vi "Motor driving.vi"(9 "New direction":string, 11 "Current direction":string) -> ()   [LabVIEW 2015]
uses:
  <vilib>/Platform/TimedLoop/XDataNode/timing_clust.ctl
  <vilib>/Platform/TimedLoop/XDataNode/nitl_modes.ctl
  <vilib>/Platform/TimedLoop/XDataNode/wakeup.ctl
  <vilib>/myRIO/Instrument Drivers/Onboard IO/PWM/typedefs/PWM Reference.ctl
  <vilib>/myRIO/Common/Instrument Driver Framework/Utilities/typedefs/myRIO Generic Hardware Reference.ctl
  <vilib>/myRIO/Common/Instrument Driver Framework/Utilities/typedefs/Hardware Version Enum.ctl
  <vilib>/myRIO/Common/Instrument Driver Framework/Utilities/typedefs/myRIO v1.0 Reference.ctl
  <vilib>/myRIO/Common/Instrument Driver Framework/Utilities/typedefs/Generic FPGA Reference.ctl
  <vilib>/myRIO/Common/Instrument Driver Framework/myRIO v1.0/PWM/typedefs/PWM Channels Enum.ctl
  <vilib>/myRIO/Instrument Drivers/Onboard IO/PWM/typedefs/PWM Configuration.ctl
  <vilib>/userdefined/High Color/nirio_resource_hc.ctl
  <vilib>/myRIO/Common/Instrument Driver Framework/Utilities/vis/Is FPGA Ref Available.vi
  <vilib>/myRIO/Common/Instrument Driver Framework/myRIO v1.0/PWM/vis/myRIO v1.1 Open PWM.vi
  <vilib>/myRIO/Instrument Drivers/Onboard IO/PWM/vis/Set Duty Cycle and Frequency.vi
  <vilib>/myRIO/Common/Instrument Driver Framework/Utilities/vis/Validate Channels.vi
  <vilib>/myRIO/Common/Instrument Driver Framework/myRIO v1.0/PWM/vis/myRIO v1.0 Reserve PWM.vi
  <vilib>/myRIO/Common/Instrument Driver Framework/myRIO v1.0/PWM/vis/myRIO v1.0 Build MUX Configuration PWM.vi
  <vilib>/myRIO/Common/Instrument Driver Framework/myRIO v1.0/Resource Manager/vis/myRIO v1.0 Reserve Channel List.vi
  <vilib>/myRIO/Common/Instrument Driver Framework/myRIO v1.0/Resource Manager/vis/myRIO v1.0 Create Configuration List.vi
  <vilib>/myRIO/Common/Instrument Driver Framework/myRIO v1.0/Resource Manager/vis/myRIO v1.0 Reserve Channel.vi
  <vilib>/myRIO/Common/Instrument Driver Framework/myRIO v1.0/Resource Manager/vis/myRIO v1.0 Unreserve Channel.vi
  <vilib>/myRIO/Common/Instrument Driver Framework/myRIO v1.0/Resource Manager/vis/myRIO v1.0 Build Mutex Name.vi
  <vilib>/Utility/VariantDataType/GetNumericInfo.vi
  <vilib>/Utility/error.llb/Error Cluster From Error Code.vi
  <vilib>/myRIO/Common/Instrument Driver Framework/myRIO v1.0/myRIO v1.1 Open.vi
  <vilib>/myRIO/Common/Instrument Driver Framework/Utilities/vis/IO Manager.vi
  <vilib>/myRIO/Common/Instrument Driver Framework/Utilities/vis/Configuration Manager.vi
  <vilib>/myRIO/Common/Instrument Driver Framework/myRIO v1.0/Resource Manager/vis/myRIO v1.0 Configure IO.vi
  <vilib>/myRIO/Common/Instrument Driver Framework/myRIO v1.0/myRIO v1.0 Close.vi
  <vilib>/myRIO/Common/Instrument Driver Framework/myRIO v1.0/PWM/vis/myRIO v1.0 Write PWM.vi
  <vilib>/platform/TimedLoop/XDataNode/XDataNode.xnode
  <vilib>/myRIO/Express VI/Onboard IO/PWM/PWM Express VI.xnode
  <vilib>/myRIO/Instrument Drivers/Onboard IO/PWM/vis/myRIO PWM Open.xnode
  <vilib>/Platform/TimedLoop/XDataNode/XDNodeRunTimeDep.lvlib
  <vilib>/myRIO/Instrument Drivers/Onboard IO/PWM/PWM.lvlib
panel:
  in  "Array":string[](array[string])
  out "left sped/right speed/time":dbl[][](array[numeric])
  out "Right":dbl=0.85
  out "Left":dbl=0.65
  out "Time":i32=2000
  out "error out 3":errorcluster
  out "error out 2":errorcluster
  in  "error in (no error) 2":errorcluster
  in  "error in (no error)":errorcluster
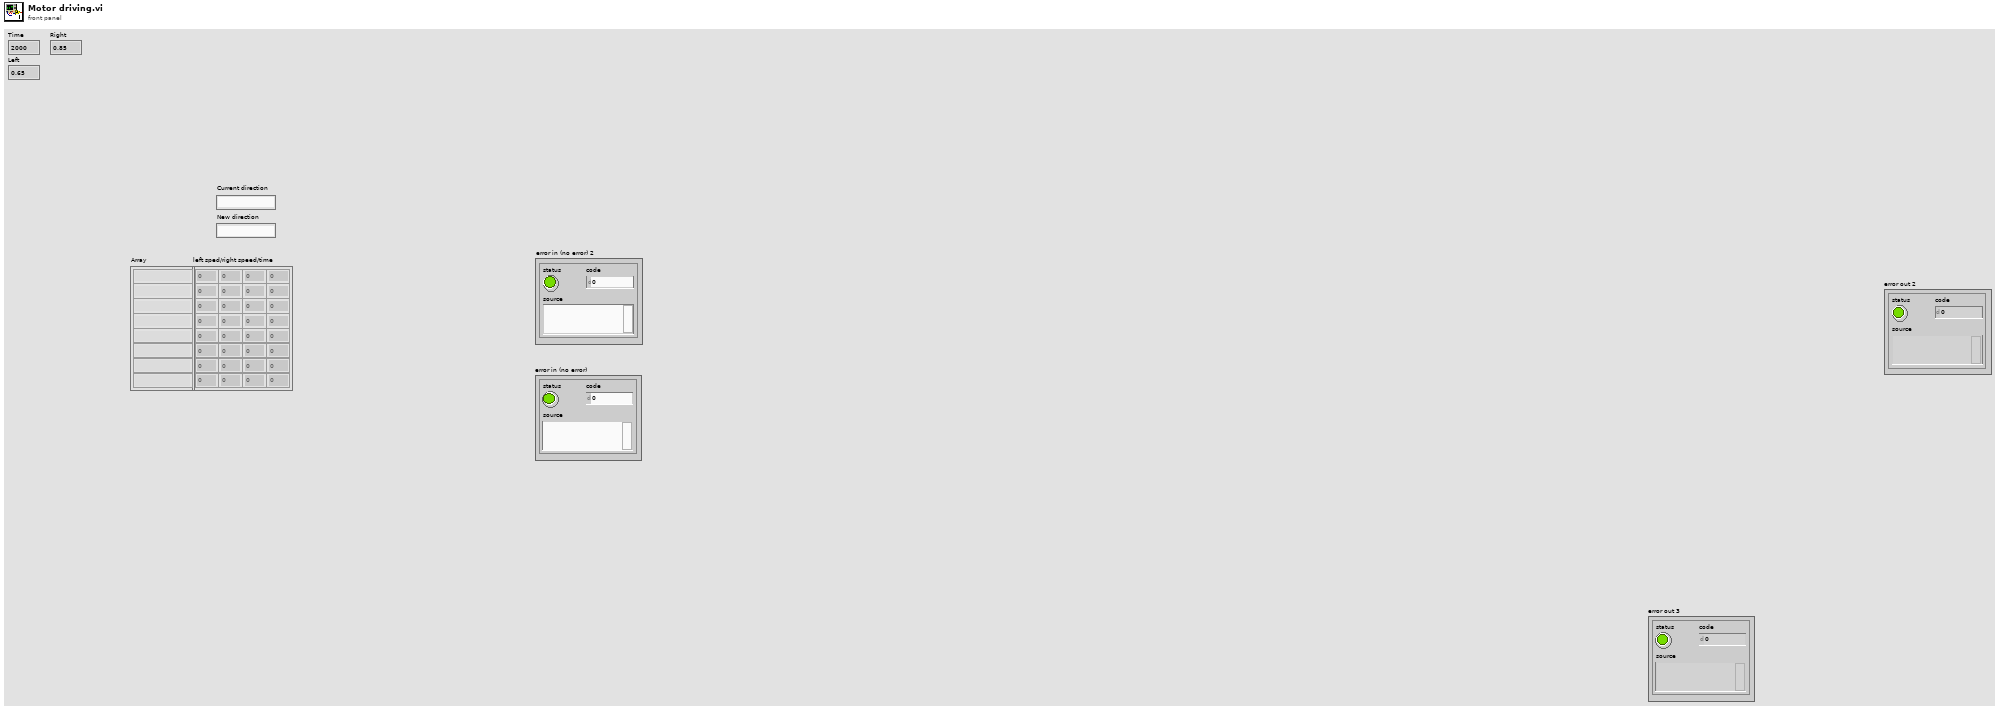
[diagram p1: front panel]
types:
  T1 = typedef "XDNodeRunTimeDep.lvlib/timing_clust.ctl" = cluster{"Expected End [f-1]":u64, "Actual End [f-1]":u64, "Finished Late? [f-1]":bool, "Expected End [i-1]":u64, "Actual End [i-1]":u64, "Finished Late? [i-1]":bool, "Expected Start [i]":u64, "Actual Start [i]":u64, "Expected Start [f]":u64, "Actual Start [f]":u64, "Source Name":string, "Structure Name":string, "Period":i64, "Deadline":i64, "Offset":i64, "Start":i64, "Priority":i32, "Timeout":i32, "Mode":T2, "Wakeup Reason":T3, "Error":errorcluster, "Source Type":string, "Secondary Source Type":string, "Global End Time":u64, "Global Start Time":u64, "Frame Duration":u64, "Iteration Duration":u64, "Assigned CPU":i32, "I/O Scan Engine Mode":u32}
  T2 = typedef "XDNodeRunTimeDep.lvlib/nitl_modes.ctl" = enum32{"No Change", "Process missed periods, maintain original phase", "Discard missed periods, maintain original phase", "Process missed periods, ignore original phase", "Discard missed periods, ignore original phase"}
  T3 = typedef "XDNodeRunTimeDep.lvlib/wakeup.ctl" = enum32{"Normal", "Aborted", "Asynchronous wakeup", "Timing source error", "Timed loop error", "Timeout"}
  T4 = typedef "PWM.lvlib/PWM Reference.ctl" = cluster{"myRIO Reference":T5, "PWM Channels Enum":T9, "PWM Configuration":T10}
  T5 = typedef "myRIO Generic Hardware Reference.ctl" = cluster{"myRIO Model":T6, "myRIO Hardware Reference":T7}
  T6 = typedef "Hardware Version Enum.ctl" = enum16{"Unknown", "myRIO-1900", "myRIO-1950", "roboRIO"}
  T7 = typedef "myRIO v1.0 Reference.ctl" = cluster{"Generic FPGA Reference":T8, "Allow multiple opens":bool}
  T8 = typedef "Generic FPGA Reference.ctl" = refnum<k20>
  T9 = typedef "PWM Channels Enum.ctl" = enum16{"Not Connected", "C/PWM0", "C/PWM1", "A/PWM0", "A/PWM1", "A/PWM2", "B/PWM0", "B/PWM1", "B/PWM2", "PWM/PWM0", "PWM/PWM1", "PWM/PWM2", "PWM/PWM3", "PWM/PWM4", "PWM/PWM5", "PWM/PWM6", "PWM/PWM7", "PWM/PWM8", "PWM/PWM9"}
  T10 = typedef "PWM.lvlib/PWM Configuration.ctl" = cluster{"Frequency":dbl, "Duty Cycle":dbl}
  T11 = typedef "nirio_resource_hc.ctl" = tag
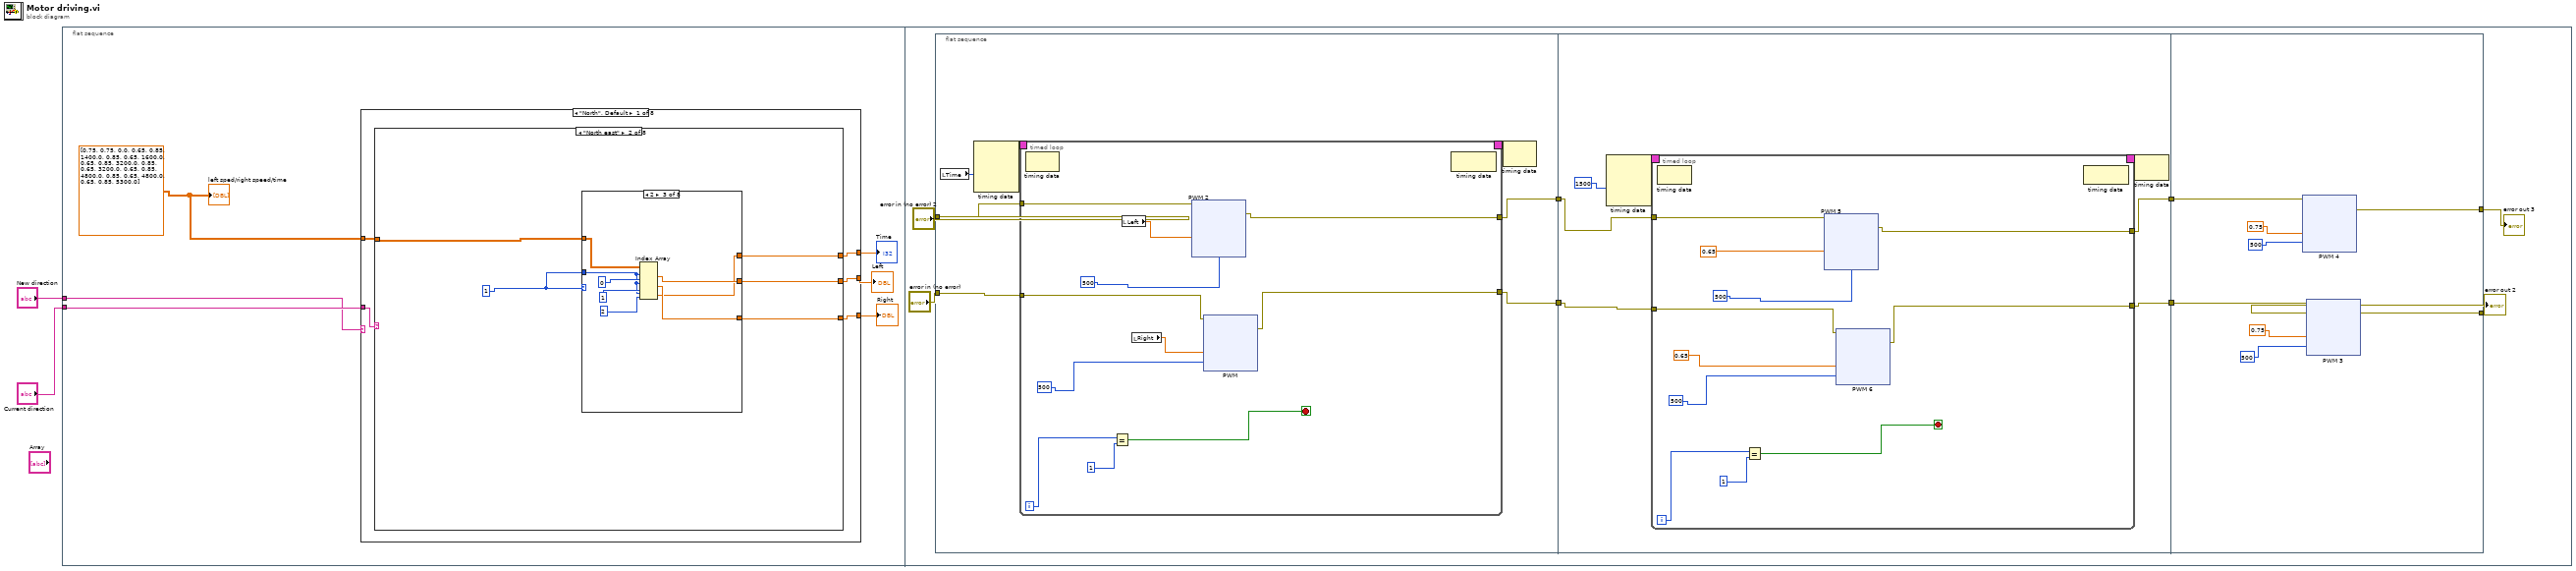
[diagram p0: block diagram]
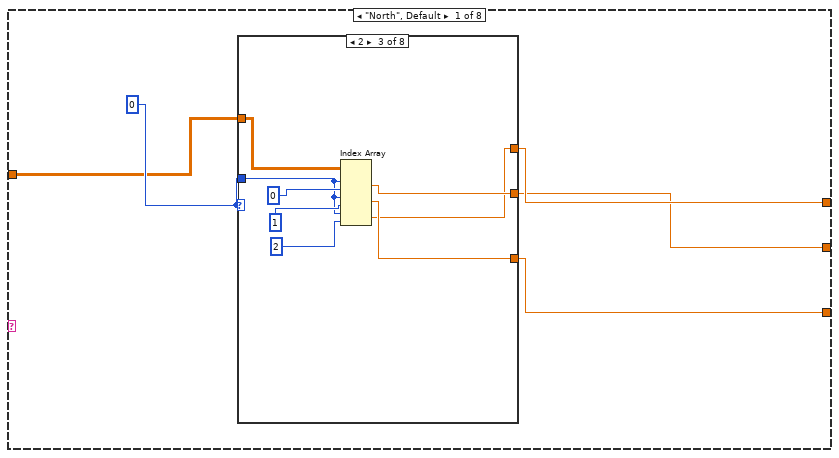
[diagram p2: hidden frame]
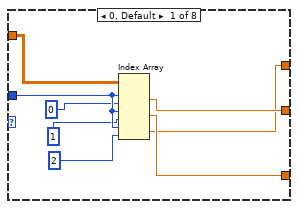
[diagram p3: hidden frame]
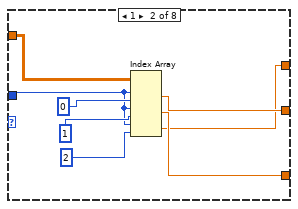
[diagram p4: hidden frame]
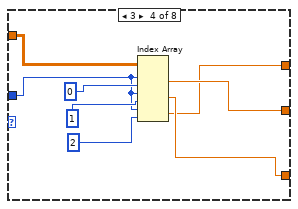
[diagram p5: hidden frame]
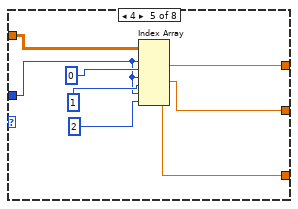
[diagram p6: hidden frame]
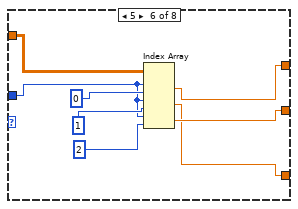
[diagram p7: hidden frame]
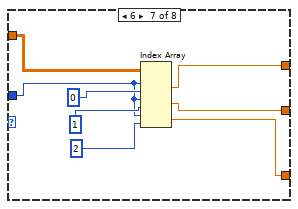
[diagram p8: hidden frame]
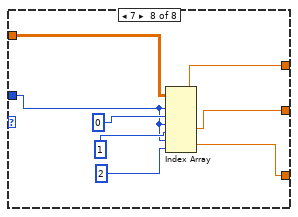
[diagram p9: hidden frame]
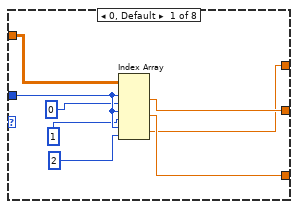
[diagram p10: hidden frame]
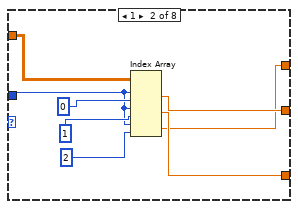
[diagram p11: hidden frame]
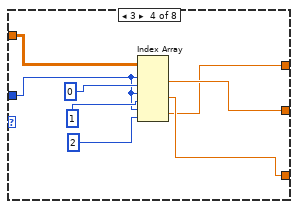
[diagram p12: hidden frame]
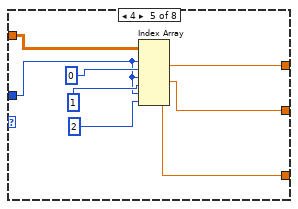
[diagram p13: hidden frame]
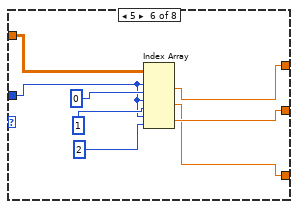
[diagram p14: hidden frame]
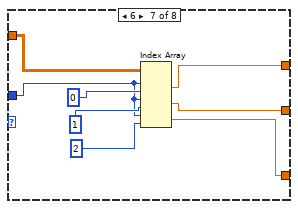
[diagram p15: hidden frame]
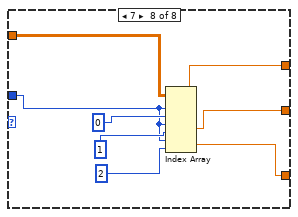
[diagram p16: hidden frame]
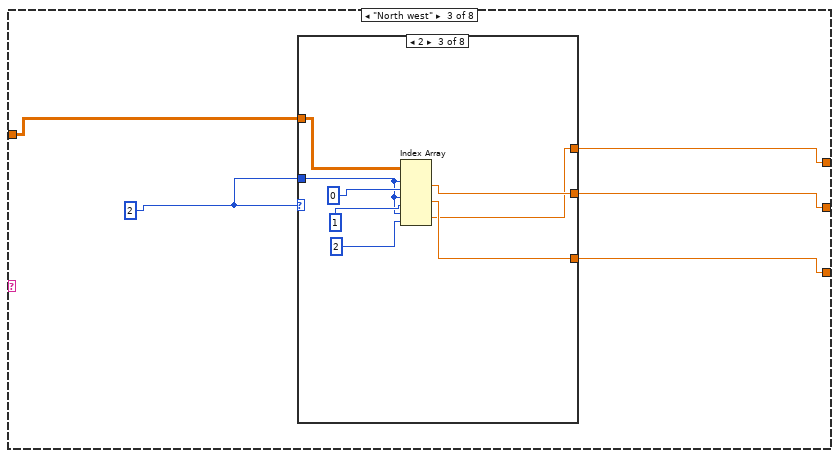
[diagram p17: hidden frame]
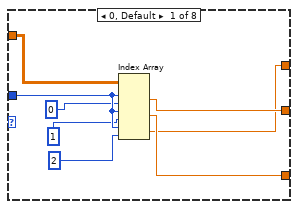
[diagram p18: hidden frame]
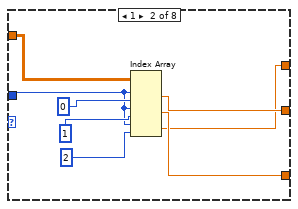
[diagram p19: hidden frame]
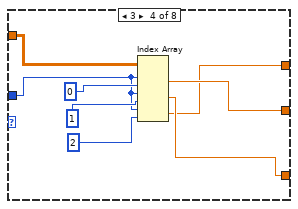
[diagram p20: hidden frame]
diagram:
  n1 = flat-sequence {
    tunnel: "Current direction" -> [w4]
    tunnel: "New direction" -> [w3]
    frame #0 {
      w5 = dbl[][] [[0.75, 0.75, 0.0], [0.65, 0.85, 1400.0], [0.85, 0.65, 1600.0], [0.65, 0.85, 3200.0], [0.85, 0.65, 3200.0], [0.65, 0.85, 4800.0], [0.85, 0.65, 4800.0], [0.65, 0.85, 5300.0]]
      n2 = case shown="\"North\", Default" w3 {
        tunnel: w4 -> [w9 w570 w1127 w1684 w2240 w2797 w3354 w3911]
        tunnel: [w12 w568 w1125 w1682 w2239 w2796 w3353 w3910] -> w8
        tunnel: [w11 w567 w1124 w1681 w2238 w2795 w3352 w3909] -> w7
        tunnel: [w10 w566 w1123 w1680 w2237 w2794 w3351 w3908] -> w6
        tunnel: w5 -> [w13 w569 w1126 w1683 w2241 w2798 w3355 w3912]
        frame "North", Default {
          n3 = case shown="\"North east\"" w9 {
            tunnel: [w17 w87 w155 w222 w292 w362 w430 w500] -> w12
            tunnel: [w16 w86 w154 w223 w291 w360 w429 w499] -> w11
            tunnel: [w15 w85 w153 w221 w290 w359 w428 w498] -> w10
            tunnel: w13 -> [w14 w83 w152 w224 w293 w361 w431 w497]
            frame "North", Default {
              w18 = 0
              n4 = case shown="2" w18 {
                tunnel: [w22 w28 w36 w44 w52 w61 w68 w77] -> w17
                tunnel: [w24 w30 w38 w45 w54 w63 w70 w79] -> w16
                tunnel: [w23 w29 w37 w46 w53 w62 w69 w78] -> w15
                tunnel: w18 -> [w26 w31 w39 w47 w55 w60 w71 w76]
                tunnel: w14 -> [w19 w27 w35 w43 w51 w59 w67 w75]
                frame 0, Default {
                  n5 = Index Array(array=w19, index (row) #1=w26, index (col) #1=0, index (row) #2=w26, index (col) #2=1, index (row) #3=w26, index (col) #3=2) -> (element #1=w24:dbl, element #2=w23:dbl, element #3=w22:dbl)
                }
                frame 1 {
                  n6 = Index Array(array=w27, index (row) #1=w31, index (col) #1=0, index (row) #2=w31, index (col) #2=1, index (row) #3=w31, index (col) #3=2) -> (element #1=w30:dbl, element #2=w29:dbl, element #3=w28:dbl)
                }
                frame 2 {
                  n7 = Index Array(array=w35, index (row) #1=w39, index (col) #1=0, index (row) #2=w39, index (col) #2=1, index (row) #3=w39, index (col) #3=2) -> (element #1=w38:dbl, element #2=w37:dbl, element #3=w36:dbl)
                }
                frame 3 {
                  n8 = Index Array(array=w43, index (row) #1=w47, index (col) #1=0, index (row) #2=w47, index (col) #2=1, index (row) #3=w47, index (col) #3=2) -> (element #1=w45:dbl, element #2=w46:dbl, element #3=w44:dbl)
                }
                frame 4 {
                  n9 = Index Array(array=w51, index (row) #1=w55, index (col) #1=0, index (row) #2=w55, index (col) #2=1, index (row) #3=w55, index (col) #3=2) -> (element #1=w52:dbl, element #2=w54:dbl, element #3=w53:dbl)
                }
                frame 5 {
                  n10 = Index Array(array=w59, index (row) #1=w60, index (col) #1=0, index (row) #2=w60, index (col) #2=1, index (row) #3=w60, index (col) #3=2) -> (element #1=w61:dbl, element #2=w62:dbl, element #3=w63:dbl)
                }
                frame 6 {
                  n11 = Index Array(array=w67, index (row) #1=w71, index (col) #1=0, index (row) #2=w71, index (col) #2=1, index (row) #3=w71, index (col) #3=2) -> (element #1=w68:dbl, element #2=w70:dbl, element #3=w69:dbl)
                }
                frame 7 {
                  n12 = Index Array(array=w75, index (row) #1=w76, index (col) #1=0, index (row) #2=w76, index (col) #2=1, index (row) #3=w76, index (col) #3=2) -> (element #1=w77:dbl, element #2=w79:dbl, element #3=w78:dbl)
                }
              }
            }
            frame "North east" {
              w84 = 1
              n13 = case shown="2" w84 {
                tunnel: [w91 w97 w105 w113 w121 w130 w137 w146] -> w87
                tunnel: [w93 w99 w107 w114 w123 w132 w139 w148] -> w86
                tunnel: [w92 w98 w106 w115 w122 w131 w138 w147] -> w85
                tunnel: w84 -> [w95 w100 w108 w116 w124 w129 w140 w145]
                tunnel: w83 -> [w88 w96 w104 w112 w120 w128 w136 w144]
                frame 0, Default {
                  n14 = Index Array(array=w88, index (row) #1=w95, index (col) #1=0, index (row) #2=w95, index (col) #2=1, index (row) #3=w95, index (col) #3=2) -> (element #1=w93:dbl, element #2=w92:dbl, element #3=w91:dbl)
                }
                frame 1 {
                  n15 = Index Array(array=w96, index (row) #1=w100, index (col) #1=0, index (row) #2=w100, index (col) #2=1, index (row) #3=w100, index (col) #3=2) -> (element #1=w99:dbl, element #2=w98:dbl, element #3=w97:dbl)
                }
                frame 2 {
                  n16 = Index Array(array=w104, index (row) #1=w108, index (col) #1=0, index (row) #2=w108, index (col) #2=1, index (row) #3=w108, index (col) #3=2) -> (element #1=w107:dbl, element #2=w106:dbl, element #3=w105:dbl)
                }
                frame 3 {
                  n17 = Index Array(array=w112, index (row) #1=w116, index (col) #1=0, index (row) #2=w116, index (col) #2=1, index (row) #3=w116, index (col) #3=2) -> (element #1=w114:dbl, element #2=w115:dbl, element #3=w113:dbl)
                }
                frame 4 {
                  n18 = Index Array(array=w120, index (row) #1=w124, index (col) #1=0, index (row) #2=w124, index (col) #2=1, index (row) #3=w124, index (col) #3=2) -> (element #1=w121:dbl, element #2=w123:dbl, element #3=w122:dbl)
                }
                frame 5 {
                  n19 = Index Array(array=w128, index (row) #1=w129, index (col) #1=0, index (row) #2=w129, index (col) #2=1, index (row) #3=w129, index (col) #3=2) -> (element #1=w130:dbl, element #2=w131:dbl, element #3=w132:dbl)
                }
                frame 6 {
                  n20 = Index Array(array=w136, index (row) #1=w140, index (col) #1=0, index (row) #2=w140, index (col) #2=1, index (row) #3=w140, index (col) #3=2) -> (element #1=w137:dbl, element #2=w139:dbl, element #3=w138:dbl)
                }
                frame 7 {
                  n21 = Index Array(array=w144, index (row) #1=w145, index (col) #1=0, index (row) #2=w145, index (col) #2=1, index (row) #3=w145, index (col) #3=2) -> (element #1=w146:dbl, element #2=w148:dbl, element #3=w147:dbl)
                }
              }
            }
            frame "North west" {
              w156 = 2
              n22 = case shown="2" w156 {
                tunnel: [w160 w166 w174 w182 w190 w199 w206 w215] -> w155
                tunnel: [w162 w168 w176 w183 w192 w201 w208 w217] -> w154
                tunnel: [w161 w167 w175 w184 w191 w200 w207 w216] -> w153
                tunnel: w156 -> [w164 w169 w177 w185 w193 w198 w209 w214]
                tunnel: w152 -> [w157 w165 w173 w181 w189 w197 w205 w213]
                frame 0, Default {
                  n23 = Index Array(array=w157, index (row) #1=w164, index (col) #1=0, index (row) #2=w164, index (col) #2=1, index (row) #3=w164, index (col) #3=2) -> (element #1=w162:dbl, element #2=w161:dbl, element #3=w160:dbl)
                }
                frame 1 {
                  n24 = Index Array(array=w165, index (row) #1=w169, index (col) #1=0, index (row) #2=w169, index (col) #2=1, index (row) #3=w169, index (col) #3=2) -> (element #1=w168:dbl, element #2=w167:dbl, element #3=w166:dbl)
                }
                frame 2 {
                  n25 = Index Array(array=w173, index (row) #1=w177, index (col) #1=0, index (row) #2=w177, index (col) #2=1, index (row) #3=w177, index (col) #3=2) -> (element #1=w176:dbl, element #2=w175:dbl, element #3=w174:dbl)
                }
                frame 3 {
                  n26 = Index Array(array=w181, index (row) #1=w185, index (col) #1=0, index (row) #2=w185, index (col) #2=1, index (row) #3=w185, index (col) #3=2) -> (element #1=w183:dbl, element #2=w184:dbl, element #3=w182:dbl)
                }
                frame 4 {
                  n27 = Index Array(array=w189, index (row) #1=w193, index (col) #1=0, index (row) #2=w193, index (col) #2=1, index (row) #3=w193, index (col) #3=2) -> (element #1=w190:dbl, element #2=w192:dbl, element #3=w191:dbl)
                }
                frame 5 {
                  n28 = Index Array(array=w197, index (row) #1=w198, index (col) #1=0, index (row) #2=w198, index (col) #2=1, index (row) #3=w198, index (col) #3=2) -> (element #1=w199:dbl, element #2=w200:dbl, element #3=w201:dbl)
                }
                frame 6 {
                  n29 = Index Array(array=w205, index (row) #1=w209, index (col) #1=0, index (row) #2=w209, index (col) #2=1, index (row) #3=w209, index (col) #3=2) -> (element #1=w206:dbl, element #2=w208:dbl, element #3=w207:dbl)
                }
                frame 7 {
                  n30 = Index Array(array=w213, index (row) #1=w214, index (col) #1=0, index (row) #2=w214, index (col) #2=1, index (row) #3=w214, index (col) #3=2) -> (element #1=w215:dbl, element #2=w217:dbl, element #3=w216:dbl)
                }
              }
            }
            frame "West" {
              w225 = 4
              n31 = case shown="2" w225 {
                tunnel: [w229 w235 w243 w251 w259 w268 w275 w284] -> w222
                tunnel: [w231 w237 w245 w252 w261 w270 w277 w286] -> w223
                tunnel: [w230 w236 w244 w253 w260 w269 w276 w285] -> w221
                tunnel: w225 -> [w233 w238 w246 w254 w262 w267 w278 w283]
                tunnel: w224 -> [w226 w234 w242 w250 w258 w266 w274 w282]
                frame 0, Default {
                  n32 = Index Array(array=w226, index (row) #1=w233, index (col) #1=0, index (row) #2=w233, index (col) #2=1, index (row) #3=w233, index (col) #3=2) -> (element #1=w231:dbl, element #2=w230:dbl, element #3=w229:dbl)
                }
                frame 1 {
                  n33 = Index Array(array=w234, index (row) #1=w238, index (col) #1=0, index (row) #2=w238, index (col) #2=1, index (row) #3=w238, index (col) #3=2) -> (element #1=w237:dbl, element #2=w236:dbl, element #3=w235:dbl)
                }
                frame 2 {
                  n34 = Index Array(array=w242, index (row) #1=w246, index (col) #1=0, index (row) #2=w246, index (col) #2=1, index (row) #3=w246, index (col) #3=2) -> (element #1=w245:dbl, element #2=w244:dbl, element #3=w243:dbl)
                }
                frame 3 {
                  n35 = Index Array(array=w250, index (row) #1=w254, index (col) #1=0, index (row) #2=w254, index (col) #2=1, index (row) #3=w254, index (col) #3=2) -> (element #1=w252:dbl, element #2=w253:dbl, element #3=w251:dbl)
                }
                frame 4 {
                  n36 = Index Array(array=w258, index (row) #1=w262, index (col) #1=0, index (row) #2=w262, index (col) #2=1, index (row) #3=w262, index (col) #3=2) -> (element #1=w259:dbl, element #2=w261:dbl, element #3=w260:dbl)
                }
                frame 5 {
                  n37 = Index Array(array=w266, index (row) #1=w267, index (col) #1=0, index (row) #2=w267, index (col) #2=1, index (row) #3=w267, index (col) #3=2) -> (element #1=w268:dbl, element #2=w269:dbl, element #3=w270:dbl)
                }
                frame 6 {
                  n38 = Index Array(array=w274, index (row) #1=w278, index (col) #1=0, index (row) #2=w278, index (col) #2=1, index (row) #3=w278, index (col) #3=2) -> (element #1=w275:dbl, element #2=w277:dbl, element #3=w276:dbl)
                }
                frame 7 {
                  n39 = Index Array(array=w282, index (row) #1=w283, index (col) #1=0, index (row) #2=w283, index (col) #2=1, index (row) #3=w283, index (col) #3=2) -> (element #1=w284:dbl, element #2=w286:dbl, element #3=w285:dbl)
                }
              }
            }
            frame "East" {
              w294 = 3
              n40 = case shown="2" w294 {
                tunnel: [w298 w304 w312 w320 w328 w337 w344 w353] -> w292
                tunnel: [w300 w306 w314 w321 w330 w339 w346 w355] -> w291
                tunnel: [w299 w305 w313 w322 w329 w338 w345 w354] -> w290
                tunnel: w294 -> [w302 w307 w315 w323 w331 w336 w347 w352]
                tunnel: w293 -> [w295 w303 w311 w319 w327 w335 w343 w351]
                frame 0, Default {
                  n41 = Index Array(array=w295, index (row) #1=w302, index (col) #1=0, index (row) #2=w302, index (col) #2=1, index (row) #3=w302, index (col) #3=2) -> (element #1=w300:dbl, element #2=w299:dbl, element #3=w298:dbl)
                }
                frame 1 {
                  n42 = Index Array(array=w303, index (row) #1=w307, index (col) #1=0, index (row) #2=w307, index (col) #2=1, index (row) #3=w307, index (col) #3=2) -> (element #1=w306:dbl, element #2=w305:dbl, element #3=w304:dbl)
                }
                frame 2 {
                  n43 = Index Array(array=w311, index (row) #1=w315, index (col) #1=0, index (row) #2=w315, index (col) #2=1, index (row) #3=w315, index (col) #3=2) -> (element #1=w314:dbl, element #2=w313:dbl, element #3=w312:dbl)
                }
                frame 3 {
                  n44 = Index Array(array=w319, index (row) #1=w323, index (col) #1=0, index (row) #2=w323, index (col) #2=1, index (row) #3=w323, index (col) #3=2) -> (element #1=w321:dbl, element #2=w322:dbl, element #3=w320:dbl)
                }
                frame 4 {
                  n45 = Index Array(array=w327, index (row) #1=w331, index (col) #1=0, index (row) #2=w331, index (col) #2=1, index (row) #3=w331, index (col) #3=2) -> (element #1=w328:dbl, element #2=w330:dbl, element #3=w329:dbl)
                }
                frame 5 {
                  n46 = Index Array(array=w335, index (row) #1=w336, index (col) #1=0, index (row) #2=w336, index (col) #2=1, index (row) #3=w336, index (col) #3=2) -> (element #1=w337:dbl, element #2=w338:dbl, element #3=w339:dbl)
                }
                frame 6 {
                  n47 = Index Array(array=w343, index (row) #1=w347, index (col) #1=0, index (row) #2=w347, index (col) #2=1, index (row) #3=w347, index (col) #3=2) -> (element #1=w344:dbl, element #2=w346:dbl, element #3=w345:dbl)
                }
                frame 7 {
                  n48 = Index Array(array=w351, index (row) #1=w352, index (col) #1=0, index (row) #2=w352, index (col) #2=1, index (row) #3=w352, index (col) #3=2) -> (element #1=w353:dbl, element #2=w355:dbl, element #3=w354:dbl)
                }
              }
            }
            frame "South" {
              w363 = 7
              n49 = case shown="2" w363 {
                tunnel: [w367 w373 w381 w389 w397 w406 w413 w422] -> w362
                tunnel: [w369 w375 w383 w390 w399 w408 w415 w424] -> w360
                tunnel: [w368 w374 w382 w391 w398 w407 w414 w423] -> w359
                tunnel: w363 -> [w371 w376 w384 w392 w400 w405 w416 w421]
                tunnel: w361 -> [w364 w372 w380 w388 w396 w404 w412 w420]
                frame 0, Default {
                  n50 = Index Array(array=w364, index (row) #1=w371, index (col) #1=0, index (row) #2=w371, index (col) #2=1, index (row) #3=w371, index (col) #3=2) -> (element #1=w369:dbl, element #2=w368:dbl, element #3=w367:dbl)
                }
                frame 1 {
                  n51 = Index Array(array=w372, index (row) #1=w376, index (col) #1=0, index (row) #2=w376, index (col) #2=1, index (row) #3=w376, index (col) #3=2) -> (element #1=w375:dbl, element #2=w374:dbl, element #3=w373:dbl)
                }
                frame 2 {
                  n52 = Index Array(array=w380, index (row) #1=w384, index (col) #1=0, index (row) #2=w384, index (col) #2=1, index (row) #3=w384, index (col) #3=2) -> (element #1=w383:dbl, element #2=w382:dbl, element #3=w381:dbl)
                }
                frame 3 {
                  n53 = Index Array(array=w388, index (row) #1=w392, index (col) #1=0, index (row) #2=w392, index (col) #2=1, index (row) #3=w392, index (col) #3=2) -> (element #1=w390:dbl, element #2=w391:dbl, element #3=w389:dbl)
                }
                frame 4 {
                  n54 = Index Array(array=w396, index (row) #1=w400, index (col) #1=0, index (row) #2=w400, index (col) #2=1, index (row) #3=w400, index (col) #3=2) -> (element #1=w397:dbl, element #2=w399:dbl, element #3=w398:dbl)
                }
                frame 5 {
                  n55 = Index Array(array=w404, index (row) #1=w405, index (col) #1=0, index (row) #2=w405, index (col) #2=1, index (row) #3=w405, index (col) #3=2) -> (element #1=w406:dbl, element #2=w407:dbl, element #3=w408:dbl)
                }
                frame 6 {
                  n56 = Index Array(array=w412, index (row) #1=w416, index (col) #1=0, index (row) #2=w416, index (col) #2=1, index (row) #3=w416, index (col) #3=2) -> (element #1=w413:dbl, element #2=w415:dbl, element #3=w414:dbl)
                }
                frame 7 {
                  n57 = Index Array(array=w420, index (row) #1=w421, index (col) #1=0, index (row) #2=w421, index (col) #2=1, index (row) #3=w421, index (col) #3=2) -> (element #1=w422:dbl, element #2=w424:dbl, element #3=w423:dbl)
                }
              }
            }
            frame "South west" {
              w432 = 6
              n58 = case shown="2" w432 {
                tunnel: [w436 w442 w450 w458 w466 w475 w482 w491] -> w430
                tunnel: [w438 w444 w452 w459 w468 w477 w484 w493] -> w429
                tunnel: [w437 w443 w451 w460 w467 w476 w483 w492] -> w428
                tunnel: w432 -> [w440 w445 w453 w461 w469 w474 w485 w490]
                tunnel: w431 -> [w433 w441 w449 w457 w465 w473 w481 w489]
                frame 0, Default {
                  n59 = Index Array(array=w433, index (row) #1=w440, index (col) #1=0, index (row) #2=w440, index (col) #2=1, index (row) #3=w440, index (col) #3=2) -> (element #1=w438:dbl, element #2=w437:dbl, element #3=w436:dbl)
                }
                frame 1 {
                  n60 = Index Array(array=w441, index (row) #1=w445, index (col) #1=0, index (row) #2=w445, index (col) #2=1, index (row) #3=w445, index (col) #3=2) -> (element #1=w444:dbl, element #2=w443:dbl, element #3=w442:dbl)
                }
                frame 2 {
                  n61 = Index Array(array=w449, index (row) #1=w453, index (col) #1=0, index (row) #2=w453, index (col) #2=1, index (row) #3=w453, index (col) #3=2) -> (element #1=w452:dbl, element #2=w451:dbl, element #3=w450:dbl)
                }
                frame 3 {
                  n62 = Index Array(array=w457, index (row) #1=w461, index (col) #1=0, index (row) #2=w461, index (col) #2=1, index (row) #3=w461, index (col) #3=2) -> (element #1=w459:dbl, element #2=w460:dbl, element #3=w458:dbl)
                }
                frame 4 {
                  n63 = Index Array(array=w465, index (row) #1=w469, index (col) #1=0, index (row) #2=w469, index (col) #2=1, index (row) #3=w469, index (col) #3=2) -> (element #1=w466:dbl, element #2=w468:dbl, element #3=w467:dbl)
                }
                frame 5 {
                  n64 = Index Array(array=w473, index (row) #1=w474, index (col) #1=0, index (row) #2=w474, index (col) #2=1, index (row) #3=w474, index (col) #3=2) -> (element #1=w475:dbl, element #2=w476:dbl, element #3=w477:dbl)
                }
                frame 6 {
                  n65 = Index Array(array=w481, index (row) #1=w485, index (col) #1=0, index (row) #2=w485, index (col) #2=1, index (row) #3=w485, index (col) #3=2) -> (element #1=w482:dbl, element #2=w484:dbl, element #3=w483:dbl)
                }
                frame 7 {
                  n66 = Index Array(array=w489, index (row) #1=w490, index (col) #1=0, index (row) #2=w490, index (col) #2=1, index (row) #3=w490, index (col) #3=2) -> (element #1=w491:dbl, element #2=w493:dbl, element #3=w492:dbl)
                }
              }
            }
            frame "South east" {
              w501 = 5
              n67 = case shown="2" w501 {
                tunnel: [w505 w511 w519 w527 w535 w544 w551 w560] -> w500
                tunnel: [w507 w513 w521 w528 w537 w546 w553 w562] -> w499
                tunnel: [w506 w512 w520 w529 w536 w545 w552 w561] -> w498
                tunnel: w501 -> [w509 w514 w522 w530 w538 w543 w554 w559]
                tunnel: w497 -> [w502 w510 w518 w526 w534 w542 w550 w558]
                frame 0, Default {
                  n68 = Index Array(array=w502, index (row) #1=w509, index (col) #1=0, index (row) #2=w509, index (col) #2=1, index (row) #3=w509, index (col) #3=2) -> (element #1=w507:dbl, element #2=w506:dbl, element #3=w505:dbl)
                }
                frame 1 {
                  n69 = Index Array(array=w510, index (row) #1=w514, index (col) #1=0, index (row) #2=w514, index (col) #2=1, index (row) #3=w514, index (col) #3=2) -> (element #1=w513:dbl, element #2=w512:dbl, element #3=w511:dbl)
                }
                frame 2 {
                  n70 = Index Array(array=w518, index (row) #1=w522, index (col) #1=0, index (row) #2=w522, index (col) #2=1, index (row) #3=w522, index (col) #3=2) -> (element #1=w521:dbl, element #2=w520:dbl, element #3=w519:dbl)
                }
                frame 3 {
                  n71 = Index Array(array=w526, index (row) #1=w530, index (col) #1=0, index (row) #2=w530, index (col) #2=1, index (row) #3=w530, index (col) #3=2) -> (element #1=w528:dbl, element #2=w529:dbl, element #3=w527:dbl)
                }
                frame 4 {
                  n72 = Index Array(array=w534, index (row) #1=w538, index (col) #1=0, index (row) #2=w538, index (col) #2=1, index (row) #3=w538, index (col) #3=2) -> (element #1=w535:dbl, element #2=w537:dbl, element #3=w536:dbl)
                }
                frame 5 {
                  n73 = Index Array(array=w542, index (row) #1=w543, index (col) #1=0, index (row) #2=w543, index (col) #2=1, index (row) #3=w543, index (col) #3=2) -> (element #1=w544:dbl, element #2=w545:dbl, element #3=w546:dbl)
                }
                frame 6 {
                  n74 = Index Array(array=w550, index (row) #1=w554, index (col) #1=0, index (row) #2=w554, index (col) #2=1, index (row) #3=w554, index (col) #3=2) -> (element #1=w551:dbl, element #2=w553:dbl, element #3=w552:dbl)
                }
                frame 7 {
                  n75 = Index Array(array=w558, index (row) #1=w559, index (col) #1=0, index (row) #2=w559, index (col) #2=1, index (row) #3=w559, index (col) #3=2) -> (element #1=w560:dbl, element #2=w562:dbl, element #3=w561:dbl)
                }
              }
            }
          }
        }
        frame "North east" {
          n76 = case shown="\"North\", Default" w570 {
            tunnel: [w574 w644 w712 w779 w849 w919 w987 w1057] -> w568
            tunnel: [w573 w643 w711 w780 w848 w917 w986 w1056] -> w567
            tunnel: [w572 w642 w710 w778 w847 w916 w985 w1055] -> w566
            tunnel: w569 -> [w571 w640 w709 w781 w850 w918 w988 w1054]
            frame "North", Default {
              w575 = 2
              n77 = case shown="2" w575 {
                tunnel: [w579 w585 w593 w601 w609 w618 w625 w634] -> w574
                tunnel: [w581 w587 w595 w602 w611 w620 w627 w636] -> w573
                tunnel: [w580 w586 w594 w603 w610 w619 w626 w635] -> w572
                tunnel: w575 -> [w583 w588 w596 w604 w612 w617 w628 w633]
                tunnel: w571 -> [w576 w584 w592 w600 w608 w616 w624 w632]
                frame 0, Default {
                  n78 = Index Array(array=w576, index (row) #1=w583, index (col) #1=0, index (row) #2=w583, index (col) #2=1, index (row) #3=w583, index (col) #3=2) -> (element #1=w581:dbl, element #2=w580:dbl, element #3=w579:dbl)
                }
                frame 1 {
                  n79 = Index Array(array=w584, index (row) #1=w588, index (col) #1=0, index (row) #2=w588, index (col) #2=1, index (row) #3=w588, index (col) #3=2) -> (element #1=w587:dbl, element #2=w586:dbl, element #3=w585:dbl)
                }
                frame 2 {
                  n80 = Index Array(array=w592, index (row) #1=w596, index (col) #1=0, index (row) #2=w596, index (col) #2=1, index (row) #3=w596, index (col) #3=2) -> (element #1=w595:dbl, element #2=w594:dbl, element #3=w593:dbl)
                }
                frame 3 {
                  n81 = Index Array(array=w600, index (row) #1=w604, index (col) #1=0, index (row) #2=w604, index (col) #2=1, index (row) #3=w604, index (col) #3=2) -> (element #1=w602:dbl, element #2=w603:dbl, element #3=w601:dbl)
                }
                frame 4 {
                  n82 = Index Array(array=w608, index (row) #1=w612, index (col) #1=0, index (row) #2=w612, index (col) #2=1, index (row) #3=w612, index (col) #3=2) -> (element #1=w609:dbl, element #2=w611:dbl, element #3=w610:dbl)
                }
                frame 5 {
                  n83 = Index Array(array=w616, index (row) #1=w617, index (col) #1=0, index (row) #2=w617, index (col) #2=1, index (row) #3=w617, index (col) #3=2) -> (element #1=w618:dbl, element #2=w619:dbl, element #3=w620:dbl)
                }
                frame 6 {
                  n84 = Index Array(array=w624, index (row) #1=w628, index (col) #1=0, index (row) #2=w628, index (col) #2=1, index (row) #3=w628, index (col) #3=2) -> (element #1=w625:dbl, element #2=w627:dbl, element #3=w626:dbl)
                }
                frame 7 {
                  n85 = Index Array(array=w632, index (row) #1=w633, index (col) #1=0, index (row) #2=w633, index (col) #2=1, index (row) #3=w633, index (col) #3=2) -> (element #1=w634:dbl, element #2=w636:dbl, element #3=w635:dbl)
                }
              }
            }
            frame "North east" {
              w641 = 0
              n86 = case shown="2" w641 {
                tunnel: [w648 w654 w662 w670 w678 w687 w694 w703] -> w644
                tunnel: [w650 w656 w664 w671 w680 w689 w696 w705] -> w643
                tunnel: [w649 w655 w663 w672 w679 w688 w695 w704] -> w642
                tunnel: w641 -> [w652 w657 w665 w673 w681 w686 w697 w702]
                tunnel: w640 -> [w645 w653 w661 w669 w677 w685 w693 w701]
                frame 0, Default {
                  n87 = Index Array(array=w645, index (row) #1=w652, index (col) #1=0, index (row) #2=w652, index (col) #2=1, index (row) #3=w652, index (col) #3=2) -> (element #1=w650:dbl, element #2=w649:dbl, element #3=w648:dbl)
                }
                frame 1 {
                  n88 = Index Array(array=w653, index (row) #1=w657, index (col) #1=0, index (row) #2=w657, index (col) #2=1, index (row) #3=w657, index (col) #3=2) -> (element #1=w656:dbl, element #2=w655:dbl, element #3=w654:dbl)
                }
                frame 2 {
                  n89 = Index Array(array=w661, index (row) #1=w665, index (col) #1=0, index (row) #2=w665, index (col) #2=1, index (row) #3=w665, index (col) #3=2) -> (element #1=w664:dbl, element #2=w663:dbl, element #3=w662:dbl)
                }
                frame 3 {
                  n90 = Index Array(array=w669, index (row) #1=w673, index (col) #1=0, index (row) #2=w673, index (col) #2=1, index (row) #3=w673, index (col) #3=2) -> (element #1=w671:dbl, element #2=w672:dbl, element #3=w670:dbl)
                }
                frame 4 {
                  n91 = Index Array(array=w677, index (row) #1=w681, index (col) #1=0, index (row) #2=w681, index (col) #2=1, index (row) #3=w681, index (col) #3=2) -> (element #1=w678:dbl, element #2=w680:dbl, element #3=w679:dbl)
                }
                frame 5 {
                  n92 = Index Array(array=w685, index (row) #1=w686, index (col) #1=0, index (row) #2=w686, index (col) #2=1, index (row) #3=w686, index (col) #3=2) -> (element #1=w687:dbl, element #2=w688:dbl, element #3=w689:dbl)
                }
                frame 6 {
                  n93 = Index Array(array=w693, index (row) #1=w697, index (col) #1=0, index (row) #2=w697, index (col) #2=1, index (row) #3=w697, index (col) #3=2) -> (element #1=w694:dbl, element #2=w696:dbl, element #3=w695:dbl)
                }
                frame 7 {
                  n94 = Index Array(array=w701, index (row) #1=w702, index (col) #1=0, index (row) #2=w702, index (col) #2=1, index (row) #3=w702, index (col) #3=2) -> (element #1=w703:dbl, element #2=w705:dbl, element #3=w704:dbl)
                }
              }
            }
            frame "North west" {
              w713 = 4
              n95 = case shown="2" w713 {
                tunnel: [w717 w723 w731 w739 w747 w756 w763 w772] -> w712
                tunnel: [w719 w725 w733 w740 w749 w758 w765 w774] -> w711
                tunnel: [w718 w724 w732 w741 w748 w757 w764 w773] -> w710
                tunnel: w713 -> [w721 w726 w734 w742 w750 w755 w766 w771]
                tunnel: w709 -> [w714 w722 w730 w738 w746 w754 w762 w770]
                frame 0, Default {
                  n96 = Index Array(array=w714, index (row) #1=w721, index (col) #1=0, index (row) #2=w721, index (col) #2=1, index (row) #3=w721, index (col) #3=2) -> (element #1=w719:dbl, element #2=w718:dbl, element #3=w717:dbl)
                }
                frame 1 {
                  n97 = Index Array(array=w722, index (row) #1=w726, index (col) #1=0, index (row) #2=w726, index (col) #2=1, index (row) #3=w726, index (col) #3=2) -> (element #1=w725:dbl, element #2=w724:dbl, element #3=w723:dbl)
                }
                frame 2 {
                  n98 = Index Array(array=w730, index (row) #1=w734, index (col) #1=0, index (row) #2=w734, index (col) #2=1, index (row) #3=w734, index (col) #3=2) -> (element #1=w733:dbl, element #2=w732:dbl, element #3=w731:dbl)
                }
                frame 3 {
                  n99 = Index Array(array=w738, index (row) #1=w742, index (col) #1=0, index (row) #2=w742, index (col) #2=1, index (row) #3=w742, index (col) #3=2) -> (element #1=w740:dbl, element #2=w741:dbl, element #3=w739:dbl)
                }
                frame 4 {
                  n100 = Index Array(array=w746, index (row) #1=w750, index (col) #1=0, index (row) #2=w750, index (col) #2=1, index (row) #3=w750, index (col) #3=2) -> (element #1=w747:dbl, element #2=w749:dbl, element #3=w748:dbl)
                }
                frame 5 {
                  n101 = Index Array(array=w754, index (row) #1=w755, index (col) #1=0, index (row) #2=w755, index (col) #2=1, index (row) #3=w755, index (col) #3=2) -> (element #1=w756:dbl, element #2=w757:dbl, element #3=w758:dbl)
                }
                frame 6 {
                  n102 = Index Array(array=w762, index (row) #1=w766, index (col) #1=0, index (row) #2=w766, index (col) #2=1, index (row) #3=w766, index (col) #3=2) -> (element #1=w763:dbl, element #2=w765:dbl, element #3=w764:dbl)
                }
                frame 7 {
                  n103 = Index Array(array=w770, index (row) #1=w771, index (col) #1=0, index (row) #2=w771, index (col) #2=1, index (row) #3=w771, index (col) #3=2) -> (element #1=w772:dbl, element #2=w774:dbl, element #3=w773:dbl)
                }
              }
            }
            frame "West" {
              w782 = 6
              n104 = case shown="2" w782 {
                tunnel: [w786 w792 w800 w808 w816 w825 w832 w841] -> w779
                tunnel: [w788 w794 w802 w809 w818 w827 w834 w843] -> w780
                tunnel: [w787 w793 w801 w810 w817 w826 w833 w842] -> w778
                tunnel: w782 -> [w790 w795 w803 w811 w819 w824 w835 w840]
                tunnel: w781 -> [w783 w791 w799 w807 w815 w823 w831 w839]
                frame 0, Default {
                  n105 = Index Array(array=w783, index (row) #1=w790, index (col) #1=0, index (row) #2=w790, index (col) #2=1, index (row) #3=w790, index (col) #3=2) -> (element #1=w788:dbl, element #2=w787:dbl, element #3=w786:dbl)
                }
                frame 1 {
                  n106 = Index Array(array=w791, index (row) #1=w795, index (col) #1=0, index (row) #2=w795, index (col) #2=1, index (row) #3=w795, index (col) #3=2) -> (element #1=w794:dbl, element #2=w793:dbl, element #3=w792:dbl)
                }
                frame 2 {
                  n107 = Index Array(array=w799, index (row) #1=w803, index (col) #1=0, index (row) #2=w803, index (col) #2=1, index (row) #3=w803, index (col) #3=2) -> (element #1=w802:dbl, element #2=w801:dbl, element #3=w800:dbl)
                }
                frame 3 {
                  n108 = Index Array(array=w807, index (row) #1=w811, index (col) #1=0, index (row) #2=w811, index (col) #2=1, index (row) #3=w811, index (col) #3=2) -> (element #1=w809:dbl, element #2=w810:dbl, element #3=w808:dbl)
                }
                frame 4 {
                  n109 = Index Array(array=w815, index (row) #1=w819, index (col) #1=0, index (row) #2=w819, index (col) #2=1, index (row) #3=w819, index (col) #3=2) -> (element #1=w816:dbl, element #2=w818:dbl, element #3=w817:dbl)
                }
                frame 5 {
                  n110 = Index Array(array=w823, index (row) #1=w824, index (col) #1=0, index (row) #2=w824, index (col) #2=1, index (row) #3=w824, index (col) #3=2) -> (element #1=w825:dbl, element #2=w826:dbl, element #3=w827:dbl)
                }
                frame 6 {
                  n111 = Index Array(array=w831, index (row) #1=w835, index (col) #1=0, index (row) #2=w835, index (col) #2=1, index (row) #3=w835, index (col) #3=2) -> (element #1=w832:dbl, element #2=w834:dbl, element #3=w833:dbl)
                }
                frame 7 {
                  n112 = Index Array(array=w839, index (row) #1=w840, index (col) #1=0, index (row) #2=w840, index (col) #2=1, index (row) #3=w840, index (col) #3=2) -> (element #1=w841:dbl, element #2=w843:dbl, element #3=w842:dbl)
                }
              }
            }
            frame "East" {
              w851 = 1
              n113 = case shown="2" w851 {
                tunnel: [w855 w861 w869 w877 w885 w894 w901 w910] -> w849
                tunnel: [w857 w863 w871 w878 w887 w896 w903 w912] -> w848
                tunnel: [w856 w862 w870 w879 w886 w895 w902 w911] -> w847
                tunnel: w851 -> [w859 w864 w872 w880 w888 w893 w904 w909]
                tunnel: w850 -> [w852 w860 w868 w876 w884 w892 w900 w908]
                frame 0, Default {
                  n114 = Index Array(array=w852, index (row) #1=w859, index (col) #1=0, index (row) #2=w859, index (col) #2=1, index (row) #3=w859, index (col) #3=2) -> (element #1=w857:dbl, element #2=w856:dbl, element #3=w855:dbl)
                }
                frame 1 {
                  n115 = Index Array(array=w860, index (row) #1=w864, index (col) #1=0, index (row) #2=w864, index (col) #2=1, index (row) #3=w864, index (col) #3=2) -> (element #1=w863:dbl, element #2=w862:dbl, element #3=w861:dbl)
                }
                frame 2 {
                  n116 = Index Array(array=w868, index (row) #1=w872, index (col) #1=0, index (row) #2=w872, index (col) #2=1, index (row) #3=w872, index (col) #3=2) -> (element #1=w871:dbl, element #2=w870:dbl, element #3=w869:dbl)
                }
                frame 3 {
                  n117 = Index Array(array=w876, index (row) #1=w880, index (col) #1=0, index (row) #2=w880, index (col) #2=1, index (row) #3=w880, index (col) #3=2) -> (element #1=w878:dbl, element #2=w879:dbl, element #3=w877:dbl)
                }
                frame 4 {
                  n118 = Index Array(array=w884, index (row) #1=w888, index (col) #1=0, index (row) #2=w888, index (col) #2=1, index (row) #3=w888, index (col) #3=2) -> (element #1=w885:dbl, element #2=w887:dbl, element #3=w886:dbl)
                }
                frame 5 {
                  n119 = Index Array(array=w892, index (row) #1=w893, index (col) #1=0, index (row) #2=w893, index (col) #2=1, index (row) #3=w893, index (col) #3=2) -> (element #1=w894:dbl, element #2=w895:dbl, element #3=w896:dbl)
                }
                frame 6 {
                  n120 = Index Array(array=w900, index (row) #1=w904, index (col) #1=0, index (row) #2=w904, index (col) #2=1, index (row) #3=w904, index (col) #3=2) -> (element #1=w901:dbl, element #2=w903:dbl, element #3=w902:dbl)
                }
                frame 7 {
                  n121 = Index Array(array=w908, index (row) #1=w909, index (col) #1=0, index (row) #2=w909, index (col) #2=1, index (row) #3=w909, index (col) #3=2) -> (element #1=w910:dbl, element #2=w912:dbl, element #3=w911:dbl)
                }
              }
            }
            frame "South" {
              w920 = 5
              n122 = case shown="2" w920 {
                tunnel: [w924 w930 w938 w946 w954 w963 w970 w979] -> w919
                tunnel: [w926 w932 w940 w947 w956 w965 w972 w981] -> w917
                tunnel: [w925 w931 w939 w948 w955 w964 w971 w980] -> w916
                tunnel: w920 -> [w928 w933 w941 w949 w957 w962 w973 w978]
                tunnel: w918 -> [w921 w929 w937 w945 w953 w961 w969 w977]
                frame 0, Default {
                  n123 = Index Array(array=w921, index (row) #1=w928, index (col) #1=0, index (row) #2=w928, index (col) #2=1, index (row) #3=w928, index (col) #3=2) -> (element #1=w926:dbl, element #2=w925:dbl, element #3=w924:dbl)
                }
                frame 1 {
                  n124 = Index Array(array=w929, index (row) #1=w933, index (col) #1=0, index (row) #2=w933, index (col) #2=1, index (row) #3=w933, index (col) #3=2) -> (element #1=w932:dbl, element #2=w931:dbl, element #3=w930:dbl)
                }
                frame 2 {
                  n125 = Index Array(array=w937, index (row) #1=w941, index (col) #1=0, index (row) #2=w941, index (col) #2=1, index (row) #3=w941, index (col) #3=2) -> (element #1=w940:dbl, element #2=w939:dbl, element #3=w938:dbl)
                }
                frame 3 {
                  n126 = Index Array(array=w945, index (row) #1=w949, index (col) #1=0, index (row) #2=w949, index (col) #2=1, index (row) #3=w949, index (col) #3=2) -> (element #1=w947:dbl, element #2=w948:dbl, element #3=w946:dbl)
                }
                frame 4 {
                  n127 = Index Array(array=w953, index (row) #1=w957, index (col) #1=0, index (row) #2=w957, index (col) #2=1, index (row) #3=w957, index (col) #3=2) -> (element #1=w954:dbl, element #2=w956:dbl, element #3=w955:dbl)
                }
                frame 5 {
                  n128 = Index Array(array=w961, index (row) #1=w962, index (col) #1=0, index (row) #2=w962, index (col) #2=1, index (row) #3=w962, index (col) #3=2) -> (element #1=w963:dbl, element #2=w964:dbl, element #3=w965:dbl)
                }
                frame 6 {
                  n129 = Index Array(array=w969, index (row) #1=w973, index (col) #1=0, index (row) #2=w973, index (col) #2=1, index (row) #3=w973, index (col) #3=2) -> (element #1=w970:dbl, element #2=w972:dbl, element #3=w971:dbl)
                }
                frame 7 {
                  n130 = Index Array(array=w977, index (row) #1=w978, index (col) #1=0, index (row) #2=w978, index (col) #2=1, index (row) #3=w978, index (col) #3=2) -> (element #1=w979:dbl, element #2=w981:dbl, element #3=w980:dbl)
                }
              }
            }
            frame "South west" {
              w989 = 7
              n131 = case shown="2" w989 {
                tunnel: [w993 w999 w1007 w1015 w1023 w1032 w1039 w1048] -> w987
                tunnel: [w995 w1001 w1009 w1016 w1025 w1034 w1041 w1050] -> w986
                tunnel: [w994 w1000 w1008 w1017 w1024 w1033 w1040 w1049] -> w985
                tunnel: w989 -> [w997 w1002 w1010 w1018 w1026 w1031 w1042 w1047]
                tunnel: w988 -> [w990 w998 w1006 w1014 w1022 w1030 w1038 w1046]
                frame 0, Default {
                  n132 = Index Array(array=w990, index (row) #1=w997, index (col) #1=0, index (row) #2=w997, index (col) #2=1, index (row) #3=w997, index (col) #3=2) -> (element #1=w995:dbl, element #2=w994:dbl, element #3=w993:dbl)
                }
                frame 1 {
                  n133 = Index Array(array=w998, index (row) #1=w1002, index (col) #1=0, index (row) #2=w1002, index (col) #2=1, index (row) #3=w1002, index (col) #3=2) -> (element #1=w1001:dbl, element #2=w1000:dbl, element #3=w999:dbl)
                }
                frame 2 {
                  n134 = Index Array(array=w1006, index (row) #1=w1010, index (col) #1=0, index (row) #2=w1010, index (col) #2=1, index (row) #3=w1010, index (col) #3=2) -> (element #1=w1009:dbl, element #2=w1008:dbl, element #3=w1007:dbl)
                }
                frame 3 {
                  n135 = Index Array(array=w1014, index (row) #1=w1018, index (col) #1=0, index (row) #2=w1018, index (col) #2=1, index (row) #3=w1018, index (col) #3=2) -> (element #1=w1016:dbl, element #2=w1017:dbl, element #3=w1015:dbl)
                }
                frame 4 {
                  n136 = Index Array(array=w1022, index (row) #1=w1026, index (col) #1=0, index (row) #2=w1026, index (col) #2=1, index (row) #3=w1026, index (col) #3=2) -> (element #1=w1023:dbl, element #2=w1025:dbl, element #3=w1024:dbl)
                }
                frame 5 {
                  n137 = Index Array(array=w1030, index (row) #1=w1031, index (col) #1=0, index (row) #2=w1031, index (col) #2=1, index (row) #3=w1031, index (col) #3=2) -> (element #1=w1032:dbl, element #2=w1033:dbl, element #3=w1034:dbl)
                }
                frame 6 {
                  n138 = Index Array(array=w1038, index (row) #1=w1042, index (col) #1=0, index (row) #2=w1042, index (col) #2=1, index (row) #3=w1042, index (col) #3=2) -> (element #1=w1039:dbl, element #2=w1041:dbl, element #3=w1040:dbl)
                }
                frame 7 {
                  n139 = Index Array(array=w1046, index (row) #1=w1047, index (col) #1=0, index (row) #2=w1047, index (col) #2=1, index (row) #3=w1047, index (col) #3=2) -> (element #1=w1048:dbl, element #2=w1050:dbl, element #3=w1049:dbl)
                }
              }
            }
            frame "South east" {
              w1058 = 3
              n140 = case shown="2" w1058 {
                tunnel: [w1062 w1068 w1076 w1084 w1092 w1101 w1108 w1117] -> w1057
                tunnel: [w1064 w1070 w1078 w1085 w1094 w1103 w1110 w1119] -> w1056
                tunnel: [w1063 w1069 w1077 w1086 w1093 w1102 w1109 w1118] -> w1055
                tunnel: w1058 -> [w1066 w1071 w1079 w1087 w1095 w1100 w1111 w1116]
                tunnel: w1054 -> [w1059 w1067 w1075 w1083 w1091 w1099 w1107 w1115]
                frame 0, Default {
                  n141 = Index Array(array=w1059, index (row) #1=w1066, index (col) #1=0, index (row) #2=w1066, index (col) #2=1, index (row) #3=w1066, index (col) #3=2) -> (element #1=w1064:dbl, element #2=w1063:dbl, element #3=w1062:dbl)
                }
                frame 1 {
                  n142 = Index Array(array=w1067, index (row) #1=w1071, index (col) #1=0, index (row) #2=w1071, index (col) #2=1, index (row) #3=w1071, index (col) #3=2) -> (element #1=w1070:dbl, element #2=w1069:dbl, element #3=w1068:dbl)
                }
                frame 2 {
                  n143 = Index Array(array=w1075, index (row) #1=w1079, index (col) #1=0, index (row) #2=w1079, index (col) #2=1, index (row) #3=w1079, index (col) #3=2) -> (element #1=w1078:dbl, element #2=w1077:dbl, element #3=w1076:dbl)
                }
                frame 3 {
                  n144 = Index Array(array=w1083, index (row) #1=w1087, index (col) #1=0, index (row) #2=w1087, index (col) #2=1, index (row) #3=w1087, index (col) #3=2) -> (element #1=w1085:dbl, element #2=w1086:dbl, element #3=w1084:dbl)
                }
                frame 4 {
                  n145 = Index Array(array=w1091, index (row) #1=w1095, index (col) #1=0, index (row) #2=w1095, index (col) #2=1, index (row) #3=w1095, index (col) #3=2) -> (element #1=w1092:dbl, element #2=w1094:dbl, element #3=w1093:dbl)
                }
                frame 5 {
                  n146 = Index Array(array=w1099, index (row) #1=w1100, index (col) #1=0, index (row) #2=w1100, index (col) #2=1, index (row) #3=w1100, index (col) #3=2) -> (element #1=w1101:dbl, element #2=w1102:dbl, element #3=w1103:dbl)
                }
                frame 6 {
                  n147 = Index Array(array=w1107, index (row) #1=w1111, index (col) #1=0, index (row) #2=w1111, index (col) #2=1, index (row) #3=w1111, index (col) #3=2) -> (element #1=w1108:dbl, element #2=w1110:dbl, element #3=w1109:dbl)
                }
                frame 7 {
                  n148 = Index Array(array=w1115, index (row) #1=w1116, index (col) #1=0, index (row) #2=w1116, index (col) #2=1, index (row) #3=w1116, index (col) #3=2) -> (element #1=w1117:dbl, element #2=w1119:dbl, element #3=w1118:dbl)
                }
              }
            }
          }
        }
        frame "North west" {
          n149 = case shown="\"South east\"" w1127 {
            tunnel: [w1131 w1201 w1269 w1336 w1406 w1476 w1544 w1614] -> w1125
            tunnel: [w1130 w1200 w1268 w1337 w1405 w1474 w1543 w1613] -> w1124
            tunnel: [w1129 w1199 w1267 w1335 w1404 w1473 w1542 w1612] -> w1123
            tunnel: w1126 -> [w1128 w1197 w1266 w1338 w1407 w1475 w1545 w1611]
            frame "North", Default {
              w1132 = 1
              n150 = case shown="2" w1132 {
                tunnel: [w1136 w1142 w1150 w1158 w1166 w1175 w1182 w1191] -> w1131
                tunnel: [w1138 w1144 w1152 w1159 w1168 w1177 w1184 w1193] -> w1130
                tunnel: [w1137 w1143 w1151 w1160 w1167 w1176 w1183 w1192] -> w1129
                tunnel: w1132 -> [w1140 w1145 w1153 w1161 w1169 w1174 w1185 w1190]
                tunnel: w1128 -> [w1133 w1141 w1149 w1157 w1165 w1173 w1181 w1189]
                frame 0, Default {
                  n151 = Index Array(array=w1133, index (row) #1=w1140, index (col) #1=0, index (row) #2=w1140, index (col) #2=1, index (row) #3=w1140, index (col) #3=2) -> (element #1=w1138:dbl, element #2=w1137:dbl, element #3=w1136:dbl)
                }
                frame 1 {
                  n152 = Index Array(array=w1141, index (row) #1=w1145, index (col) #1=0, index (row) #2=w1145, index (col) #2=1, index (row) #3=w1145, index (col) #3=2) -> (element #1=w1144:dbl, element #2=w1143:dbl, element #3=w1142:dbl)
                }
                frame 2 {
                  n153 = Index Array(array=w1149, index (row) #1=w1153, index (col) #1=0, index (row) #2=w1153, index (col) #2=1, index (row) #3=w1153, index (col) #3=2) -> (element #1=w1152:dbl, element #2=w1151:dbl, element #3=w1150:dbl)
                }
                frame 3 {
                  n154 = Index Array(array=w1157, index (row) #1=w1161, index (col) #1=0, index (row) #2=w1161, index (col) #2=1, index (row) #3=w1161, index (col) #3=2) -> (element #1=w1159:dbl, element #2=w1160:dbl, element #3=w1158:dbl)
                }
                frame 4 {
                  n155 = Index Array(array=w1165, index (row) #1=w1169, index (col) #1=0, index (row) #2=w1169, index (col) #2=1, index (row) #3=w1169, index (col) #3=2) -> (element #1=w1166:dbl, element #2=w1168:dbl, element #3=w1167:dbl)
                }
                frame 5 {
                  n156 = Index Array(array=w1173, index (row) #1=w1174, index (col) #1=0, index (row) #2=w1174, index (col) #2=1, index (row) #3=w1174, index (col) #3=2) -> (element #1=w1175:dbl, element #2=w1176:dbl, element #3=w1177:dbl)
                }
                frame 6 {
                  n157 = Index Array(array=w1181, index (row) #1=w1185, index (col) #1=0, index (row) #2=w1185, index (col) #2=1, index (row) #3=w1185, index (col) #3=2) -> (element #1=w1182:dbl, element #2=w1184:dbl, element #3=w1183:dbl)
                }
                frame 7 {
                  n158 = Index Array(array=w1189, index (row) #1=w1190, index (col) #1=0, index (row) #2=w1190, index (col) #2=1, index (row) #3=w1190, index (col) #3=2) -> (element #1=w1191:dbl, element #2=w1193:dbl, element #3=w1192:dbl)
                }
              }
            }
            frame "North east" {
              w1198 = 3
              n159 = case shown="2" w1198 {
                tunnel: [w1205 w1211 w1219 w1227 w1235 w1244 w1251 w1260] -> w1201
                tunnel: [w1207 w1213 w1221 w1228 w1237 w1246 w1253 w1262] -> w1200
                tunnel: [w1206 w1212 w1220 w1229 w1236 w1245 w1252 w1261] -> w1199
                tunnel: w1198 -> [w1209 w1214 w1222 w1230 w1238 w1243 w1254 w1259]
                tunnel: w1197 -> [w1202 w1210 w1218 w1226 w1234 w1242 w1250 w1258]
                frame 0, Default {
                  n160 = Index Array(array=w1202, index (row) #1=w1209, index (col) #1=0, index (row) #2=w1209, index (col) #2=1, index (row) #3=w1209, index (col) #3=2) -> (element #1=w1207:dbl, element #2=w1206:dbl, element #3=w1205:dbl)
                }
                frame 1 {
                  n161 = Index Array(array=w1210, index (row) #1=w1214, index (col) #1=0, index (row) #2=w1214, index (col) #2=1, index (row) #3=w1214, index (col) #3=2) -> (element #1=w1213:dbl, element #2=w1212:dbl, element #3=w1211:dbl)
                }
                frame 2 {
                  n162 = Index Array(array=w1218, index (row) #1=w1222, index (col) #1=0, index (row) #2=w1222, index (col) #2=1, index (row) #3=w1222, index (col) #3=2) -> (element #1=w1221:dbl, element #2=w1220:dbl, element #3=w1219:dbl)
                }
                frame 3 {
                  n163 = Index Array(array=w1226, index (row) #1=w1230, index (col) #1=0, index (row) #2=w1230, index (col) #2=1, index (row) #3=w1230, index (col) #3=2) -> (element #1=w1228:dbl, element #2=w1229:dbl, element #3=w1227:dbl)
                }
                frame 4 {
                  n164 = Index Array(array=w1234, index (row) #1=w1238, index (col) #1=0, index (row) #2=w1238, index (col) #2=1, index (row) #3=w1238, index (col) #3=2) -> (element #1=w1235:dbl, element #2=w1237:dbl, element #3=w1236:dbl)
                }
                frame 5 {
                  n165 = Index Array(array=w1242, index (row) #1=w1243, index (col) #1=0, index (row) #2=w1243, index (col) #2=1, index (row) #3=w1243, index (col) #3=2) -> (element #1=w1244:dbl, element #2=w1245:dbl, element #3=w1246:dbl)
                }
                frame 6 {
                  n166 = Index Array(array=w1250, index (row) #1=w1254, index (col) #1=0, index (row) #2=w1254, index (col) #2=1, index (row) #3=w1254, index (col) #3=2) -> (element #1=w1251:dbl, element #2=w1253:dbl, element #3=w1252:dbl)
                }
                frame 7 {
                  n167 = Index Array(array=w1258, index (row) #1=w1259, index (col) #1=0, index (row) #2=w1259, index (col) #2=1, index (row) #3=w1259, index (col) #3=2) -> (element #1=w1260:dbl, element #2=w1262:dbl, element #3=w1261:dbl)
                }
              }
            }
            frame "North west" {
              w1270 = 0
              n168 = case shown="2" w1270 {
                tunnel: [w1274 w1280 w1288 w1296 w1304 w1313 w1320 w1329] -> w1269
                tunnel: [w1276 w1282 w1290 w1297 w1306 w1315 w1322 w1331] -> w1268
                tunnel: [w1275 w1281 w1289 w1298 w1305 w1314 w1321 w1330] -> w1267
                tunnel: w1270 -> [w1278 w1283 w1291 w1299 w1307 w1312 w1323 w1328]
                tunnel: w1266 -> [w1271 w1279 w1287 w1295 w1303 w1311 w1319 w1327]
                frame 0, Default {
                  n169 = Index Array(array=w1271, index (row) #1=w1278, index (col) #1=0, index (row) #2=w1278, index (col) #2=1, index (row) #3=w1278, index (col) #3=2) -> (element #1=w1276:dbl, element #2=w1275:dbl, element #3=w1274:dbl)
                }
                frame 1 {
                  n170 = Index Array(array=w1279, index (row) #1=w1283, index (col) #1=0, index (row) #2=w1283, index (col) #2=1, index (row) #3=w1283, index (col) #3=2) -> (element #1=w1282:dbl, element #2=w1281:dbl, element #3=w1280:dbl)
                }
                frame 2 {
                  n171 = Index Array(array=w1287, index (row) #1=w1291, index (col) #1=0, index (row) #2=w1291, index (col) #2=1, index (row) #3=w1291, index (col) #3=2) -> (element #1=w1290:dbl, element #2=w1289:dbl, element #3=w1288:dbl)
                }
                frame 3 {
                  n172 = Index Array(array=w1295, index (row) #1=w1299, index (col) #1=0, index (row) #2=w1299, index (col) #2=1, index (row) #3=w1299, index (col) #3=2) -> (element #1=w1297:dbl, element #2=w1298:dbl, element #3=w1296:dbl)
                }
                frame 4 {
                  n173 = Index Array(array=w1303, index (row) #1=w1307, index (col) #1=0, index (row) #2=w1307, index (col) #2=1, index (row) #3=w1307, index (col) #3=2) -> (element #1=w1304:dbl, element #2=w1306:dbl, element #3=w1305:dbl)
                }
                frame 5 {
                  n174 = Index Array(array=w1311, index (row) #1=w1312, index (col) #1=0, index (row) #2=w1312, index (col) #2=1, index (row) #3=w1312, index (col) #3=2) -> (element #1=w1313:dbl, element #2=w1314:dbl, element #3=w1315:dbl)
                }
                frame 6 {
                  n175 = Index Array(array=w1319, index (row) #1=w1323, index (col) #1=0, index (row) #2=w1323, index (col) #2=1, index (row) #3=w1323, index (col) #3=2) -> (element #1=w1320:dbl, element #2=w1322:dbl, element #3=w1321:dbl)
                }
                frame 7 {
                  n176 = Index Array(array=w1327, index (row) #1=w1328, index (col) #1=0, index (row) #2=w1328, index (col) #2=1, index (row) #3=w1328, index (col) #3=2) -> (element #1=w1329:dbl, element #2=w1331:dbl, element #3=w1330:dbl)
                }
              }
            }
            frame "West" {
              w1339 = 2
              n177 = case shown="2" w1339 {
                tunnel: [w1343 w1349 w1357 w1365 w1373 w1382 w1389 w1398] -> w1336
                tunnel: [w1345 w1351 w1359 w1366 w1375 w1384 w1391 w1400] -> w1337
                tunnel: [w1344 w1350 w1358 w1367 w1374 w1383 w1390 w1399] -> w1335
                tunnel: w1339 -> [w1347 w1352 w1360 w1368 w1376 w1381 w1392 w1397]
                tunnel: w1338 -> [w1340 w1348 w1356 w1364 w1372 w1380 w1388 w1396]
                frame 0, Default {
                  n178 = Index Array(array=w1340, index (row) #1=w1347, index (col) #1=0, index (row) #2=w1347, index (col) #2=1, index (row) #3=w1347, index (col) #3=2) -> (element #1=w1345:dbl, element #2=w1344:dbl, element #3=w1343:dbl)
                }
                frame 1 {
                  n179 = Index Array(array=w1348, index (row) #1=w1352, index (col) #1=0, index (row) #2=w1352, index (col) #2=1, index (row) #3=w1352, index (col) #3=2) -> (element #1=w1351:dbl, element #2=w1350:dbl, element #3=w1349:dbl)
                }
                frame 2 {
                  n180 = Index Array(array=w1356, index (row) #1=w1360, index (col) #1=0, index (row) #2=w1360, index (col) #2=1, index (row) #3=w1360, index (col) #3=2) -> (element #1=w1359:dbl, element #2=w1358:dbl, element #3=w1357:dbl)
                }
                frame 3 {
                  n181 = Index Array(array=w1364, index (row) #1=w1368, index (col) #1=0, index (row) #2=w1368, index (col) #2=1, index (row) #3=w1368, index (col) #3=2) -> (element #1=w1366:dbl, element #2=w1367:dbl, element #3=w1365:dbl)
                }
                frame 4 {
                  n182 = Index Array(array=w1372, index (row) #1=w1376, index (col) #1=0, index (row) #2=w1376, index (col) #2=1, index (row) #3=w1376, index (col) #3=2) -> (element #1=w1373:dbl, element #2=w1375:dbl, element #3=w1374:dbl)
                }
                frame 5 {
                  n183 = Index Array(array=w1380, index (row) #1=w1381, index (col) #1=0, index (row) #2=w1381, index (col) #2=1, index (row) #3=w1381, index (col) #3=2) -> (element #1=w1382:dbl, element #2=w1383:dbl, element #3=w1384:dbl)
                }
                frame 6 {
                  n184 = Index Array(array=w1388, index (row) #1=w1392, index (col) #1=0, index (row) #2=w1392, index (col) #2=1, index (row) #3=w1392, index (col) #3=2) -> (element #1=w1389:dbl, element #2=w1391:dbl, element #3=w1390:dbl)
                }
                frame 7 {
                  n185 = Index Array(array=w1396, index (row) #1=w1397, index (col) #1=0, index (row) #2=w1397, index (col) #2=1, index (row) #3=w1397, index (col) #3=2) -> (element #1=w1398:dbl, element #2=w1400:dbl, element #3=w1399:dbl)
                }
              }
            }
            frame "East" {
              w1408 = 5
              n186 = case shown="2" w1408 {
                tunnel: [w1412 w1418 w1426 w1434 w1442 w1451 w1458 w1467] -> w1406
                tunnel: [w1414 w1420 w1428 w1435 w1444 w1453 w1460 w1469] -> w1405
                tunnel: [w1413 w1419 w1427 w1436 w1443 w1452 w1459 w1468] -> w1404
                tunnel: w1408 -> [w1416 w1421 w1429 w1437 w1445 w1450 w1461 w1466]
                tunnel: w1407 -> [w1409 w1417 w1425 w1433 w1441 w1449 w1457 w1465]
                frame 0, Default {
                  n187 = Index Array(array=w1409, index (row) #1=w1416, index (col) #1=0, index (row) #2=w1416, index (col) #2=1, index (row) #3=w1416, index (col) #3=2) -> (element #1=w1414:dbl, element #2=w1413:dbl, element #3=w1412:dbl)
                }
                frame 1 {
                  n188 = Index Array(array=w1417, index (row) #1=w1421, index (col) #1=0, index (row) #2=w1421, index (col) #2=1, index (row) #3=w1421, index (col) #3=2) -> (element #1=w1420:dbl, element #2=w1419:dbl, element #3=w1418:dbl)
                }
                frame 2 {
                  n189 = Index Array(array=w1425, index (row) #1=w1429, index (col) #1=0, index (row) #2=w1429, index (col) #2=1, index (row) #3=w1429, index (col) #3=2) -> (element #1=w1428:dbl, element #2=w1427:dbl, element #3=w1426:dbl)
                }
                frame 3 {
                  n190 = Index Array(array=w1433, index (row) #1=w1437, index (col) #1=0, index (row) #2=w1437, index (col) #2=1, index (row) #3=w1437, index (col) #3=2) -> (element #1=w1435:dbl, element #2=w1436:dbl, element #3=w1434:dbl)
                }
                frame 4 {
                  n191 = Index Array(array=w1441, index (row) #1=w1445, index (col) #1=0, index (row) #2=w1445, index (col) #2=1, index (row) #3=w1445, index (col) #3=2) -> (element #1=w1442:dbl, element #2=w1444:dbl, element #3=w1443:dbl)
                }
                frame 5 {
                  n192 = Index Array(array=w1449, index (row) #1=w1450, index (col) #1=0, index (row) #2=w1450, index (col) #2=1, index (row) #3=w1450, index (col) #3=2) -> (element #1=w1451:dbl, element #2=w1452:dbl, element #3=w1453:dbl)
                }
                frame 6 {
                  n193 = Index Array(array=w1457, index (row) #1=w1461, index (col) #1=0, index (row) #2=w1461, index (col) #2=1, index (row) #3=w1461, index (col) #3=2) -> (element #1=w1458:dbl, element #2=w1460:dbl, element #3=w1459:dbl)
                }
                frame 7 {
                  n194 = Index Array(array=w1465, index (row) #1=w1466, index (col) #1=0, index (row) #2=w1466, index (col) #2=1, index (row) #3=w1466, index (col) #3=2) -> (element #1=w1467:dbl, element #2=w1469:dbl, element #3=w1468:dbl)
                }
              }
            }
            frame "South" {
              w1477 = 6
              n195 = case shown="2" w1477 {
                tunnel: [w1481 w1487 w1495 w1503 w1511 w1520 w1527 w1536] -> w1476
                tunnel: [w1483 w1489 w1497 w1504 w1513 w1522 w1529 w1538] -> w1474
                tunnel: [w1482 w1488 w1496 w1505 w1512 w1521 w1528 w1537] -> w1473
                tunnel: w1477 -> [w1485 w1490 w1498 w1506 w1514 w1519 w1530 w1535]
                tunnel: w1475 -> [w1478 w1486 w1494 w1502 w1510 w1518 w1526 w1534]
                frame 0, Default {
                  n196 = Index Array(array=w1478, index (row) #1=w1485, index (col) #1=0, index (row) #2=w1485, index (col) #2=1, index (row) #3=w1485, index (col) #3=2) -> (element #1=w1483:dbl, element #2=w1482:dbl, element #3=w1481:dbl)
                }
                frame 1 {
                  n197 = Index Array(array=w1486, index (row) #1=w1490, index (col) #1=0, index (row) #2=w1490, index (col) #2=1, index (row) #3=w1490, index (col) #3=2) -> (element #1=w1489:dbl, element #2=w1488:dbl, element #3=w1487:dbl)
                }
                frame 2 {
                  n198 = Index Array(array=w1494, index (row) #1=w1498, index (col) #1=0, index (row) #2=w1498, index (col) #2=1, index (row) #3=w1498, index (col) #3=2) -> (element #1=w1497:dbl, element #2=w1496:dbl, element #3=w1495:dbl)
                }
                frame 3 {
                  n199 = Index Array(array=w1502, index (row) #1=w1506, index (col) #1=0, index (row) #2=w1506, index (col) #2=1, index (row) #3=w1506, index (col) #3=2) -> (element #1=w1504:dbl, element #2=w1505:dbl, element #3=w1503:dbl)
                }
                frame 4 {
                  n200 = Index Array(array=w1510, index (row) #1=w1514, index (col) #1=0, index (row) #2=w1514, index (col) #2=1, index (row) #3=w1514, index (col) #3=2) -> (element #1=w1511:dbl, element #2=w1513:dbl, element #3=w1512:dbl)
                }
                frame 5 {
                  n201 = Index Array(array=w1518, index (row) #1=w1519, index (col) #1=0, index (row) #2=w1519, index (col) #2=1, index (row) #3=w1519, index (col) #3=2) -> (element #1=w1520:dbl, element #2=w1521:dbl, element #3=w1522:dbl)
                }
                frame 6 {
                  n202 = Index Array(array=w1526, index (row) #1=w1530, index (col) #1=0, index (row) #2=w1530, index (col) #2=1, index (row) #3=w1530, index (col) #3=2) -> (element #1=w1527:dbl, element #2=w1529:dbl, element #3=w1528:dbl)
                }
                frame 7 {
                  n203 = Index Array(array=w1534, index (row) #1=w1535, index (col) #1=0, index (row) #2=w1535, index (col) #2=1, index (row) #3=w1535, index (col) #3=2) -> (element #1=w1536:dbl, element #2=w1538:dbl, element #3=w1537:dbl)
                }
              }
            }
            frame "South west" {
              w1546 = 4
              n204 = case shown="2" w1546 {
                tunnel: [w1550 w1556 w1564 w1572 w1580 w1589 w1596 w1605] -> w1544
                tunnel: [w1552 w1558 w1566 w1573 w1582 w1591 w1598 w1607] -> w1543
                tunnel: [w1551 w1557 w1565 w1574 w1581 w1590 w1597 w1606] -> w1542
                tunnel: w1546 -> [w1554 w1559 w1567 w1575 w1583 w1588 w1599 w1604]
                tunnel: w1545 -> [w1547 w1555 w1563 w1571 w1579 w1587 w1595 w1603]
                frame 0, Default {
                  n205 = Index Array(array=w1547, index (row) #1=w1554, index (col) #1=0, index (row) #2=w1554, index (col) #2=1, index (row) #3=w1554, index (col) #3=2) -> (element #1=w1552:dbl, element #2=w1551:dbl, element #3=w1550:dbl)
                }
                frame 1 {
                  n206 = Index Array(array=w1555, index (row) #1=w1559, index (col) #1=0, index (row) #2=w1559, index (col) #2=1, index (row) #3=w1559, index (col) #3=2) -> (element #1=w1558:dbl, element #2=w1557:dbl, element #3=w1556:dbl)
                }
                frame 2 {
                  n207 = Index Array(array=w1563, index (row) #1=w1567, index (col) #1=0, index (row) #2=w1567, index (col) #2=1, index (row) #3=w1567, index (col) #3=2) -> (element #1=w1566:dbl, element #2=w1565:dbl, element #3=w1564:dbl)
                }
                frame 3 {
                  n208 = Index Array(array=w1571, index (row) #1=w1575, index (col) #1=0, index (row) #2=w1575, index (col) #2=1, index (row) #3=w1575, index (col) #3=2) -> (element #1=w1573:dbl, element #2=w1574:dbl, element #3=w1572:dbl)
                }
                frame 4 {
                  n209 = Index Array(array=w1579, index (row) #1=w1583, index (col) #1=0, index (row) #2=w1583, index (col) #2=1, index (row) #3=w1583, index (col) #3=2) -> (element #1=w1580:dbl, element #2=w1582:dbl, element #3=w1581:dbl)
                }
                frame 5 {
                  n210 = Index Array(array=w1587, index (row) #1=w1588, index (col) #1=0, index (row) #2=w1588, index (col) #2=1, index (row) #3=w1588, index (col) #3=2) -> (element #1=w1589:dbl, element #2=w1590:dbl, element #3=w1591:dbl)
                }
                frame 6 {
                  n211 = Index Array(array=w1595, index (row) #1=w1599, index (col) #1=0, index (row) #2=w1599, index (col) #2=1, index (row) #3=w1599, index (col) #3=2) -> (element #1=w1596:dbl, element #2=w1598:dbl, element #3=w1597:dbl)
                }
                frame 7 {
                  n212 = Index Array(array=w1603, index (row) #1=w1604, index (col) #1=0, index (row) #2=w1604, index (col) #2=1, index (row) #3=w1604, index (col) #3=2) -> (element #1=w1605:dbl, element #2=w1607:dbl, element #3=w1606:dbl)
                }
              }
            }
            frame "South east" {
              w1615 = 7
              n213 = case shown="2" w1615 {
                tunnel: [w1619 w1625 w1633 w1641 w1649 w1658 w1665 w1674] -> w1614
                tunnel: [w1621 w1627 w1635 w1642 w1651 w1660 w1667 w1676] -> w1613
                tunnel: [w1620 w1626 w1634 w1643 w1650 w1659 w1666 w1675] -> w1612
                tunnel: w1615 -> [w1623 w1628 w1636 w1644 w1652 w1657 w1668 w1673]
                tunnel: w1611 -> [w1616 w1624 w1632 w1640 w1648 w1656 w1664 w1672]
                frame 0, Default {
                  n214 = Index Array(array=w1616, index (row) #1=w1623, index (col) #1=0, index (row) #2=w1623, index (col) #2=1, index (row) #3=w1623, index (col) #3=2) -> (element #1=w1621:dbl, element #2=w1620:dbl, element #3=w1619:dbl)
                }
                frame 1 {
                  n215 = Index Array(array=w1624, index (row) #1=w1628, index (col) #1=0, index (row) #2=w1628, index (col) #2=1, index (row) #3=w1628, index (col) #3=2) -> (element #1=w1627:dbl, element #2=w1626:dbl, element #3=w1625:dbl)
                }
                frame 2 {
                  n216 = Index Array(array=w1632, index (row) #1=w1636, index (col) #1=0, index (row) #2=w1636, index (col) #2=1, index (row) #3=w1636, index (col) #3=2) -> (element #1=w1635:dbl, element #2=w1634:dbl, element #3=w1633:dbl)
                }
                frame 3 {
                  n217 = Index Array(array=w1640, index (row) #1=w1644, index (col) #1=0, index (row) #2=w1644, index (col) #2=1, index (row) #3=w1644, index (col) #3=2) -> (element #1=w1642:dbl, element #2=w1643:dbl, element #3=w1641:dbl)
                }
                frame 4 {
                  n218 = Index Array(array=w1648, index (row) #1=w1652, index (col) #1=0, index (row) #2=w1652, index (col) #2=1, index (row) #3=w1652, index (col) #3=2) -> (element #1=w1649:dbl, element #2=w1651:dbl, element #3=w1650:dbl)
                }
                frame 5 {
                  n219 = Index Array(array=w1656, index (row) #1=w1657, index (col) #1=0, index (row) #2=w1657, index (col) #2=1, index (row) #3=w1657, index (col) #3=2) -> (element #1=w1658:dbl, element #2=w1659:dbl, element #3=w1660:dbl)
                }
                frame 6 {
                  n220 = Index Array(array=w1664, index (row) #1=w1668, index (col) #1=0, index (row) #2=w1668, index (col) #2=1, index (row) #3=w1668, index (col) #3=2) -> (element #1=w1665:dbl, element #2=w1667:dbl, element #3=w1666:dbl)
                }
                frame 7 {
                  n221 = Index Array(array=w1672, index (row) #1=w1673, index (col) #1=0, index (row) #2=w1673, index (col) #2=1, index (row) #3=w1673, index (col) #3=2) -> (element #1=w1674:dbl, element #2=w1676:dbl, element #3=w1675:dbl)
                }
              }
            }
          }
        }
        frame "West" {
          n222 = case shown="\"North\", Default" w1684 {
            tunnel: [w1688 w1758 w1826 w1893 w1963 w2033 w2101 w2171] -> w1682
            tunnel: [w1687 w1757 w1825 w1894 w1962 w2031 w2100 w2170] -> w1681
            tunnel: [w1686 w1756 w1824 w1892 w1961 w2030 w2099 w2169] -> w1680
            tunnel: w1683 -> [w1685 w1754 w1823 w1895 w1964 w2032 w2102 w2168]
            frame "North", Default {
              w1689 = 3
              n223 = case shown="2" w1689 {
                tunnel: [w1693 w1699 w1707 w1715 w1723 w1732 w1739 w1748] -> w1688
                tunnel: [w1695 w1701 w1709 w1716 w1725 w1734 w1741 w1750] -> w1687
                tunnel: [w1694 w1700 w1708 w1717 w1724 w1733 w1740 w1749] -> w1686
                tunnel: w1689 -> [w1697 w1702 w1710 w1718 w1726 w1731 w1742 w1747]
                tunnel: w1685 -> [w1690 w1698 w1706 w1714 w1722 w1730 w1738 w1746]
                frame 0, Default {
                  n224 = Index Array(array=w1690, index (row) #1=w1697, index (col) #1=0, index (row) #2=w1697, index (col) #2=1, index (row) #3=w1697, index (col) #3=2) -> (element #1=w1695:dbl, element #2=w1694:dbl, element #3=w1693:dbl)
                }
                frame 1 {
                  n225 = Index Array(array=w1698, index (row) #1=w1702, index (col) #1=0, index (row) #2=w1702, index (col) #2=1, index (row) #3=w1702, index (col) #3=2) -> (element #1=w1701:dbl, element #2=w1700:dbl, element #3=w1699:dbl)
                }
                frame 2 {
                  n226 = Index Array(array=w1706, index (row) #1=w1710, index (col) #1=0, index (row) #2=w1710, index (col) #2=1, index (row) #3=w1710, index (col) #3=2) -> (element #1=w1709:dbl, element #2=w1708:dbl, element #3=w1707:dbl)
                }
                frame 3 {
                  n227 = Index Array(array=w1714, index (row) #1=w1718, index (col) #1=0, index (row) #2=w1718, index (col) #2=1, index (row) #3=w1718, index (col) #3=2) -> (element #1=w1716:dbl, element #2=w1717:dbl, element #3=w1715:dbl)
                }
                frame 4 {
                  n228 = Index Array(array=w1722, index (row) #1=w1726, index (col) #1=0, index (row) #2=w1726, index (col) #2=1, index (row) #3=w1726, index (col) #3=2) -> (element #1=w1723:dbl, element #2=w1725:dbl, element #3=w1724:dbl)
                }
                frame 5 {
                  n229 = Index Array(array=w1730, index (row) #1=w1731, index (col) #1=0, index (row) #2=w1731, index (col) #2=1, index (row) #3=w1731, index (col) #3=2) -> (element #1=w1732:dbl, element #2=w1733:dbl, element #3=w1734:dbl)
                }
                frame 6 {
                  n230 = Index Array(array=w1738, index (row) #1=w1742, index (col) #1=0, index (row) #2=w1742, index (col) #2=1, index (row) #3=w1742, index (col) #3=2) -> (element #1=w1739:dbl, element #2=w1741:dbl, element #3=w1740:dbl)
                }
                frame 7 {
                  n231 = Index Array(array=w1746, index (row) #1=w1747, index (col) #1=0, index (row) #2=w1747, index (col) #2=1, index (row) #3=w1747, index (col) #3=2) -> (element #1=w1748:dbl, element #2=w1750:dbl, element #3=w1749:dbl)
                }
              }
            }
            frame "North east" {
              w1755 = 5
              n232 = case shown="2" w1755 {
                tunnel: [w1762 w1768 w1776 w1784 w1792 w1801 w1808 w1817] -> w1758
                tunnel: [w1764 w1770 w1778 w1785 w1794 w1803 w1810 w1819] -> w1757
                tunnel: [w1763 w1769 w1777 w1786 w1793 w1802 w1809 w1818] -> w1756
                tunnel: w1755 -> [w1766 w1771 w1779 w1787 w1795 w1800 w1811 w1816]
                tunnel: w1754 -> [w1759 w1767 w1775 w1783 w1791 w1799 w1807 w1815]
                frame 0, Default {
                  n233 = Index Array(array=w1759, index (row) #1=w1766, index (col) #1=0, index (row) #2=w1766, index (col) #2=1, index (row) #3=w1766, index (col) #3=2) -> (element #1=w1764:dbl, element #2=w1763:dbl, element #3=w1762:dbl)
                }
                frame 1 {
                  n234 = Index Array(array=w1767, index (row) #1=w1771, index (col) #1=0, index (row) #2=w1771, index (col) #2=1, index (row) #3=w1771, index (col) #3=2) -> (element #1=w1770:dbl, element #2=w1769:dbl, element #3=w1768:dbl)
                }
                frame 2 {
                  n235 = Index Array(array=w1775, index (row) #1=w1779, index (col) #1=0, index (row) #2=w1779, index (col) #2=1, index (row) #3=w1779, index (col) #3=2) -> (element #1=w1778:dbl, element #2=w1777:dbl, element #3=w1776:dbl)
                }
                frame 3 {
                  n236 = Index Array(array=w1783, index (row) #1=w1787, index (col) #1=0, index (row) #2=w1787, index (col) #2=1, index (row) #3=w1787, index (col) #3=2) -> (element #1=w1785:dbl, element #2=w1786:dbl, element #3=w1784:dbl)
                }
                frame 4 {
                  n237 = Index Array(array=w1791, index (row) #1=w1795, index (col) #1=0, index (row) #2=w1795, index (col) #2=1, index (row) #3=w1795, index (col) #3=2) -> (element #1=w1792:dbl, element #2=w1794:dbl, element #3=w1793:dbl)
                }
                frame 5 {
                  n238 = Index Array(array=w1799, index (row) #1=w1800, index (col) #1=0, index (row) #2=w1800, index (col) #2=1, index (row) #3=w1800, index (col) #3=2) -> (element #1=w1801:dbl, element #2=w1802:dbl, element #3=w1803:dbl)
                }
                frame 6 {
                  n239 = Index Array(array=w1807, index (row) #1=w1811, index (col) #1=0, index (row) #2=w1811, index (col) #2=1, index (row) #3=w1811, index (col) #3=2) -> (element #1=w1808:dbl, element #2=w1810:dbl, element #3=w1809:dbl)
                }
                frame 7 {
                  n240 = Index Array(array=w1815, index (row) #1=w1816, index (col) #1=0, index (row) #2=w1816, index (col) #2=1, index (row) #3=w1816, index (col) #3=2) -> (element #1=w1817:dbl, element #2=w1819:dbl, element #3=w1818:dbl)
                }
              }
            }
            frame "North west" {
              w1827 = 1
              n241 = case shown="2" w1827 {
                tunnel: [w1831 w1837 w1845 w1853 w1861 w1870 w1877 w1886] -> w1826
                tunnel: [w1833 w1839 w1847 w1854 w1863 w1872 w1879 w1888] -> w1825
                tunnel: [w1832 w1838 w1846 w1855 w1862 w1871 w1878 w1887] -> w1824
                tunnel: w1827 -> [w1835 w1840 w1848 w1856 w1864 w1869 w1880 w1885]
                tunnel: w1823 -> [w1828 w1836 w1844 w1852 w1860 w1868 w1876 w1884]
                frame 0, Default {
                  n242 = Index Array(array=w1828, index (row) #1=w1835, index (col) #1=0, index (row) #2=w1835, index (col) #2=1, index (row) #3=w1835, index (col) #3=2) -> (element #1=w1833:dbl, element #2=w1832:dbl, element #3=w1831:dbl)
                }
                frame 1 {
                  n243 = Index Array(array=w1836, index (row) #1=w1840, index (col) #1=0, index (row) #2=w1840, index (col) #2=1, index (row) #3=w1840, index (col) #3=2) -> (element #1=w1839:dbl, element #2=w1838:dbl, element #3=w1837:dbl)
                }
                frame 2 {
                  n244 = Index Array(array=w1844, index (row) #1=w1848, index (col) #1=0, index (row) #2=w1848, index (col) #2=1, index (row) #3=w1848, index (col) #3=2) -> (element #1=w1847:dbl, element #2=w1846:dbl, element #3=w1845:dbl)
                }
                frame 3 {
                  n245 = Index Array(array=w1852, index (row) #1=w1856, index (col) #1=0, index (row) #2=w1856, index (col) #2=1, index (row) #3=w1856, index (col) #3=2) -> (element #1=w1854:dbl, element #2=w1855:dbl, element #3=w1853:dbl)
                }
                frame 4 {
                  n246 = Index Array(array=w1860, index (row) #1=w1864, index (col) #1=0, index (row) #2=w1864, index (col) #2=1, index (row) #3=w1864, index (col) #3=2) -> (element #1=w1861:dbl, element #2=w1863:dbl, element #3=w1862:dbl)
                }
                frame 5 {
                  n247 = Index Array(array=w1868, index (row) #1=w1869, index (col) #1=0, index (row) #2=w1869, index (col) #2=1, index (row) #3=w1869, index (col) #3=2) -> (element #1=w1870:dbl, element #2=w1871:dbl, element #3=w1872:dbl)
                }
                frame 6 {
                  n248 = Index Array(array=w1876, index (row) #1=w1880, index (col) #1=0, index (row) #2=w1880, index (col) #2=1, index (row) #3=w1880, index (col) #3=2) -> (element #1=w1877:dbl, element #2=w1879:dbl, element #3=w1878:dbl)
                }
                frame 7 {
                  n249 = Index Array(array=w1884, index (row) #1=w1885, index (col) #1=0, index (row) #2=w1885, index (col) #2=1, index (row) #3=w1885, index (col) #3=2) -> (element #1=w1886:dbl, element #2=w1888:dbl, element #3=w1887:dbl)
                }
              }
            }
            frame "West" {
              w1896 = 0
              n250 = case shown="2" w1896 {
                tunnel: [w1900 w1906 w1914 w1922 w1930 w1939 w1946 w1955] -> w1893
                tunnel: [w1902 w1908 w1916 w1923 w1932 w1941 w1948 w1957] -> w1894
                tunnel: [w1901 w1907 w1915 w1924 w1931 w1940 w1947 w1956] -> w1892
                tunnel: w1896 -> [w1904 w1909 w1917 w1925 w1933 w1938 w1949 w1954]
                tunnel: w1895 -> [w1897 w1905 w1913 w1921 w1929 w1937 w1945 w1953]
                frame 0, Default {
                  n251 = Index Array(array=w1897, index (row) #1=w1904, index (col) #1=0, index (row) #2=w1904, index (col) #2=1, index (row) #3=w1904, index (col) #3=2) -> (element #1=w1902:dbl, element #2=w1901:dbl, element #3=w1900:dbl)
                }
                frame 1 {
                  n252 = Index Array(array=w1905, index (row) #1=w1909, index (col) #1=0, index (row) #2=w1909, index (col) #2=1, index (row) #3=w1909, index (col) #3=2) -> (element #1=w1908:dbl, element #2=w1907:dbl, element #3=w1906:dbl)
                }
                frame 2 {
                  n253 = Index Array(array=w1913, index (row) #1=w1917, index (col) #1=0, index (row) #2=w1917, index (col) #2=1, index (row) #3=w1917, index (col) #3=2) -> (element #1=w1916:dbl, element #2=w1915:dbl, element #3=w1914:dbl)
                }
                frame 3 {
                  n254 = Index Array(array=w1921, index (row) #1=w1925, index (col) #1=0, index (row) #2=w1925, index (col) #2=1, index (row) #3=w1925, index (col) #3=2) -> (element #1=w1923:dbl, element #2=w1924:dbl, element #3=w1922:dbl)
                }
                frame 4 {
                  n255 = Index Array(array=w1929, index (row) #1=w1933, index (col) #1=0, index (row) #2=w1933, index (col) #2=1, index (row) #3=w1933, index (col) #3=2) -> (element #1=w1930:dbl, element #2=w1932:dbl, element #3=w1931:dbl)
                }
                frame 5 {
                  n256 = Index Array(array=w1937, index (row) #1=w1938, index (col) #1=0, index (row) #2=w1938, index (col) #2=1, index (row) #3=w1938, index (col) #3=2) -> (element #1=w1939:dbl, element #2=w1940:dbl, element #3=w1941:dbl)
                }
                frame 6 {
                  n257 = Index Array(array=w1945, index (row) #1=w1949, index (col) #1=0, index (row) #2=w1949, index (col) #2=1, index (row) #3=w1949, index (col) #3=2) -> (element #1=w1946:dbl, element #2=w1948:dbl, element #3=w1947:dbl)
                }
                frame 7 {
                  n258 = Index Array(array=w1953, index (row) #1=w1954, index (col) #1=0, index (row) #2=w1954, index (col) #2=1, index (row) #3=w1954, index (col) #3=2) -> (element #1=w1955:dbl, element #2=w1957:dbl, element #3=w1956:dbl)
                }
              }
            }
            frame "East" {
              w1965 = 7
              n259 = case shown="2" w1965 {
                tunnel: [w1969 w1975 w1983 w1991 w1999 w2008 w2015 w2024] -> w1963
                tunnel: [w1971 w1977 w1985 w1992 w2001 w2010 w2017 w2026] -> w1962
                tunnel: [w1970 w1976 w1984 w1993 w2000 w2009 w2016 w2025] -> w1961
                tunnel: w1965 -> [w1973 w1978 w1986 w1994 w2002 w2007 w2018 w2023]
                tunnel: w1964 -> [w1966 w1974 w1982 w1990 w1998 w2006 w2014 w2022]
                frame 0, Default {
                  n260 = Index Array(array=w1966, index (row) #1=w1973, index (col) #1=0, index (row) #2=w1973, index (col) #2=1, index (row) #3=w1973, index (col) #3=2) -> (element #1=w1971:dbl, element #2=w1970:dbl, element #3=w1969:dbl)
                }
                frame 1 {
                  n261 = Index Array(array=w1974, index (row) #1=w1978, index (col) #1=0, index (row) #2=w1978, index (col) #2=1, index (row) #3=w1978, index (col) #3=2) -> (element #1=w1977:dbl, element #2=w1976:dbl, element #3=w1975:dbl)
                }
                frame 2 {
                  n262 = Index Array(array=w1982, index (row) #1=w1986, index (col) #1=0, index (row) #2=w1986, index (col) #2=1, index (row) #3=w1986, index (col) #3=2) -> (element #1=w1985:dbl, element #2=w1984:dbl, element #3=w1983:dbl)
                }
                frame 3 {
                  n263 = Index Array(array=w1990, index (row) #1=w1994, index (col) #1=0, index (row) #2=w1994, index (col) #2=1, index (row) #3=w1994, index (col) #3=2) -> (element #1=w1992:dbl, element #2=w1993:dbl, element #3=w1991:dbl)
                }
                frame 4 {
                  n264 = Index Array(array=w1998, index (row) #1=w2002, index (col) #1=0, index (row) #2=w2002, index (col) #2=1, index (row) #3=w2002, index (col) #3=2) -> (element #1=w1999:dbl, element #2=w2001:dbl, element #3=w2000:dbl)
                }
                frame 5 {
                  n265 = Index Array(array=w2006, index (row) #1=w2007, index (col) #1=0, index (row) #2=w2007, index (col) #2=1, index (row) #3=w2007, index (col) #3=2) -> (element #1=w2008:dbl, element #2=w2009:dbl, element #3=w2010:dbl)
                }
                frame 6 {
                  n266 = Index Array(array=w2014, index (row) #1=w2018, index (col) #1=0, index (row) #2=w2018, index (col) #2=1, index (row) #3=w2018, index (col) #3=2) -> (element #1=w2015:dbl, element #2=w2017:dbl, element #3=w2016:dbl)
                }
                frame 7 {
                  n267 = Index Array(array=w2022, index (row) #1=w2023, index (col) #1=0, index (row) #2=w2023, index (col) #2=1, index (row) #3=w2023, index (col) #3=2) -> (element #1=w2024:dbl, element #2=w2026:dbl, element #3=w2025:dbl)
                }
              }
            }
            frame "South" {
              w2034 = 4
              n268 = case shown="2" w2034 {
                tunnel: [w2038 w2044 w2052 w2060 w2068 w2077 w2084 w2093] -> w2033
                tunnel: [w2040 w2046 w2054 w2061 w2070 w2079 w2086 w2095] -> w2031
                tunnel: [w2039 w2045 w2053 w2062 w2069 w2078 w2085 w2094] -> w2030
                tunnel: w2034 -> [w2042 w2047 w2055 w2063 w2071 w2076 w2087 w2092]
                tunnel: w2032 -> [w2035 w2043 w2051 w2059 w2067 w2075 w2083 w2091]
                frame 0, Default {
                  n269 = Index Array(array=w2035, index (row) #1=w2042, index (col) #1=0, index (row) #2=w2042, index (col) #2=1, index (row) #3=w2042, index (col) #3=2) -> (element #1=w2040:dbl, element #2=w2039:dbl, element #3=w2038:dbl)
                }
                frame 1 {
                  n270 = Index Array(array=w2043, index (row) #1=w2047, index (col) #1=0, index (row) #2=w2047, index (col) #2=1, index (row) #3=w2047, index (col) #3=2) -> (element #1=w2046:dbl, element #2=w2045:dbl, element #3=w2044:dbl)
                }
                frame 2 {
                  n271 = Index Array(array=w2051, index (row) #1=w2055, index (col) #1=0, index (row) #2=w2055, index (col) #2=1, index (row) #3=w2055, index (col) #3=2) -> (element #1=w2054:dbl, element #2=w2053:dbl, element #3=w2052:dbl)
                }
                frame 3 {
                  n272 = Index Array(array=w2059, index (row) #1=w2063, index (col) #1=0, index (row) #2=w2063, index (col) #2=1, index (row) #3=w2063, index (col) #3=2) -> (element #1=w2061:dbl, element #2=w2062:dbl, element #3=w2060:dbl)
                }
                frame 4 {
                  n273 = Index Array(array=w2067, index (row) #1=w2071, index (col) #1=0, index (row) #2=w2071, index (col) #2=1, index (row) #3=w2071, index (col) #3=2) -> (element #1=w2068:dbl, element #2=w2070:dbl, element #3=w2069:dbl)
                }
                frame 5 {
                  n274 = Index Array(array=w2075, index (row) #1=w2076, index (col) #1=0, index (row) #2=w2076, index (col) #2=1, index (row) #3=w2076, index (col) #3=2) -> (element #1=w2077:dbl, element #2=w2078:dbl, element #3=w2079:dbl)
                }
                frame 6 {
                  n275 = Index Array(array=w2083, index (row) #1=w2087, index (col) #1=0, index (row) #2=w2087, index (col) #2=1, index (row) #3=w2087, index (col) #3=2) -> (element #1=w2084:dbl, element #2=w2086:dbl, element #3=w2085:dbl)
                }
                frame 7 {
                  n276 = Index Array(array=w2091, index (row) #1=w2092, index (col) #1=0, index (row) #2=w2092, index (col) #2=1, index (row) #3=w2092, index (col) #3=2) -> (element #1=w2093:dbl, element #2=w2095:dbl, element #3=w2094:dbl)
                }
              }
            }
            frame "South west" {
              w2103 = 2
              n277 = case shown="2" w2103 {
                tunnel: [w2107 w2113 w2121 w2129 w2137 w2146 w2153 w2162] -> w2101
                tunnel: [w2109 w2115 w2123 w2130 w2139 w2148 w2155 w2164] -> w2100
                tunnel: [w2108 w2114 w2122 w2131 w2138 w2147 w2154 w2163] -> w2099
                tunnel: w2103 -> [w2111 w2116 w2124 w2132 w2140 w2145 w2156 w2161]
                tunnel: w2102 -> [w2104 w2112 w2120 w2128 w2136 w2144 w2152 w2160]
                frame 0, Default {
                  n278 = Index Array(array=w2104, index (row) #1=w2111, index (col) #1=0, index (row) #2=w2111, index (col) #2=1, index (row) #3=w2111, index (col) #3=2) -> (element #1=w2109:dbl, element #2=w2108:dbl, element #3=w2107:dbl)
                }
                frame 1 {
                  n279 = Index Array(array=w2112, index (row) #1=w2116, index (col) #1=0, index (row) #2=w2116, index (col) #2=1, index (row) #3=w2116, index (col) #3=2) -> (element #1=w2115:dbl, element #2=w2114:dbl, element #3=w2113:dbl)
                }
                frame 2 {
                  n280 = Index Array(array=w2120, index (row) #1=w2124, index (col) #1=0, index (row) #2=w2124, index (col) #2=1, index (row) #3=w2124, index (col) #3=2) -> (element #1=w2123:dbl, element #2=w2122:dbl, element #3=w2121:dbl)
                }
                frame 3 {
                  n281 = Index Array(array=w2128, index (row) #1=w2132, index (col) #1=0, index (row) #2=w2132, index (col) #2=1, index (row) #3=w2132, index (col) #3=2) -> (element #1=w2130:dbl, element #2=w2131:dbl, element #3=w2129:dbl)
                }
                frame 4 {
                  n282 = Index Array(array=w2136, index (row) #1=w2140, index (col) #1=0, index (row) #2=w2140, index (col) #2=1, index (row) #3=w2140, index (col) #3=2) -> (element #1=w2137:dbl, element #2=w2139:dbl, element #3=w2138:dbl)
                }
                frame 5 {
                  n283 = Index Array(array=w2144, index (row) #1=w2145, index (col) #1=0, index (row) #2=w2145, index (col) #2=1, index (row) #3=w2145, index (col) #3=2) -> (element #1=w2146:dbl, element #2=w2147:dbl, element #3=w2148:dbl)
                }
                frame 6 {
                  n284 = Index Array(array=w2152, index (row) #1=w2156, index (col) #1=0, index (row) #2=w2156, index (col) #2=1, index (row) #3=w2156, index (col) #3=2) -> (element #1=w2153:dbl, element #2=w2155:dbl, element #3=w2154:dbl)
                }
                frame 7 {
                  n285 = Index Array(array=w2160, index (row) #1=w2161, index (col) #1=0, index (row) #2=w2161, index (col) #2=1, index (row) #3=w2161, index (col) #3=2) -> (element #1=w2162:dbl, element #2=w2164:dbl, element #3=w2163:dbl)
                }
              }
            }
            frame "South east" {
              w2172 = 6
              n286 = case shown="2" w2172 {
                tunnel: [w2176 w2182 w2190 w2198 w2206 w2215 w2222 w2231] -> w2171
                tunnel: [w2178 w2184 w2192 w2199 w2208 w2217 w2224 w2233] -> w2170
                tunnel: [w2177 w2183 w2191 w2200 w2207 w2216 w2223 w2232] -> w2169
                tunnel: w2172 -> [w2180 w2185 w2193 w2201 w2209 w2214 w2225 w2230]
                tunnel: w2168 -> [w2173 w2181 w2189 w2197 w2205 w2213 w2221 w2229]
                frame 0, Default {
                  n287 = Index Array(array=w2173, index (row) #1=w2180, index (col) #1=0, index (row) #2=w2180, index (col) #2=1, index (row) #3=w2180, index (col) #3=2) -> (element #1=w2178:dbl, element #2=w2177:dbl, element #3=w2176:dbl)
                }
                frame 1 {
                  n288 = Index Array(array=w2181, index (row) #1=w2185, index (col) #1=0, index (row) #2=w2185, index (col) #2=1, index (row) #3=w2185, index (col) #3=2) -> (element #1=w2184:dbl, element #2=w2183:dbl, element #3=w2182:dbl)
                }
                frame 2 {
                  n289 = Index Array(array=w2189, index (row) #1=w2193, index (col) #1=0, index (row) #2=w2193, index (col) #2=1, index (row) #3=w2193, index (col) #3=2) -> (element #1=w2192:dbl, element #2=w2191:dbl, element #3=w2190:dbl)
                }
                frame 3 {
                  n290 = Index Array(array=w2197, index (row) #1=w2201, index (col) #1=0, index (row) #2=w2201, index (col) #2=1, index (row) #3=w2201, index (col) #3=2) -> (element #1=w2199:dbl, element #2=w2200:dbl, element #3=w2198:dbl)
                }
                frame 4 {
                  n291 = Index Array(array=w2205, index (row) #1=w2209, index (col) #1=0, index (row) #2=w2209, index (col) #2=1, index (row) #3=w2209, index (col) #3=2) -> (element #1=w2206:dbl, element #2=w2208:dbl, element #3=w2207:dbl)
                }
                frame 5 {
                  n292 = Index Array(array=w2213, index (row) #1=w2214, index (col) #1=0, index (row) #2=w2214, index (col) #2=1, index (row) #3=w2214, index (col) #3=2) -> (element #1=w2215:dbl, element #2=w2216:dbl, element #3=w2217:dbl)
                }
                frame 6 {
                  n293 = Index Array(array=w2221, index (row) #1=w2225, index (col) #1=0, index (row) #2=w2225, index (col) #2=1, index (row) #3=w2225, index (col) #3=2) -> (element #1=w2222:dbl, element #2=w2224:dbl, element #3=w2223:dbl)
                }
                frame 7 {
                  n294 = Index Array(array=w2229, index (row) #1=w2230, index (col) #1=0, index (row) #2=w2230, index (col) #2=1, index (row) #3=w2230, index (col) #3=2) -> (element #1=w2231:dbl, element #2=w2233:dbl, element #3=w2232:dbl)
                }
              }
            }
          }
        }
        frame "East" {
          n295 = case shown="\"North\", Default" w2240 {
            tunnel: [w2245 w2315 w2383 w2450 w2520 w2590 w2658 w2728] -> w2239
            tunnel: [w2244 w2314 w2382 w2451 w2519 w2588 w2657 w2727] -> w2238
            tunnel: [w2243 w2313 w2381 w2449 w2518 w2587 w2656 w2726] -> w2237
            tunnel: w2241 -> [w2242 w2311 w2380 w2452 w2521 w2589 w2659 w2725]
            frame "North", Default {
              w2246 = 4
              n296 = case shown="2" w2246 {
                tunnel: [w2250 w2256 w2264 w2272 w2280 w2289 w2296 w2305] -> w2245
                tunnel: [w2252 w2258 w2266 w2273 w2282 w2291 w2298 w2307] -> w2244
                tunnel: [w2251 w2257 w2265 w2274 w2281 w2290 w2297 w2306] -> w2243
                tunnel: w2246 -> [w2254 w2259 w2267 w2275 w2283 w2288 w2299 w2304]
                tunnel: w2242 -> [w2247 w2255 w2263 w2271 w2279 w2287 w2295 w2303]
                frame 0, Default {
                  n297 = Index Array(array=w2247, index (row) #1=w2254, index (col) #1=0, index (row) #2=w2254, index (col) #2=1, index (row) #3=w2254, index (col) #3=2) -> (element #1=w2252:dbl, element #2=w2251:dbl, element #3=w2250:dbl)
                }
                frame 1 {
                  n298 = Index Array(array=w2255, index (row) #1=w2259, index (col) #1=0, index (row) #2=w2259, index (col) #2=1, index (row) #3=w2259, index (col) #3=2) -> (element #1=w2258:dbl, element #2=w2257:dbl, element #3=w2256:dbl)
                }
                frame 2 {
                  n299 = Index Array(array=w2263, index (row) #1=w2267, index (col) #1=0, index (row) #2=w2267, index (col) #2=1, index (row) #3=w2267, index (col) #3=2) -> (element #1=w2266:dbl, element #2=w2265:dbl, element #3=w2264:dbl)
                }
                frame 3 {
                  n300 = Index Array(array=w2271, index (row) #1=w2275, index (col) #1=0, index (row) #2=w2275, index (col) #2=1, index (row) #3=w2275, index (col) #3=2) -> (element #1=w2273:dbl, element #2=w2274:dbl, element #3=w2272:dbl)
                }
                frame 4 {
                  n301 = Index Array(array=w2279, index (row) #1=w2283, index (col) #1=0, index (row) #2=w2283, index (col) #2=1, index (row) #3=w2283, index (col) #3=2) -> (element #1=w2280:dbl, element #2=w2282:dbl, element #3=w2281:dbl)
                }
                frame 5 {
                  n302 = Index Array(array=w2287, index (row) #1=w2288, index (col) #1=0, index (row) #2=w2288, index (col) #2=1, index (row) #3=w2288, index (col) #3=2) -> (element #1=w2289:dbl, element #2=w2290:dbl, element #3=w2291:dbl)
                }
                frame 6 {
                  n303 = Index Array(array=w2295, index (row) #1=w2299, index (col) #1=0, index (row) #2=w2299, index (col) #2=1, index (row) #3=w2299, index (col) #3=2) -> (element #1=w2296:dbl, element #2=w2298:dbl, element #3=w2297:dbl)
                }
                frame 7 {
                  n304 = Index Array(array=w2303, index (row) #1=w2304, index (col) #1=0, index (row) #2=w2304, index (col) #2=1, index (row) #3=w2304, index (col) #3=2) -> (element #1=w2305:dbl, element #2=w2307:dbl, element #3=w2306:dbl)
                }
              }
            }
            frame "North east" {
              w2312 = 2
              n305 = case shown="2" w2312 {
                tunnel: [w2319 w2325 w2333 w2341 w2349 w2358 w2365 w2374] -> w2315
                tunnel: [w2321 w2327 w2335 w2342 w2351 w2360 w2367 w2376] -> w2314
                tunnel: [w2320 w2326 w2334 w2343 w2350 w2359 w2366 w2375] -> w2313
                tunnel: w2312 -> [w2323 w2328 w2336 w2344 w2352 w2357 w2368 w2373]
                tunnel: w2311 -> [w2316 w2324 w2332 w2340 w2348 w2356 w2364 w2372]
                frame 0, Default {
                  n306 = Index Array(array=w2316, index (row) #1=w2323, index (col) #1=0, index (row) #2=w2323, index (col) #2=1, index (row) #3=w2323, index (col) #3=2) -> (element #1=w2321:dbl, element #2=w2320:dbl, element #3=w2319:dbl)
                }
                frame 1 {
                  n307 = Index Array(array=w2324, index (row) #1=w2328, index (col) #1=0, index (row) #2=w2328, index (col) #2=1, index (row) #3=w2328, index (col) #3=2) -> (element #1=w2327:dbl, element #2=w2326:dbl, element #3=w2325:dbl)
                }
                frame 2 {
                  n308 = Index Array(array=w2332, index (row) #1=w2336, index (col) #1=0, index (row) #2=w2336, index (col) #2=1, index (row) #3=w2336, index (col) #3=2) -> (element #1=w2335:dbl, element #2=w2334:dbl, element #3=w2333:dbl)
                }
                frame 3 {
                  n309 = Index Array(array=w2340, index (row) #1=w2344, index (col) #1=0, index (row) #2=w2344, index (col) #2=1, index (row) #3=w2344, index (col) #3=2) -> (element #1=w2342:dbl, element #2=w2343:dbl, element #3=w2341:dbl)
                }
                frame 4 {
                  n310 = Index Array(array=w2348, index (row) #1=w2352, index (col) #1=0, index (row) #2=w2352, index (col) #2=1, index (row) #3=w2352, index (col) #3=2) -> (element #1=w2349:dbl, element #2=w2351:dbl, element #3=w2350:dbl)
                }
                frame 5 {
                  n311 = Index Array(array=w2356, index (row) #1=w2357, index (col) #1=0, index (row) #2=w2357, index (col) #2=1, index (row) #3=w2357, index (col) #3=2) -> (element #1=w2358:dbl, element #2=w2359:dbl, element #3=w2360:dbl)
                }
                frame 6 {
                  n312 = Index Array(array=w2364, index (row) #1=w2368, index (col) #1=0, index (row) #2=w2368, index (col) #2=1, index (row) #3=w2368, index (col) #3=2) -> (element #1=w2365:dbl, element #2=w2367:dbl, element #3=w2366:dbl)
                }
                frame 7 {
                  n313 = Index Array(array=w2372, index (row) #1=w2373, index (col) #1=0, index (row) #2=w2373, index (col) #2=1, index (row) #3=w2373, index (col) #3=2) -> (element #1=w2374:dbl, element #2=w2376:dbl, element #3=w2375:dbl)
                }
              }
            }
            frame "North west" {
              w2384 = 6
              n314 = case shown="2" w2384 {
                tunnel: [w2388 w2394 w2402 w2410 w2418 w2427 w2434 w2443] -> w2383
                tunnel: [w2390 w2396 w2404 w2411 w2420 w2429 w2436 w2445] -> w2382
                tunnel: [w2389 w2395 w2403 w2412 w2419 w2428 w2435 w2444] -> w2381
                tunnel: w2384 -> [w2392 w2397 w2405 w2413 w2421 w2426 w2437 w2442]
                tunnel: w2380 -> [w2385 w2393 w2401 w2409 w2417 w2425 w2433 w2441]
                frame 0, Default {
                  n315 = Index Array(array=w2385, index (row) #1=w2392, index (col) #1=0, index (row) #2=w2392, index (col) #2=1, index (row) #3=w2392, index (col) #3=2) -> (element #1=w2390:dbl, element #2=w2389:dbl, element #3=w2388:dbl)
                }
                frame 1 {
                  n316 = Index Array(array=w2393, index (row) #1=w2397, index (col) #1=0, index (row) #2=w2397, index (col) #2=1, index (row) #3=w2397, index (col) #3=2) -> (element #1=w2396:dbl, element #2=w2395:dbl, element #3=w2394:dbl)
                }
                frame 2 {
                  n317 = Index Array(array=w2401, index (row) #1=w2405, index (col) #1=0, index (row) #2=w2405, index (col) #2=1, index (row) #3=w2405, index (col) #3=2) -> (element #1=w2404:dbl, element #2=w2403:dbl, element #3=w2402:dbl)
                }
                frame 3 {
                  n318 = Index Array(array=w2409, index (row) #1=w2413, index (col) #1=0, index (row) #2=w2413, index (col) #2=1, index (row) #3=w2413, index (col) #3=2) -> (element #1=w2411:dbl, element #2=w2412:dbl, element #3=w2410:dbl)
                }
                frame 4 {
                  n319 = Index Array(array=w2417, index (row) #1=w2421, index (col) #1=0, index (row) #2=w2421, index (col) #2=1, index (row) #3=w2421, index (col) #3=2) -> (element #1=w2418:dbl, element #2=w2420:dbl, element #3=w2419:dbl)
                }
                frame 5 {
                  n320 = Index Array(array=w2425, index (row) #1=w2426, index (col) #1=0, index (row) #2=w2426, index (col) #2=1, index (row) #3=w2426, index (col) #3=2) -> (element #1=w2427:dbl, element #2=w2428:dbl, element #3=w2429:dbl)
                }
                frame 6 {
                  n321 = Index Array(array=w2433, index (row) #1=w2437, index (col) #1=0, index (row) #2=w2437, index (col) #2=1, index (row) #3=w2437, index (col) #3=2) -> (element #1=w2434:dbl, element #2=w2436:dbl, element #3=w2435:dbl)
                }
                frame 7 {
                  n322 = Index Array(array=w2441, index (row) #1=w2442, index (col) #1=0, index (row) #2=w2442, index (col) #2=1, index (row) #3=w2442, index (col) #3=2) -> (element #1=w2443:dbl, element #2=w2445:dbl, element #3=w2444:dbl)
                }
              }
            }
            frame "West" {
              w2453 = 7
              n323 = case shown="2" w2453 {
                tunnel: [w2457 w2463 w2471 w2479 w2487 w2496 w2503 w2512] -> w2450
                tunnel: [w2459 w2465 w2473 w2480 w2489 w2498 w2505 w2514] -> w2451
                tunnel: [w2458 w2464 w2472 w2481 w2488 w2497 w2504 w2513] -> w2449
                tunnel: w2453 -> [w2461 w2466 w2474 w2482 w2490 w2495 w2506 w2511]
                tunnel: w2452 -> [w2454 w2462 w2470 w2478 w2486 w2494 w2502 w2510]
                frame 0, Default {
                  n324 = Index Array(array=w2454, index (row) #1=w2461, index (col) #1=0, index (row) #2=w2461, index (col) #2=1, index (row) #3=w2461, index (col) #3=2) -> (element #1=w2459:dbl, element #2=w2458:dbl, element #3=w2457:dbl)
                }
                frame 1 {
                  n325 = Index Array(array=w2462, index (row) #1=w2466, index (col) #1=0, index (row) #2=w2466, index (col) #2=1, index (row) #3=w2466, index (col) #3=2) -> (element #1=w2465:dbl, element #2=w2464:dbl, element #3=w2463:dbl)
                }
                frame 2 {
                  n326 = Index Array(array=w2470, index (row) #1=w2474, index (col) #1=0, index (row) #2=w2474, index (col) #2=1, index (row) #3=w2474, index (col) #3=2) -> (element #1=w2473:dbl, element #2=w2472:dbl, element #3=w2471:dbl)
                }
                frame 3 {
                  n327 = Index Array(array=w2478, index (row) #1=w2482, index (col) #1=0, index (row) #2=w2482, index (col) #2=1, index (row) #3=w2482, index (col) #3=2) -> (element #1=w2480:dbl, element #2=w2481:dbl, element #3=w2479:dbl)
                }
                frame 4 {
                  n328 = Index Array(array=w2486, index (row) #1=w2490, index (col) #1=0, index (row) #2=w2490, index (col) #2=1, index (row) #3=w2490, index (col) #3=2) -> (element #1=w2487:dbl, element #2=w2489:dbl, element #3=w2488:dbl)
                }
                frame 5 {
                  n329 = Index Array(array=w2494, index (row) #1=w2495, index (col) #1=0, index (row) #2=w2495, index (col) #2=1, index (row) #3=w2495, index (col) #3=2) -> (element #1=w2496:dbl, element #2=w2497:dbl, element #3=w2498:dbl)
                }
                frame 6 {
                  n330 = Index Array(array=w2502, index (row) #1=w2506, index (col) #1=0, index (row) #2=w2506, index (col) #2=1, index (row) #3=w2506, index (col) #3=2) -> (element #1=w2503:dbl, element #2=w2505:dbl, element #3=w2504:dbl)
                }
                frame 7 {
                  n331 = Index Array(array=w2510, index (row) #1=w2511, index (col) #1=0, index (row) #2=w2511, index (col) #2=1, index (row) #3=w2511, index (col) #3=2) -> (element #1=w2512:dbl, element #2=w2514:dbl, element #3=w2513:dbl)
                }
              }
            }
            frame "East" {
              w2522 = 0
              n332 = case shown="2" w2522 {
                tunnel: [w2526 w2532 w2540 w2548 w2556 w2565 w2572 w2581] -> w2520
                tunnel: [w2528 w2534 w2542 w2549 w2558 w2567 w2574 w2583] -> w2519
                tunnel: [w2527 w2533 w2541 w2550 w2557 w2566 w2573 w2582] -> w2518
                tunnel: w2522 -> [w2530 w2535 w2543 w2551 w2559 w2564 w2575 w2580]
                tunnel: w2521 -> [w2523 w2531 w2539 w2547 w2555 w2563 w2571 w2579]
                frame 0, Default {
                  n333 = Index Array(array=w2523, index (row) #1=w2530, index (col) #1=0, index (row) #2=w2530, index (col) #2=1, index (row) #3=w2530, index (col) #3=2) -> (element #1=w2528:dbl, element #2=w2527:dbl, element #3=w2526:dbl)
                }
                frame 1 {
                  n334 = Index Array(array=w2531, index (row) #1=w2535, index (col) #1=0, index (row) #2=w2535, index (col) #2=1, index (row) #3=w2535, index (col) #3=2) -> (element #1=w2534:dbl, element #2=w2533:dbl, element #3=w2532:dbl)
                }
                frame 2 {
                  n335 = Index Array(array=w2539, index (row) #1=w2543, index (col) #1=0, index (row) #2=w2543, index (col) #2=1, index (row) #3=w2543, index (col) #3=2) -> (element #1=w2542:dbl, element #2=w2541:dbl, element #3=w2540:dbl)
                }
                frame 3 {
                  n336 = Index Array(array=w2547, index (row) #1=w2551, index (col) #1=0, index (row) #2=w2551, index (col) #2=1, index (row) #3=w2551, index (col) #3=2) -> (element #1=w2549:dbl, element #2=w2550:dbl, element #3=w2548:dbl)
                }
                frame 4 {
                  n337 = Index Array(array=w2555, index (row) #1=w2559, index (col) #1=0, index (row) #2=w2559, index (col) #2=1, index (row) #3=w2559, index (col) #3=2) -> (element #1=w2556:dbl, element #2=w2558:dbl, element #3=w2557:dbl)
                }
                frame 5 {
                  n338 = Index Array(array=w2563, index (row) #1=w2564, index (col) #1=0, index (row) #2=w2564, index (col) #2=1, index (row) #3=w2564, index (col) #3=2) -> (element #1=w2565:dbl, element #2=w2566:dbl, element #3=w2567:dbl)
                }
                frame 6 {
                  n339 = Index Array(array=w2571, index (row) #1=w2575, index (col) #1=0, index (row) #2=w2575, index (col) #2=1, index (row) #3=w2575, index (col) #3=2) -> (element #1=w2572:dbl, element #2=w2574:dbl, element #3=w2573:dbl)
                }
                frame 7 {
                  n340 = Index Array(array=w2579, index (row) #1=w2580, index (col) #1=0, index (row) #2=w2580, index (col) #2=1, index (row) #3=w2580, index (col) #3=2) -> (element #1=w2581:dbl, element #2=w2583:dbl, element #3=w2582:dbl)
                }
              }
            }
            frame "South" {
              w2591 = 3
              n341 = case shown="2" w2591 {
                tunnel: [w2595 w2601 w2609 w2617 w2625 w2634 w2641 w2650] -> w2590
                tunnel: [w2597 w2603 w2611 w2618 w2627 w2636 w2643 w2652] -> w2588
                tunnel: [w2596 w2602 w2610 w2619 w2626 w2635 w2642 w2651] -> w2587
                tunnel: w2591 -> [w2599 w2604 w2612 w2620 w2628 w2633 w2644 w2649]
                tunnel: w2589 -> [w2592 w2600 w2608 w2616 w2624 w2632 w2640 w2648]
                frame 0, Default {
                  n342 = Index Array(array=w2592, index (row) #1=w2599, index (col) #1=0, index (row) #2=w2599, index (col) #2=1, index (row) #3=w2599, index (col) #3=2) -> (element #1=w2597:dbl, element #2=w2596:dbl, element #3=w2595:dbl)
                }
                frame 1 {
                  n343 = Index Array(array=w2600, index (row) #1=w2604, index (col) #1=0, index (row) #2=w2604, index (col) #2=1, index (row) #3=w2604, index (col) #3=2) -> (element #1=w2603:dbl, element #2=w2602:dbl, element #3=w2601:dbl)
                }
                frame 2 {
                  n344 = Index Array(array=w2608, index (row) #1=w2612, index (col) #1=0, index (row) #2=w2612, index (col) #2=1, index (row) #3=w2612, index (col) #3=2) -> (element #1=w2611:dbl, element #2=w2610:dbl, element #3=w2609:dbl)
                }
                frame 3 {
                  n345 = Index Array(array=w2616, index (row) #1=w2620, index (col) #1=0, index (row) #2=w2620, index (col) #2=1, index (row) #3=w2620, index (col) #3=2) -> (element #1=w2618:dbl, element #2=w2619:dbl, element #3=w2617:dbl)
                }
                frame 4 {
                  n346 = Index Array(array=w2624, index (row) #1=w2628, index (col) #1=0, index (row) #2=w2628, index (col) #2=1, index (row) #3=w2628, index (col) #3=2) -> (element #1=w2625:dbl, element #2=w2627:dbl, element #3=w2626:dbl)
                }
                frame 5 {
                  n347 = Index Array(array=w2632, index (row) #1=w2633, index (col) #1=0, index (row) #2=w2633, index (col) #2=1, index (row) #3=w2633, index (col) #3=2) -> (element #1=w2634:dbl, element #2=w2635:dbl, element #3=w2636:dbl)
                }
                frame 6 {
                  n348 = Index Array(array=w2640, index (row) #1=w2644, index (col) #1=0, index (row) #2=w2644, index (col) #2=1, index (row) #3=w2644, index (col) #3=2) -> (element #1=w2641:dbl, element #2=w2643:dbl, element #3=w2642:dbl)
                }
                frame 7 {
                  n349 = Index Array(array=w2648, index (row) #1=w2649, index (col) #1=0, index (row) #2=w2649, index (col) #2=1, index (row) #3=w2649, index (col) #3=2) -> (element #1=w2650:dbl, element #2=w2652:dbl, element #3=w2651:dbl)
                }
              }
            }
            frame "South west" {
              w2660 = 5
              n350 = case shown="2" w2660 {
                tunnel: [w2664 w2670 w2678 w2686 w2694 w2703 w2710 w2719] -> w2658
                tunnel: [w2666 w2672 w2680 w2687 w2696 w2705 w2712 w2721] -> w2657
                tunnel: [w2665 w2671 w2679 w2688 w2695 w2704 w2711 w2720] -> w2656
                tunnel: w2660 -> [w2668 w2673 w2681 w2689 w2697 w2702 w2713 w2718]
                tunnel: w2659 -> [w2661 w2669 w2677 w2685 w2693 w2701 w2709 w2717]
                frame 0, Default {
                  n351 = Index Array(array=w2661, index (row) #1=w2668, index (col) #1=0, index (row) #2=w2668, index (col) #2=1, index (row) #3=w2668, index (col) #3=2) -> (element #1=w2666:dbl, element #2=w2665:dbl, element #3=w2664:dbl)
                }
                frame 1 {
                  n352 = Index Array(array=w2669, index (row) #1=w2673, index (col) #1=0, index (row) #2=w2673, index (col) #2=1, index (row) #3=w2673, index (col) #3=2) -> (element #1=w2672:dbl, element #2=w2671:dbl, element #3=w2670:dbl)
                }
                frame 2 {
                  n353 = Index Array(array=w2677, index (row) #1=w2681, index (col) #1=0, index (row) #2=w2681, index (col) #2=1, index (row) #3=w2681, index (col) #3=2) -> (element #1=w2680:dbl, element #2=w2679:dbl, element #3=w2678:dbl)
                }
                frame 3 {
                  n354 = Index Array(array=w2685, index (row) #1=w2689, index (col) #1=0, index (row) #2=w2689, index (col) #2=1, index (row) #3=w2689, index (col) #3=2) -> (element #1=w2687:dbl, element #2=w2688:dbl, element #3=w2686:dbl)
                }
                frame 4 {
                  n355 = Index Array(array=w2693, index (row) #1=w2697, index (col) #1=0, index (row) #2=w2697, index (col) #2=1, index (row) #3=w2697, index (col) #3=2) -> (element #1=w2694:dbl, element #2=w2696:dbl, element #3=w2695:dbl)
                }
                frame 5 {
                  n356 = Index Array(array=w2701, index (row) #1=w2702, index (col) #1=0, index (row) #2=w2702, index (col) #2=1, index (row) #3=w2702, index (col) #3=2) -> (element #1=w2703:dbl, element #2=w2704:dbl, element #3=w2705:dbl)
                }
                frame 6 {
                  n357 = Index Array(array=w2709, index (row) #1=w2713, index (col) #1=0, index (row) #2=w2713, index (col) #2=1, index (row) #3=w2713, index (col) #3=2) -> (element #1=w2710:dbl, element #2=w2712:dbl, element #3=w2711:dbl)
                }
                frame 7 {
                  n358 = Index Array(array=w2717, index (row) #1=w2718, index (col) #1=0, index (row) #2=w2718, index (col) #2=1, index (row) #3=w2718, index (col) #3=2) -> (element #1=w2719:dbl, element #2=w2721:dbl, element #3=w2720:dbl)
                }
              }
            }
            frame "South east" {
              w2729 = 1
              n359 = case shown="2" w2729 {
                tunnel: [w2733 w2739 w2747 w2755 w2763 w2772 w2779 w2788] -> w2728
                tunnel: [w2735 w2741 w2749 w2756 w2765 w2774 w2781 w2790] -> w2727
                tunnel: [w2734 w2740 w2748 w2757 w2764 w2773 w2780 w2789] -> w2726
                tunnel: w2729 -> [w2737 w2742 w2750 w2758 w2766 w2771 w2782 w2787]
                tunnel: w2725 -> [w2730 w2738 w2746 w2754 w2762 w2770 w2778 w2786]
                frame 0, Default {
                  n360 = Index Array(array=w2730, index (row) #1=w2737, index (col) #1=0, index (row) #2=w2737, index (col) #2=1, index (row) #3=w2737, index (col) #3=2) -> (element #1=w2735:dbl, element #2=w2734:dbl, element #3=w2733:dbl)
                }
                frame 1 {
                  n361 = Index Array(array=w2738, index (row) #1=w2742, index (col) #1=0, index (row) #2=w2742, index (col) #2=1, index (row) #3=w2742, index (col) #3=2) -> (element #1=w2741:dbl, element #2=w2740:dbl, element #3=w2739:dbl)
                }
                frame 2 {
                  n362 = Index Array(array=w2746, index (row) #1=w2750, index (col) #1=0, index (row) #2=w2750, index (col) #2=1, index (row) #3=w2750, index (col) #3=2) -> (element #1=w2749:dbl, element #2=w2748:dbl, element #3=w2747:dbl)
                }
                frame 3 {
                  n363 = Index Array(array=w2754, index (row) #1=w2758, index (col) #1=0, index (row) #2=w2758, index (col) #2=1, index (row) #3=w2758, index (col) #3=2) -> (element #1=w2756:dbl, element #2=w2757:dbl, element #3=w2755:dbl)
                }
                frame 4 {
                  n364 = Index Array(array=w2762, index (row) #1=w2766, index (col) #1=0, index (row) #2=w2766, index (col) #2=1, index (row) #3=w2766, index (col) #3=2) -> (element #1=w2763:dbl, element #2=w2765:dbl, element #3=w2764:dbl)
                }
                frame 5 {
                  n365 = Index Array(array=w2770, index (row) #1=w2771, index (col) #1=0, index (row) #2=w2771, index (col) #2=1, index (row) #3=w2771, index (col) #3=2) -> (element #1=w2772:dbl, element #2=w2773:dbl, element #3=w2774:dbl)
                }
                frame 6 {
                  n366 = Index Array(array=w2778, index (row) #1=w2782, index (col) #1=0, index (row) #2=w2782, index (col) #2=1, index (row) #3=w2782, index (col) #3=2) -> (element #1=w2779:dbl, element #2=w2781:dbl, element #3=w2780:dbl)
                }
                frame 7 {
                  n367 = Index Array(array=w2786, index (row) #1=w2787, index (col) #1=0, index (row) #2=w2787, index (col) #2=1, index (row) #3=w2787, index (col) #3=2) -> (element #1=w2788:dbl, element #2=w2790:dbl, element #3=w2789:dbl)
                }
              }
            }
          }
        }
        frame "South" {
          n368 = case shown="\"North\", Default" w2797 {
            tunnel: [w2802 w2872 w2940 w3007 w3077 w3147 w3215 w3285] -> w2796
            tunnel: [w2801 w2871 w2939 w3008 w3076 w3145 w3214 w3284] -> w2795
            tunnel: [w2800 w2870 w2938 w3006 w3075 w3144 w3213 w3283] -> w2794
            tunnel: w2798 -> [w2799 w2868 w2937 w3009 w3078 w3146 w3216 w3282]
            frame "North", Default {
              w2803 = 7
              n369 = case shown="2" w2803 {
                tunnel: [w2807 w2813 w2821 w2829 w2837 w2846 w2853 w2862] -> w2802
                tunnel: [w2809 w2815 w2823 w2830 w2839 w2848 w2855 w2864] -> w2801
                tunnel: [w2808 w2814 w2822 w2831 w2838 w2847 w2854 w2863] -> w2800
                tunnel: w2803 -> [w2811 w2816 w2824 w2832 w2840 w2845 w2856 w2861]
                tunnel: w2799 -> [w2804 w2812 w2820 w2828 w2836 w2844 w2852 w2860]
                frame 0, Default {
                  n370 = Index Array(array=w2804, index (row) #1=w2811, index (col) #1=0, index (row) #2=w2811, index (col) #2=1, index (row) #3=w2811, index (col) #3=2) -> (element #1=w2809:dbl, element #2=w2808:dbl, element #3=w2807:dbl)
                }
                frame 1 {
                  n371 = Index Array(array=w2812, index (row) #1=w2816, index (col) #1=0, index (row) #2=w2816, index (col) #2=1, index (row) #3=w2816, index (col) #3=2) -> (element #1=w2815:dbl, element #2=w2814:dbl, element #3=w2813:dbl)
                }
                frame 2 {
                  n372 = Index Array(array=w2820, index (row) #1=w2824, index (col) #1=0, index (row) #2=w2824, index (col) #2=1, index (row) #3=w2824, index (col) #3=2) -> (element #1=w2823:dbl, element #2=w2822:dbl, element #3=w2821:dbl)
                }
                frame 3 {
                  n373 = Index Array(array=w2828, index (row) #1=w2832, index (col) #1=0, index (row) #2=w2832, index (col) #2=1, index (row) #3=w2832, index (col) #3=2) -> (element #1=w2830:dbl, element #2=w2831:dbl, element #3=w2829:dbl)
                }
                frame 4 {
                  n374 = Index Array(array=w2836, index (row) #1=w2840, index (col) #1=0, index (row) #2=w2840, index (col) #2=1, index (row) #3=w2840, index (col) #3=2) -> (element #1=w2837:dbl, element #2=w2839:dbl, element #3=w2838:dbl)
                }
                frame 5 {
                  n375 = Index Array(array=w2844, index (row) #1=w2845, index (col) #1=0, index (row) #2=w2845, index (col) #2=1, index (row) #3=w2845, index (col) #3=2) -> (element #1=w2846:dbl, element #2=w2847:dbl, element #3=w2848:dbl)
                }
                frame 6 {
                  n376 = Index Array(array=w2852, index (row) #1=w2856, index (col) #1=0, index (row) #2=w2856, index (col) #2=1, index (row) #3=w2856, index (col) #3=2) -> (element #1=w2853:dbl, element #2=w2855:dbl, element #3=w2854:dbl)
                }
                frame 7 {
                  n377 = Index Array(array=w2860, index (row) #1=w2861, index (col) #1=0, index (row) #2=w2861, index (col) #2=1, index (row) #3=w2861, index (col) #3=2) -> (element #1=w2862:dbl, element #2=w2864:dbl, element #3=w2863:dbl)
                }
              }
            }
            frame "North east" {
              w2869 = 6
              n378 = case shown="2" w2869 {
                tunnel: [w2876 w2882 w2890 w2898 w2906 w2915 w2922 w2931] -> w2872
                tunnel: [w2878 w2884 w2892 w2899 w2908 w2917 w2924 w2933] -> w2871
                tunnel: [w2877 w2883 w2891 w2900 w2907 w2916 w2923 w2932] -> w2870
                tunnel: w2869 -> [w2880 w2885 w2893 w2901 w2909 w2914 w2925 w2930]
                tunnel: w2868 -> [w2873 w2881 w2889 w2897 w2905 w2913 w2921 w2929]
                frame 0, Default {
                  n379 = Index Array(array=w2873, index (row) #1=w2880, index (col) #1=0, index (row) #2=w2880, index (col) #2=1, index (row) #3=w2880, index (col) #3=2) -> (element #1=w2878:dbl, element #2=w2877:dbl, element #3=w2876:dbl)
                }
                frame 1 {
                  n380 = Index Array(array=w2881, index (row) #1=w2885, index (col) #1=0, index (row) #2=w2885, index (col) #2=1, index (row) #3=w2885, index (col) #3=2) -> (element #1=w2884:dbl, element #2=w2883:dbl, element #3=w2882:dbl)
                }
                frame 2 {
                  n381 = Index Array(array=w2889, index (row) #1=w2893, index (col) #1=0, index (row) #2=w2893, index (col) #2=1, index (row) #3=w2893, index (col) #3=2) -> (element #1=w2892:dbl, element #2=w2891:dbl, element #3=w2890:dbl)
                }
                frame 3 {
                  n382 = Index Array(array=w2897, index (row) #1=w2901, index (col) #1=0, index (row) #2=w2901, index (col) #2=1, index (row) #3=w2901, index (col) #3=2) -> (element #1=w2899:dbl, element #2=w2900:dbl, element #3=w2898:dbl)
                }
                frame 4 {
                  n383 = Index Array(array=w2905, index (row) #1=w2909, index (col) #1=0, index (row) #2=w2909, index (col) #2=1, index (row) #3=w2909, index (col) #3=2) -> (element #1=w2906:dbl, element #2=w2908:dbl, element #3=w2907:dbl)
                }
                frame 5 {
                  n384 = Index Array(array=w2913, index (row) #1=w2914, index (col) #1=0, index (row) #2=w2914, index (col) #2=1, index (row) #3=w2914, index (col) #3=2) -> (element #1=w2915:dbl, element #2=w2916:dbl, element #3=w2917:dbl)
                }
                frame 6 {
                  n385 = Index Array(array=w2921, index (row) #1=w2925, index (col) #1=0, index (row) #2=w2925, index (col) #2=1, index (row) #3=w2925, index (col) #3=2) -> (element #1=w2922:dbl, element #2=w2924:dbl, element #3=w2923:dbl)
                }
                frame 7 {
                  n386 = Index Array(array=w2929, index (row) #1=w2930, index (col) #1=0, index (row) #2=w2930, index (col) #2=1, index (row) #3=w2930, index (col) #3=2) -> (element #1=w2931:dbl, element #2=w2933:dbl, element #3=w2932:dbl)
                }
              }
            }
            frame "North west" {
              w2941 = 5
              n387 = case shown="2" w2941 {
                tunnel: [w2945 w2951 w2959 w2967 w2975 w2984 w2991 w3000] -> w2940
                tunnel: [w2947 w2953 w2961 w2968 w2977 w2986 w2993 w3002] -> w2939
                tunnel: [w2946 w2952 w2960 w2969 w2976 w2985 w2992 w3001] -> w2938
                tunnel: w2941 -> [w2949 w2954 w2962 w2970 w2978 w2983 w2994 w2999]
                tunnel: w2937 -> [w2942 w2950 w2958 w2966 w2974 w2982 w2990 w2998]
                frame 0, Default {
                  n388 = Index Array(array=w2942, index (row) #1=w2949, index (col) #1=0, index (row) #2=w2949, index (col) #2=1, index (row) #3=w2949, index (col) #3=2) -> (element #1=w2947:dbl, element #2=w2946:dbl, element #3=w2945:dbl)
                }
                frame 1 {
                  n389 = Index Array(array=w2950, index (row) #1=w2954, index (col) #1=0, index (row) #2=w2954, index (col) #2=1, index (row) #3=w2954, index (col) #3=2) -> (element #1=w2953:dbl, element #2=w2952:dbl, element #3=w2951:dbl)
                }
                frame 2 {
                  n390 = Index Array(array=w2958, index (row) #1=w2962, index (col) #1=0, index (row) #2=w2962, index (col) #2=1, index (row) #3=w2962, index (col) #3=2) -> (element #1=w2961:dbl, element #2=w2960:dbl, element #3=w2959:dbl)
                }
                frame 3 {
                  n391 = Index Array(array=w2966, index (row) #1=w2970, index (col) #1=0, index (row) #2=w2970, index (col) #2=1, index (row) #3=w2970, index (col) #3=2) -> (element #1=w2968:dbl, element #2=w2969:dbl, element #3=w2967:dbl)
                }
                frame 4 {
                  n392 = Index Array(array=w2974, index (row) #1=w2978, index (col) #1=0, index (row) #2=w2978, index (col) #2=1, index (row) #3=w2978, index (col) #3=2) -> (element #1=w2975:dbl, element #2=w2977:dbl, element #3=w2976:dbl)
                }
                frame 5 {
                  n393 = Index Array(array=w2982, index (row) #1=w2983, index (col) #1=0, index (row) #2=w2983, index (col) #2=1, index (row) #3=w2983, index (col) #3=2) -> (element #1=w2984:dbl, element #2=w2985:dbl, element #3=w2986:dbl)
                }
                frame 6 {
                  n394 = Index Array(array=w2990, index (row) #1=w2994, index (col) #1=0, index (row) #2=w2994, index (col) #2=1, index (row) #3=w2994, index (col) #3=2) -> (element #1=w2991:dbl, element #2=w2993:dbl, element #3=w2992:dbl)
                }
                frame 7 {
                  n395 = Index Array(array=w2998, index (row) #1=w2999, index (col) #1=0, index (row) #2=w2999, index (col) #2=1, index (row) #3=w2999, index (col) #3=2) -> (element #1=w3000:dbl, element #2=w3002:dbl, element #3=w3001:dbl)
                }
              }
            }
            frame "West" {
              w3010 = 3
              n396 = case shown="2" w3010 {
                tunnel: [w3014 w3020 w3028 w3036 w3044 w3053 w3060 w3069] -> w3007
                tunnel: [w3016 w3022 w3030 w3037 w3046 w3055 w3062 w3071] -> w3008
                tunnel: [w3015 w3021 w3029 w3038 w3045 w3054 w3061 w3070] -> w3006
                tunnel: w3010 -> [w3018 w3023 w3031 w3039 w3047 w3052 w3063 w3068]
                tunnel: w3009 -> [w3011 w3019 w3027 w3035 w3043 w3051 w3059 w3067]
                frame 0, Default {
                  n397 = Index Array(array=w3011, index (row) #1=w3018, index (col) #1=0, index (row) #2=w3018, index (col) #2=1, index (row) #3=w3018, index (col) #3=2) -> (element #1=w3016:dbl, element #2=w3015:dbl, element #3=w3014:dbl)
                }
                frame 1 {
                  n398 = Index Array(array=w3019, index (row) #1=w3023, index (col) #1=0, index (row) #2=w3023, index (col) #2=1, index (row) #3=w3023, index (col) #3=2) -> (element #1=w3022:dbl, element #2=w3021:dbl, element #3=w3020:dbl)
                }
                frame 2 {
                  n399 = Index Array(array=w3027, index (row) #1=w3031, index (col) #1=0, index (row) #2=w3031, index (col) #2=1, index (row) #3=w3031, index (col) #3=2) -> (element #1=w3030:dbl, element #2=w3029:dbl, element #3=w3028:dbl)
                }
                frame 3 {
                  n400 = Index Array(array=w3035, index (row) #1=w3039, index (col) #1=0, index (row) #2=w3039, index (col) #2=1, index (row) #3=w3039, index (col) #3=2) -> (element #1=w3037:dbl, element #2=w3038:dbl, element #3=w3036:dbl)
                }
                frame 4 {
                  n401 = Index Array(array=w3043, index (row) #1=w3047, index (col) #1=0, index (row) #2=w3047, index (col) #2=1, index (row) #3=w3047, index (col) #3=2) -> (element #1=w3044:dbl, element #2=w3046:dbl, element #3=w3045:dbl)
                }
                frame 5 {
                  n402 = Index Array(array=w3051, index (row) #1=w3052, index (col) #1=0, index (row) #2=w3052, index (col) #2=1, index (row) #3=w3052, index (col) #3=2) -> (element #1=w3053:dbl, element #2=w3054:dbl, element #3=w3055:dbl)
                }
                frame 6 {
                  n403 = Index Array(array=w3059, index (row) #1=w3063, index (col) #1=0, index (row) #2=w3063, index (col) #2=1, index (row) #3=w3063, index (col) #3=2) -> (element #1=w3060:dbl, element #2=w3062:dbl, element #3=w3061:dbl)
                }
                frame 7 {
                  n404 = Index Array(array=w3067, index (row) #1=w3068, index (col) #1=0, index (row) #2=w3068, index (col) #2=1, index (row) #3=w3068, index (col) #3=2) -> (element #1=w3069:dbl, element #2=w3071:dbl, element #3=w3070:dbl)
                }
              }
            }
            frame "East" {
              w3079 = 4
              n405 = case shown="2" w3079 {
                tunnel: [w3083 w3089 w3097 w3105 w3113 w3122 w3129 w3138] -> w3077
                tunnel: [w3085 w3091 w3099 w3106 w3115 w3124 w3131 w3140] -> w3076
                tunnel: [w3084 w3090 w3098 w3107 w3114 w3123 w3130 w3139] -> w3075
                tunnel: w3079 -> [w3087 w3092 w3100 w3108 w3116 w3121 w3132 w3137]
                tunnel: w3078 -> [w3080 w3088 w3096 w3104 w3112 w3120 w3128 w3136]
                frame 0, Default {
                  n406 = Index Array(array=w3080, index (row) #1=w3087, index (col) #1=0, index (row) #2=w3087, index (col) #2=1, index (row) #3=w3087, index (col) #3=2) -> (element #1=w3085:dbl, element #2=w3084:dbl, element #3=w3083:dbl)
                }
                frame 1 {
                  n407 = Index Array(array=w3088, index (row) #1=w3092, index (col) #1=0, index (row) #2=w3092, index (col) #2=1, index (row) #3=w3092, index (col) #3=2) -> (element #1=w3091:dbl, element #2=w3090:dbl, element #3=w3089:dbl)
                }
                frame 2 {
                  n408 = Index Array(array=w3096, index (row) #1=w3100, index (col) #1=0, index (row) #2=w3100, index (col) #2=1, index (row) #3=w3100, index (col) #3=2) -> (element #1=w3099:dbl, element #2=w3098:dbl, element #3=w3097:dbl)
                }
                frame 3 {
                  n409 = Index Array(array=w3104, index (row) #1=w3108, index (col) #1=0, index (row) #2=w3108, index (col) #2=1, index (row) #3=w3108, index (col) #3=2) -> (element #1=w3106:dbl, element #2=w3107:dbl, element #3=w3105:dbl)
                }
                frame 4 {
                  n410 = Index Array(array=w3112, index (row) #1=w3116, index (col) #1=0, index (row) #2=w3116, index (col) #2=1, index (row) #3=w3116, index (col) #3=2) -> (element #1=w3113:dbl, element #2=w3115:dbl, element #3=w3114:dbl)
                }
                frame 5 {
                  n411 = Index Array(array=w3120, index (row) #1=w3121, index (col) #1=0, index (row) #2=w3121, index (col) #2=1, index (row) #3=w3121, index (col) #3=2) -> (element #1=w3122:dbl, element #2=w3123:dbl, element #3=w3124:dbl)
                }
                frame 6 {
                  n412 = Index Array(array=w3128, index (row) #1=w3132, index (col) #1=0, index (row) #2=w3132, index (col) #2=1, index (row) #3=w3132, index (col) #3=2) -> (element #1=w3129:dbl, element #2=w3131:dbl, element #3=w3130:dbl)
                }
                frame 7 {
                  n413 = Index Array(array=w3136, index (row) #1=w3137, index (col) #1=0, index (row) #2=w3137, index (col) #2=1, index (row) #3=w3137, index (col) #3=2) -> (element #1=w3138:dbl, element #2=w3140:dbl, element #3=w3139:dbl)
                }
              }
            }
            frame "South" {
              w3148 = 0
              n414 = case shown="2" w3148 {
                tunnel: [w3152 w3158 w3166 w3174 w3182 w3191 w3198 w3207] -> w3147
                tunnel: [w3154 w3160 w3168 w3175 w3184 w3193 w3200 w3209] -> w3145
                tunnel: [w3153 w3159 w3167 w3176 w3183 w3192 w3199 w3208] -> w3144
                tunnel: w3148 -> [w3156 w3161 w3169 w3177 w3185 w3190 w3201 w3206]
                tunnel: w3146 -> [w3149 w3157 w3165 w3173 w3181 w3189 w3197 w3205]
                frame 0, Default {
                  n415 = Index Array(array=w3149, index (row) #1=w3156, index (col) #1=0, index (row) #2=w3156, index (col) #2=1, index (row) #3=w3156, index (col) #3=2) -> (element #1=w3154:dbl, element #2=w3153:dbl, element #3=w3152:dbl)
                }
                frame 1 {
                  n416 = Index Array(array=w3157, index (row) #1=w3161, index (col) #1=0, index (row) #2=w3161, index (col) #2=1, index (row) #3=w3161, index (col) #3=2) -> (element #1=w3160:dbl, element #2=w3159:dbl, element #3=w3158:dbl)
                }
                frame 2 {
                  n417 = Index Array(array=w3165, index (row) #1=w3169, index (col) #1=0, index (row) #2=w3169, index (col) #2=1, index (row) #3=w3169, index (col) #3=2) -> (element #1=w3168:dbl, element #2=w3167:dbl, element #3=w3166:dbl)
                }
                frame 3 {
                  n418 = Index Array(array=w3173, index (row) #1=w3177, index (col) #1=0, index (row) #2=w3177, index (col) #2=1, index (row) #3=w3177, index (col) #3=2) -> (element #1=w3175:dbl, element #2=w3176:dbl, element #3=w3174:dbl)
                }
                frame 4 {
                  n419 = Index Array(array=w3181, index (row) #1=w3185, index (col) #1=0, index (row) #2=w3185, index (col) #2=1, index (row) #3=w3185, index (col) #3=2) -> (element #1=w3182:dbl, element #2=w3184:dbl, element #3=w3183:dbl)
                }
                frame 5 {
                  n420 = Index Array(array=w3189, index (row) #1=w3190, index (col) #1=0, index (row) #2=w3190, index (col) #2=1, index (row) #3=w3190, index (col) #3=2) -> (element #1=w3191:dbl, element #2=w3192:dbl, element #3=w3193:dbl)
                }
                frame 6 {
                  n421 = Index Array(array=w3197, index (row) #1=w3201, index (col) #1=0, index (row) #2=w3201, index (col) #2=1, index (row) #3=w3201, index (col) #3=2) -> (element #1=w3198:dbl, element #2=w3200:dbl, element #3=w3199:dbl)
                }
                frame 7 {
                  n422 = Index Array(array=w3205, index (row) #1=w3206, index (col) #1=0, index (row) #2=w3206, index (col) #2=1, index (row) #3=w3206, index (col) #3=2) -> (element #1=w3207:dbl, element #2=w3209:dbl, element #3=w3208:dbl)
                }
              }
            }
            frame "South west" {
              w3217 = 1
              n423 = case shown="2" w3217 {
                tunnel: [w3221 w3227 w3235 w3243 w3251 w3260 w3267 w3276] -> w3215
                tunnel: [w3223 w3229 w3237 w3244 w3253 w3262 w3269 w3278] -> w3214
                tunnel: [w3222 w3228 w3236 w3245 w3252 w3261 w3268 w3277] -> w3213
                tunnel: w3217 -> [w3225 w3230 w3238 w3246 w3254 w3259 w3270 w3275]
                tunnel: w3216 -> [w3218 w3226 w3234 w3242 w3250 w3258 w3266 w3274]
                frame 0, Default {
                  n424 = Index Array(array=w3218, index (row) #1=w3225, index (col) #1=0, index (row) #2=w3225, index (col) #2=1, index (row) #3=w3225, index (col) #3=2) -> (element #1=w3223:dbl, element #2=w3222:dbl, element #3=w3221:dbl)
                }
                frame 1 {
                  n425 = Index Array(array=w3226, index (row) #1=w3230, index (col) #1=0, index (row) #2=w3230, index (col) #2=1, index (row) #3=w3230, index (col) #3=2) -> (element #1=w3229:dbl, element #2=w3228:dbl, element #3=w3227:dbl)
                }
                frame 2 {
                  n426 = Index Array(array=w3234, index (row) #1=w3238, index (col) #1=0, index (row) #2=w3238, index (col) #2=1, index (row) #3=w3238, index (col) #3=2) -> (element #1=w3237:dbl, element #2=w3236:dbl, element #3=w3235:dbl)
                }
                frame 3 {
                  n427 = Index Array(array=w3242, index (row) #1=w3246, index (col) #1=0, index (row) #2=w3246, index (col) #2=1, index (row) #3=w3246, index (col) #3=2) -> (element #1=w3244:dbl, element #2=w3245:dbl, element #3=w3243:dbl)
                }
                frame 4 {
                  n428 = Index Array(array=w3250, index (row) #1=w3254, index (col) #1=0, index (row) #2=w3254, index (col) #2=1, index (row) #3=w3254, index (col) #3=2) -> (element #1=w3251:dbl, element #2=w3253:dbl, element #3=w3252:dbl)
                }
                frame 5 {
                  n429 = Index Array(array=w3258, index (row) #1=w3259, index (col) #1=0, index (row) #2=w3259, index (col) #2=1, index (row) #3=w3259, index (col) #3=2) -> (element #1=w3260:dbl, element #2=w3261:dbl, element #3=w3262:dbl)
                }
                frame 6 {
                  n430 = Index Array(array=w3266, index (row) #1=w3270, index (col) #1=0, index (row) #2=w3270, index (col) #2=1, index (row) #3=w3270, index (col) #3=2) -> (element #1=w3267:dbl, element #2=w3269:dbl, element #3=w3268:dbl)
                }
                frame 7 {
                  n431 = Index Array(array=w3274, index (row) #1=w3275, index (col) #1=0, index (row) #2=w3275, index (col) #2=1, index (row) #3=w3275, index (col) #3=2) -> (element #1=w3276:dbl, element #2=w3278:dbl, element #3=w3277:dbl)
                }
              }
            }
            frame "South east" {
              w3286 = 2
              n432 = case shown="2" w3286 {
                tunnel: [w3290 w3296 w3304 w3312 w3320 w3329 w3336 w3345] -> w3285
                tunnel: [w3292 w3298 w3306 w3313 w3322 w3331 w3338 w3347] -> w3284
                tunnel: [w3291 w3297 w3305 w3314 w3321 w3330 w3337 w3346] -> w3283
                tunnel: w3286 -> [w3294 w3299 w3307 w3315 w3323 w3328 w3339 w3344]
                tunnel: w3282 -> [w3287 w3295 w3303 w3311 w3319 w3327 w3335 w3343]
                frame 0, Default {
                  n433 = Index Array(array=w3287, index (row) #1=w3294, index (col) #1=0, index (row) #2=w3294, index (col) #2=1, index (row) #3=w3294, index (col) #3=2) -> (element #1=w3292:dbl, element #2=w3291:dbl, element #3=w3290:dbl)
                }
                frame 1 {
                  n434 = Index Array(array=w3295, index (row) #1=w3299, index (col) #1=0, index (row) #2=w3299, index (col) #2=1, index (row) #3=w3299, index (col) #3=2) -> (element #1=w3298:dbl, element #2=w3297:dbl, element #3=w3296:dbl)
                }
                frame 2 {
                  n435 = Index Array(array=w3303, index (row) #1=w3307, index (col) #1=0, index (row) #2=w3307, index (col) #2=1, index (row) #3=w3307, index (col) #3=2) -> (element #1=w3306:dbl, element #2=w3305:dbl, element #3=w3304:dbl)
                }
                frame 3 {
                  n436 = Index Array(array=w3311, index (row) #1=w3315, index (col) #1=0, index (row) #2=w3315, index (col) #2=1, index (row) #3=w3315, index (col) #3=2) -> (element #1=w3313:dbl, element #2=w3314:dbl, element #3=w3312:dbl)
                }
                frame 4 {
                  n437 = Index Array(array=w3319, index (row) #1=w3323, index (col) #1=0, index (row) #2=w3323, index (col) #2=1, index (row) #3=w3323, index (col) #3=2) -> (element #1=w3320:dbl, element #2=w3322:dbl, element #3=w3321:dbl)
                }
                frame 5 {
                  n438 = Index Array(array=w3327, index (row) #1=w3328, index (col) #1=0, index (row) #2=w3328, index (col) #2=1, index (row) #3=w3328, index (col) #3=2) -> (element #1=w3329:dbl, element #2=w3330:dbl, element #3=w3331:dbl)
                }
                frame 6 {
                  n439 = Index Array(array=w3335, index (row) #1=w3339, index (col) #1=0, index (row) #2=w3339, index (col) #2=1, index (row) #3=w3339, index (col) #3=2) -> (element #1=w3336:dbl, element #2=w3338:dbl, element #3=w3337:dbl)
                }
                frame 7 {
                  n440 = Index Array(array=w3343, index (row) #1=w3344, index (col) #1=0, index (row) #2=w3344, index (col) #2=1, index (row) #3=w3344, index (col) #3=2) -> (element #1=w3345:dbl, element #2=w3347:dbl, element #3=w3346:dbl)
                }
              }
            }
          }
        }
        frame "South west" {
          n441 = case shown="\"North\", Default" w3354 {
            tunnel: [w3359 w3429 w3497 w3564 w3634 w3704 w3772 w3842] -> w3353
            tunnel: [w3358 w3428 w3496 w3565 w3633 w3702 w3771 w3841] -> w3352
            tunnel: [w3357 w3427 w3495 w3563 w3632 w3701 w3770 w3840] -> w3351
            tunnel: w3355 -> [w3356 w3425 w3494 w3566 w3635 w3703 w3773 w3839]
            frame "North", Default {
              w3360 = 6
              n442 = case shown="2" w3360 {
                tunnel: [w3364 w3370 w3378 w3386 w3394 w3403 w3410 w3419] -> w3359
                tunnel: [w3366 w3372 w3380 w3387 w3396 w3405 w3412 w3421] -> w3358
                tunnel: [w3365 w3371 w3379 w3388 w3395 w3404 w3411 w3420] -> w3357
                tunnel: w3360 -> [w3368 w3373 w3381 w3389 w3397 w3402 w3413 w3418]
                tunnel: w3356 -> [w3361 w3369 w3377 w3385 w3393 w3401 w3409 w3417]
                frame 0, Default {
                  n443 = Index Array(array=w3361, index (row) #1=w3368, index (col) #1=0, index (row) #2=w3368, index (col) #2=1, index (row) #3=w3368, index (col) #3=2) -> (element #1=w3366:dbl, element #2=w3365:dbl, element #3=w3364:dbl)
                }
                frame 1 {
                  n444 = Index Array(array=w3369, index (row) #1=w3373, index (col) #1=0, index (row) #2=w3373, index (col) #2=1, index (row) #3=w3373, index (col) #3=2) -> (element #1=w3372:dbl, element #2=w3371:dbl, element #3=w3370:dbl)
                }
                frame 2 {
                  n445 = Index Array(array=w3377, index (row) #1=w3381, index (col) #1=0, index (row) #2=w3381, index (col) #2=1, index (row) #3=w3381, index (col) #3=2) -> (element #1=w3380:dbl, element #2=w3379:dbl, element #3=w3378:dbl)
                }
                frame 3 {
                  n446 = Index Array(array=w3385, index (row) #1=w3389, index (col) #1=0, index (row) #2=w3389, index (col) #2=1, index (row) #3=w3389, index (col) #3=2) -> (element #1=w3387:dbl, element #2=w3388:dbl, element #3=w3386:dbl)
                }
                frame 4 {
                  n447 = Index Array(array=w3393, index (row) #1=w3397, index (col) #1=0, index (row) #2=w3397, index (col) #2=1, index (row) #3=w3397, index (col) #3=2) -> (element #1=w3394:dbl, element #2=w3396:dbl, element #3=w3395:dbl)
                }
                frame 5 {
                  n448 = Index Array(array=w3401, index (row) #1=w3402, index (col) #1=0, index (row) #2=w3402, index (col) #2=1, index (row) #3=w3402, index (col) #3=2) -> (element #1=w3403:dbl, element #2=w3404:dbl, element #3=w3405:dbl)
                }
                frame 6 {
                  n449 = Index Array(array=w3409, index (row) #1=w3413, index (col) #1=0, index (row) #2=w3413, index (col) #2=1, index (row) #3=w3413, index (col) #3=2) -> (element #1=w3410:dbl, element #2=w3412:dbl, element #3=w3411:dbl)
                }
                frame 7 {
                  n450 = Index Array(array=w3417, index (row) #1=w3418, index (col) #1=0, index (row) #2=w3418, index (col) #2=1, index (row) #3=w3418, index (col) #3=2) -> (element #1=w3419:dbl, element #2=w3421:dbl, element #3=w3420:dbl)
                }
              }
            }
            frame "North east" {
              w3426 = 7
              n451 = case shown="2" w3426 {
                tunnel: [w3433 w3439 w3447 w3455 w3463 w3472 w3479 w3488] -> w3429
                tunnel: [w3435 w3441 w3449 w3456 w3465 w3474 w3481 w3490] -> w3428
                tunnel: [w3434 w3440 w3448 w3457 w3464 w3473 w3480 w3489] -> w3427
                tunnel: w3426 -> [w3437 w3442 w3450 w3458 w3466 w3471 w3482 w3487]
                tunnel: w3425 -> [w3430 w3438 w3446 w3454 w3462 w3470 w3478 w3486]
                frame 0, Default {
                  n452 = Index Array(array=w3430, index (row) #1=w3437, index (col) #1=0, index (row) #2=w3437, index (col) #2=1, index (row) #3=w3437, index (col) #3=2) -> (element #1=w3435:dbl, element #2=w3434:dbl, element #3=w3433:dbl)
                }
                frame 1 {
                  n453 = Index Array(array=w3438, index (row) #1=w3442, index (col) #1=0, index (row) #2=w3442, index (col) #2=1, index (row) #3=w3442, index (col) #3=2) -> (element #1=w3441:dbl, element #2=w3440:dbl, element #3=w3439:dbl)
                }
                frame 2 {
                  n454 = Index Array(array=w3446, index (row) #1=w3450, index (col) #1=0, index (row) #2=w3450, index (col) #2=1, index (row) #3=w3450, index (col) #3=2) -> (element #1=w3449:dbl, element #2=w3448:dbl, element #3=w3447:dbl)
                }
                frame 3 {
                  n455 = Index Array(array=w3454, index (row) #1=w3458, index (col) #1=0, index (row) #2=w3458, index (col) #2=1, index (row) #3=w3458, index (col) #3=2) -> (element #1=w3456:dbl, element #2=w3457:dbl, element #3=w3455:dbl)
                }
                frame 4 {
                  n456 = Index Array(array=w3462, index (row) #1=w3466, index (col) #1=0, index (row) #2=w3466, index (col) #2=1, index (row) #3=w3466, index (col) #3=2) -> (element #1=w3463:dbl, element #2=w3465:dbl, element #3=w3464:dbl)
                }
                frame 5 {
                  n457 = Index Array(array=w3470, index (row) #1=w3471, index (col) #1=0, index (row) #2=w3471, index (col) #2=1, index (row) #3=w3471, index (col) #3=2) -> (element #1=w3472:dbl, element #2=w3473:dbl, element #3=w3474:dbl)
                }
                frame 6 {
                  n458 = Index Array(array=w3478, index (row) #1=w3482, index (col) #1=0, index (row) #2=w3482, index (col) #2=1, index (row) #3=w3482, index (col) #3=2) -> (element #1=w3479:dbl, element #2=w3481:dbl, element #3=w3480:dbl)
                }
                frame 7 {
                  n459 = Index Array(array=w3486, index (row) #1=w3487, index (col) #1=0, index (row) #2=w3487, index (col) #2=1, index (row) #3=w3487, index (col) #3=2) -> (element #1=w3488:dbl, element #2=w3490:dbl, element #3=w3489:dbl)
                }
              }
            }
            frame "North west" {
              w3498 = 4
              n460 = case shown="2" w3498 {
                tunnel: [w3502 w3508 w3516 w3524 w3532 w3541 w3548 w3557] -> w3497
                tunnel: [w3504 w3510 w3518 w3525 w3534 w3543 w3550 w3559] -> w3496
                tunnel: [w3503 w3509 w3517 w3526 w3533 w3542 w3549 w3558] -> w3495
                tunnel: w3498 -> [w3506 w3511 w3519 w3527 w3535 w3540 w3551 w3556]
                tunnel: w3494 -> [w3499 w3507 w3515 w3523 w3531 w3539 w3547 w3555]
                frame 0, Default {
                  n461 = Index Array(array=w3499, index (row) #1=w3506, index (col) #1=0, index (row) #2=w3506, index (col) #2=1, index (row) #3=w3506, index (col) #3=2) -> (element #1=w3504:dbl, element #2=w3503:dbl, element #3=w3502:dbl)
                }
                frame 1 {
                  n462 = Index Array(array=w3507, index (row) #1=w3511, index (col) #1=0, index (row) #2=w3511, index (col) #2=1, index (row) #3=w3511, index (col) #3=2) -> (element #1=w3510:dbl, element #2=w3509:dbl, element #3=w3508:dbl)
                }
                frame 2 {
                  n463 = Index Array(array=w3515, index (row) #1=w3519, index (col) #1=0, index (row) #2=w3519, index (col) #2=1, index (row) #3=w3519, index (col) #3=2) -> (element #1=w3518:dbl, element #2=w3517:dbl, element #3=w3516:dbl)
                }
                frame 3 {
                  n464 = Index Array(array=w3523, index (row) #1=w3527, index (col) #1=0, index (row) #2=w3527, index (col) #2=1, index (row) #3=w3527, index (col) #3=2) -> (element #1=w3525:dbl, element #2=w3526:dbl, element #3=w3524:dbl)
                }
                frame 4 {
                  n465 = Index Array(array=w3531, index (row) #1=w3535, index (col) #1=0, index (row) #2=w3535, index (col) #2=1, index (row) #3=w3535, index (col) #3=2) -> (element #1=w3532:dbl, element #2=w3534:dbl, element #3=w3533:dbl)
                }
                frame 5 {
                  n466 = Index Array(array=w3539, index (row) #1=w3540, index (col) #1=0, index (row) #2=w3540, index (col) #2=1, index (row) #3=w3540, index (col) #3=2) -> (element #1=w3541:dbl, element #2=w3542:dbl, element #3=w3543:dbl)
                }
                frame 6 {
                  n467 = Index Array(array=w3547, index (row) #1=w3551, index (col) #1=0, index (row) #2=w3551, index (col) #2=1, index (row) #3=w3551, index (col) #3=2) -> (element #1=w3548:dbl, element #2=w3550:dbl, element #3=w3549:dbl)
                }
                frame 7 {
                  n468 = Index Array(array=w3555, index (row) #1=w3556, index (col) #1=0, index (row) #2=w3556, index (col) #2=1, index (row) #3=w3556, index (col) #3=2) -> (element #1=w3557:dbl, element #2=w3559:dbl, element #3=w3558:dbl)
                }
              }
            }
            frame "West" {
              w3567 = 2
              n469 = case shown="2" w3567 {
                tunnel: [w3571 w3577 w3585 w3593 w3601 w3610 w3617 w3626] -> w3564
                tunnel: [w3573 w3579 w3587 w3594 w3603 w3612 w3619 w3628] -> w3565
                tunnel: [w3572 w3578 w3586 w3595 w3602 w3611 w3618 w3627] -> w3563
                tunnel: w3567 -> [w3575 w3580 w3588 w3596 w3604 w3609 w3620 w3625]
                tunnel: w3566 -> [w3568 w3576 w3584 w3592 w3600 w3608 w3616 w3624]
                frame 0, Default {
                  n470 = Index Array(array=w3568, index (row) #1=w3575, index (col) #1=0, index (row) #2=w3575, index (col) #2=1, index (row) #3=w3575, index (col) #3=2) -> (element #1=w3573:dbl, element #2=w3572:dbl, element #3=w3571:dbl)
                }
                frame 1 {
                  n471 = Index Array(array=w3576, index (row) #1=w3580, index (col) #1=0, index (row) #2=w3580, index (col) #2=1, index (row) #3=w3580, index (col) #3=2) -> (element #1=w3579:dbl, element #2=w3578:dbl, element #3=w3577:dbl)
                }
                frame 2 {
                  n472 = Index Array(array=w3584, index (row) #1=w3588, index (col) #1=0, index (row) #2=w3588, index (col) #2=1, index (row) #3=w3588, index (col) #3=2) -> (element #1=w3587:dbl, element #2=w3586:dbl, element #3=w3585:dbl)
                }
                frame 3 {
                  n473 = Index Array(array=w3592, index (row) #1=w3596, index (col) #1=0, index (row) #2=w3596, index (col) #2=1, index (row) #3=w3596, index (col) #3=2) -> (element #1=w3594:dbl, element #2=w3595:dbl, element #3=w3593:dbl)
                }
                frame 4 {
                  n474 = Index Array(array=w3600, index (row) #1=w3604, index (col) #1=0, index (row) #2=w3604, index (col) #2=1, index (row) #3=w3604, index (col) #3=2) -> (element #1=w3601:dbl, element #2=w3603:dbl, element #3=w3602:dbl)
                }
                frame 5 {
                  n475 = Index Array(array=w3608, index (row) #1=w3609, index (col) #1=0, index (row) #2=w3609, index (col) #2=1, index (row) #3=w3609, index (col) #3=2) -> (element #1=w3610:dbl, element #2=w3611:dbl, element #3=w3612:dbl)
                }
                frame 6 {
                  n476 = Index Array(array=w3616, index (row) #1=w3620, index (col) #1=0, index (row) #2=w3620, index (col) #2=1, index (row) #3=w3620, index (col) #3=2) -> (element #1=w3617:dbl, element #2=w3619:dbl, element #3=w3618:dbl)
                }
                frame 7 {
                  n477 = Index Array(array=w3624, index (row) #1=w3625, index (col) #1=0, index (row) #2=w3625, index (col) #2=1, index (row) #3=w3625, index (col) #3=2) -> (element #1=w3626:dbl, element #2=w3628:dbl, element #3=w3627:dbl)
                }
              }
            }
            frame "East" {
              w3636 = 5
              n478 = case shown="2" w3636 {
                tunnel: [w3640 w3646 w3654 w3662 w3670 w3679 w3686 w3695] -> w3634
                tunnel: [w3642 w3648 w3656 w3663 w3672 w3681 w3688 w3697] -> w3633
                tunnel: [w3641 w3647 w3655 w3664 w3671 w3680 w3687 w3696] -> w3632
                tunnel: w3636 -> [w3644 w3649 w3657 w3665 w3673 w3678 w3689 w3694]
                tunnel: w3635 -> [w3637 w3645 w3653 w3661 w3669 w3677 w3685 w3693]
                frame 0, Default {
                  n479 = Index Array(array=w3637, index (row) #1=w3644, index (col) #1=0, index (row) #2=w3644, index (col) #2=1, index (row) #3=w3644, index (col) #3=2) -> (element #1=w3642:dbl, element #2=w3641:dbl, element #3=w3640:dbl)
                }
                frame 1 {
                  n480 = Index Array(array=w3645, index (row) #1=w3649, index (col) #1=0, index (row) #2=w3649, index (col) #2=1, index (row) #3=w3649, index (col) #3=2) -> (element #1=w3648:dbl, element #2=w3647:dbl, element #3=w3646:dbl)
                }
                frame 2 {
                  n481 = Index Array(array=w3653, index (row) #1=w3657, index (col) #1=0, index (row) #2=w3657, index (col) #2=1, index (row) #3=w3657, index (col) #3=2) -> (element #1=w3656:dbl, element #2=w3655:dbl, element #3=w3654:dbl)
                }
                frame 3 {
                  n482 = Index Array(array=w3661, index (row) #1=w3665, index (col) #1=0, index (row) #2=w3665, index (col) #2=1, index (row) #3=w3665, index (col) #3=2) -> (element #1=w3663:dbl, element #2=w3664:dbl, element #3=w3662:dbl)
                }
                frame 4 {
                  n483 = Index Array(array=w3669, index (row) #1=w3673, index (col) #1=0, index (row) #2=w3673, index (col) #2=1, index (row) #3=w3673, index (col) #3=2) -> (element #1=w3670:dbl, element #2=w3672:dbl, element #3=w3671:dbl)
                }
                frame 5 {
                  n484 = Index Array(array=w3677, index (row) #1=w3678, index (col) #1=0, index (row) #2=w3678, index (col) #2=1, index (row) #3=w3678, index (col) #3=2) -> (element #1=w3679:dbl, element #2=w3680:dbl, element #3=w3681:dbl)
                }
                frame 6 {
                  n485 = Index Array(array=w3685, index (row) #1=w3689, index (col) #1=0, index (row) #2=w3689, index (col) #2=1, index (row) #3=w3689, index (col) #3=2) -> (element #1=w3686:dbl, element #2=w3688:dbl, element #3=w3687:dbl)
                }
                frame 7 {
                  n486 = Index Array(array=w3693, index (row) #1=w3694, index (col) #1=0, index (row) #2=w3694, index (col) #2=1, index (row) #3=w3694, index (col) #3=2) -> (element #1=w3695:dbl, element #2=w3697:dbl, element #3=w3696:dbl)
                }
              }
            }
            frame "South" {
              w3705 = 1
              n487 = case shown="2" w3705 {
                tunnel: [w3709 w3715 w3723 w3731 w3739 w3748 w3755 w3764] -> w3704
                tunnel: [w3711 w3717 w3725 w3732 w3741 w3750 w3757 w3766] -> w3702
                tunnel: [w3710 w3716 w3724 w3733 w3740 w3749 w3756 w3765] -> w3701
                tunnel: w3705 -> [w3713 w3718 w3726 w3734 w3742 w3747 w3758 w3763]
                tunnel: w3703 -> [w3706 w3714 w3722 w3730 w3738 w3746 w3754 w3762]
                frame 0, Default {
                  n488 = Index Array(array=w3706, index (row) #1=w3713, index (col) #1=0, index (row) #2=w3713, index (col) #2=1, index (row) #3=w3713, index (col) #3=2) -> (element #1=w3711:dbl, element #2=w3710:dbl, element #3=w3709:dbl)
                }
                frame 1 {
                  n489 = Index Array(array=w3714, index (row) #1=w3718, index (col) #1=0, index (row) #2=w3718, index (col) #2=1, index (row) #3=w3718, index (col) #3=2) -> (element #1=w3717:dbl, element #2=w3716:dbl, element #3=w3715:dbl)
                }
                frame 2 {
                  n490 = Index Array(array=w3722, index (row) #1=w3726, index (col) #1=0, index (row) #2=w3726, index (col) #2=1, index (row) #3=w3726, index (col) #3=2) -> (element #1=w3725:dbl, element #2=w3724:dbl, element #3=w3723:dbl)
                }
                frame 3 {
                  n491 = Index Array(array=w3730, index (row) #1=w3734, index (col) #1=0, index (row) #2=w3734, index (col) #2=1, index (row) #3=w3734, index (col) #3=2) -> (element #1=w3732:dbl, element #2=w3733:dbl, element #3=w3731:dbl)
                }
                frame 4 {
                  n492 = Index Array(array=w3738, index (row) #1=w3742, index (col) #1=0, index (row) #2=w3742, index (col) #2=1, index (row) #3=w3742, index (col) #3=2) -> (element #1=w3739:dbl, element #2=w3741:dbl, element #3=w3740:dbl)
                }
                frame 5 {
                  n493 = Index Array(array=w3746, index (row) #1=w3747, index (col) #1=0, index (row) #2=w3747, index (col) #2=1, index (row) #3=w3747, index (col) #3=2) -> (element #1=w3748:dbl, element #2=w3749:dbl, element #3=w3750:dbl)
                }
                frame 6 {
                  n494 = Index Array(array=w3754, index (row) #1=w3758, index (col) #1=0, index (row) #2=w3758, index (col) #2=1, index (row) #3=w3758, index (col) #3=2) -> (element #1=w3755:dbl, element #2=w3757:dbl, element #3=w3756:dbl)
                }
                frame 7 {
                  n495 = Index Array(array=w3762, index (row) #1=w3763, index (col) #1=0, index (row) #2=w3763, index (col) #2=1, index (row) #3=w3763, index (col) #3=2) -> (element #1=w3764:dbl, element #2=w3766:dbl, element #3=w3765:dbl)
                }
              }
            }
            frame "South west" {
              w3774 = 0
              n496 = case shown="2" w3774 {
                tunnel: [w3778 w3784 w3792 w3800 w3808 w3817 w3824 w3833] -> w3772
                tunnel: [w3780 w3786 w3794 w3801 w3810 w3819 w3826 w3835] -> w3771
                tunnel: [w3779 w3785 w3793 w3802 w3809 w3818 w3825 w3834] -> w3770
                tunnel: w3774 -> [w3782 w3787 w3795 w3803 w3811 w3816 w3827 w3832]
                tunnel: w3773 -> [w3775 w3783 w3791 w3799 w3807 w3815 w3823 w3831]
                frame 0, Default {
                  n497 = Index Array(array=w3775, index (row) #1=w3782, index (col) #1=0, index (row) #2=w3782, index (col) #2=1, index (row) #3=w3782, index (col) #3=2) -> (element #1=w3780:dbl, element #2=w3779:dbl, element #3=w3778:dbl)
                }
                frame 1 {
                  n498 = Index Array(array=w3783, index (row) #1=w3787, index (col) #1=0, index (row) #2=w3787, index (col) #2=1, index (row) #3=w3787, index (col) #3=2) -> (element #1=w3786:dbl, element #2=w3785:dbl, element #3=w3784:dbl)
                }
                frame 2 {
                  n499 = Index Array(array=w3791, index (row) #1=w3795, index (col) #1=0, index (row) #2=w3795, index (col) #2=1, index (row) #3=w3795, index (col) #3=2) -> (element #1=w3794:dbl, element #2=w3793:dbl, element #3=w3792:dbl)
                }
                frame 3 {
                  n500 = Index Array(array=w3799, index (row) #1=w3803, index (col) #1=0, index (row) #2=w3803, index (col) #2=1, index (row) #3=w3803, index (col) #3=2) -> (element #1=w3801:dbl, element #2=w3802:dbl, element #3=w3800:dbl)
                }
                frame 4 {
                  n501 = Index Array(array=w3807, index (row) #1=w3811, index (col) #1=0, index (row) #2=w3811, index (col) #2=1, index (row) #3=w3811, index (col) #3=2) -> (element #1=w3808:dbl, element #2=w3810:dbl, element #3=w3809:dbl)
                }
                frame 5 {
                  n502 = Index Array(array=w3815, index (row) #1=w3816, index (col) #1=0, index (row) #2=w3816, index (col) #2=1, index (row) #3=w3816, index (col) #3=2) -> (element #1=w3817:dbl, element #2=w3818:dbl, element #3=w3819:dbl)
                }
                frame 6 {
                  n503 = Index Array(array=w3823, index (row) #1=w3827, index (col) #1=0, index (row) #2=w3827, index (col) #2=1, index (row) #3=w3827, index (col) #3=2) -> (element #1=w3824:dbl, element #2=w3826:dbl, element #3=w3825:dbl)
                }
                frame 7 {
                  n504 = Index Array(array=w3831, index (row) #1=w3832, index (col) #1=0, index (row) #2=w3832, index (col) #2=1, index (row) #3=w3832, index (col) #3=2) -> (element #1=w3833:dbl, element #2=w3835:dbl, element #3=w3834:dbl)
                }
              }
            }
            frame "South east" {
              w3843 = 3
              n505 = case shown="2" w3843 {
                tunnel: [w3847 w3853 w3861 w3869 w3877 w3886 w3893 w3902] -> w3842
                tunnel: [w3849 w3855 w3863 w3870 w3879 w3888 w3895 w3904] -> w3841
                tunnel: [w3848 w3854 w3862 w3871 w3878 w3887 w3894 w3903] -> w3840
                tunnel: w3843 -> [w3851 w3856 w3864 w3872 w3880 w3885 w3896 w3901]
                tunnel: w3839 -> [w3844 w3852 w3860 w3868 w3876 w3884 w3892 w3900]
                frame 0, Default {
                  n506 = Index Array(array=w3844, index (row) #1=w3851, index (col) #1=0, index (row) #2=w3851, index (col) #2=1, index (row) #3=w3851, index (col) #3=2) -> (element #1=w3849:dbl, element #2=w3848:dbl, element #3=w3847:dbl)
                }
                frame 1 {
                  n507 = Index Array(array=w3852, index (row) #1=w3856, index (col) #1=0, index (row) #2=w3856, index (col) #2=1, index (row) #3=w3856, index (col) #3=2) -> (element #1=w3855:dbl, element #2=w3854:dbl, element #3=w3853:dbl)
                }
                frame 2 {
                  n508 = Index Array(array=w3860, index (row) #1=w3864, index (col) #1=0, index (row) #2=w3864, index (col) #2=1, index (row) #3=w3864, index (col) #3=2) -> (element #1=w3863:dbl, element #2=w3862:dbl, element #3=w3861:dbl)
                }
                frame 3 {
                  n509 = Index Array(array=w3868, index (row) #1=w3872, index (col) #1=0, index (row) #2=w3872, index (col) #2=1, index (row) #3=w3872, index (col) #3=2) -> (element #1=w3870:dbl, element #2=w3871:dbl, element #3=w3869:dbl)
                }
                frame 4 {
                  n510 = Index Array(array=w3876, index (row) #1=w3880, index (col) #1=0, index (row) #2=w3880, index (col) #2=1, index (row) #3=w3880, index (col) #3=2) -> (element #1=w3877:dbl, element #2=w3879:dbl, element #3=w3878:dbl)
                }
                frame 5 {
                  n511 = Index Array(array=w3884, index (row) #1=w3885, index (col) #1=0, index (row) #2=w3885, index (col) #2=1, index (row) #3=w3885, index (col) #3=2) -> (element #1=w3886:dbl, element #2=w3887:dbl, element #3=w3888:dbl)
                }
                frame 6 {
                  n512 = Index Array(array=w3892, index (row) #1=w3896, index (col) #1=0, index (row) #2=w3896, index (col) #2=1, index (row) #3=w3896, index (col) #3=2) -> (element #1=w3893:dbl, element #2=w3895:dbl, element #3=w3894:dbl)
                }
                frame 7 {
                  n513 = Index Array(array=w3900, index (row) #1=w3901, index (col) #1=0, index (row) #2=w3901, index (col) #2=1, index (row) #3=w3901, index (col) #3=2) -> (element #1=w3902:dbl, element #2=w3904:dbl, element #3=w3903:dbl)
                }
              }
            }
          }
        }
        frame "South east" {
          n514 = case shown="\"North\", Default" w3911 {
            tunnel: [w3916 w3986 w4054 w4121 w4191 w4261 w4329 w4399] -> w3910
            tunnel: [w3915 w3985 w4053 w4122 w4190 w4259 w4328 w4398] -> w3909
            tunnel: [w3914 w3984 w4052 w4120 w4189 w4258 w4327 w4397] -> w3908
            tunnel: w3912 -> [w3913 w3982 w4051 w4123 w4192 w4260 w4330 w4396]
            frame "North", Default {
              w3917 = 5
              n515 = case shown="2" w3917 {
                tunnel: [w3921 w3927 w3935 w3943 w3951 w3960 w3967 w3976] -> w3916
                tunnel: [w3923 w3929 w3937 w3944 w3953 w3962 w3969 w3978] -> w3915
                tunnel: [w3922 w3928 w3936 w3945 w3952 w3961 w3968 w3977] -> w3914
                tunnel: w3917 -> [w3925 w3930 w3938 w3946 w3954 w3959 w3970 w3975]
                tunnel: w3913 -> [w3918 w3926 w3934 w3942 w3950 w3958 w3966 w3974]
                frame 0, Default {
                  n516 = Index Array(array=w3918, index (row) #1=w3925, index (col) #1=0, index (row) #2=w3925, index (col) #2=1, index (row) #3=w3925, index (col) #3=2) -> (element #1=w3923:dbl, element #2=w3922:dbl, element #3=w3921:dbl)
                }
                frame 1 {
                  n517 = Index Array(array=w3926, index (row) #1=w3930, index (col) #1=0, index (row) #2=w3930, index (col) #2=1, index (row) #3=w3930, index (col) #3=2) -> (element #1=w3929:dbl, element #2=w3928:dbl, element #3=w3927:dbl)
                }
                frame 2 {
                  n518 = Index Array(array=w3934, index (row) #1=w3938, index (col) #1=0, index (row) #2=w3938, index (col) #2=1, index (row) #3=w3938, index (col) #3=2) -> (element #1=w3937:dbl, element #2=w3936:dbl, element #3=w3935:dbl)
                }
                frame 3 {
                  n519 = Index Array(array=w3942, index (row) #1=w3946, index (col) #1=0, index (row) #2=w3946, index (col) #2=1, index (row) #3=w3946, index (col) #3=2) -> (element #1=w3944:dbl, element #2=w3945:dbl, element #3=w3943:dbl)
                }
                frame 4 {
                  n520 = Index Array(array=w3950, index (row) #1=w3954, index (col) #1=0, index (row) #2=w3954, index (col) #2=1, index (row) #3=w3954, index (col) #3=2) -> (element #1=w3951:dbl, element #2=w3953:dbl, element #3=w3952:dbl)
                }
                frame 5 {
                  n521 = Index Array(array=w3958, index (row) #1=w3959, index (col) #1=0, index (row) #2=w3959, index (col) #2=1, index (row) #3=w3959, index (col) #3=2) -> (element #1=w3960:dbl, element #2=w3961:dbl, element #3=w3962:dbl)
                }
                frame 6 {
                  n522 = Index Array(array=w3966, index (row) #1=w3970, index (col) #1=0, index (row) #2=w3970, index (col) #2=1, index (row) #3=w3970, index (col) #3=2) -> (element #1=w3967:dbl, element #2=w3969:dbl, element #3=w3968:dbl)
                }
                frame 7 {
                  n523 = Index Array(array=w3974, index (row) #1=w3975, index (col) #1=0, index (row) #2=w3975, index (col) #2=1, index (row) #3=w3975, index (col) #3=2) -> (element #1=w3976:dbl, element #2=w3978:dbl, element #3=w3977:dbl)
                }
              }
            }
            frame "North east" {
              w3983 = 3
              n524 = case shown="2" w3983 {
                tunnel: [w3990 w3996 w4004 w4012 w4020 w4029 w4036 w4045] -> w3986
                tunnel: [w3992 w3998 w4006 w4013 w4022 w4031 w4038 w4047] -> w3985
                tunnel: [w3991 w3997 w4005 w4014 w4021 w4030 w4037 w4046] -> w3984
                tunnel: w3983 -> [w3994 w3999 w4007 w4015 w4023 w4028 w4039 w4044]
                tunnel: w3982 -> [w3987 w3995 w4003 w4011 w4019 w4027 w4035 w4043]
                frame 0, Default {
                  n525 = Index Array(array=w3987, index (row) #1=w3994, index (col) #1=0, index (row) #2=w3994, index (col) #2=1, index (row) #3=w3994, index (col) #3=2) -> (element #1=w3992:dbl, element #2=w3991:dbl, element #3=w3990:dbl)
                }
                frame 1 {
                  n526 = Index Array(array=w3995, index (row) #1=w3999, index (col) #1=0, index (row) #2=w3999, index (col) #2=1, index (row) #3=w3999, index (col) #3=2) -> (element #1=w3998:dbl, element #2=w3997:dbl, element #3=w3996:dbl)
                }
                frame 2 {
                  n527 = Index Array(array=w4003, index (row) #1=w4007, index (col) #1=0, index (row) #2=w4007, index (col) #2=1, index (row) #3=w4007, index (col) #3=2) -> (element #1=w4006:dbl, element #2=w4005:dbl, element #3=w4004:dbl)
                }
                frame 3 {
                  n528 = Index Array(array=w4011, index (row) #1=w4015, index (col) #1=0, index (row) #2=w4015, index (col) #2=1, index (row) #3=w4015, index (col) #3=2) -> (element #1=w4013:dbl, element #2=w4014:dbl, element #3=w4012:dbl)
                }
                frame 4 {
                  n529 = Index Array(array=w4019, index (row) #1=w4023, index (col) #1=0, index (row) #2=w4023, index (col) #2=1, index (row) #3=w4023, index (col) #3=2) -> (element #1=w4020:dbl, element #2=w4022:dbl, element #3=w4021:dbl)
                }
                frame 5 {
                  n530 = Index Array(array=w4027, index (row) #1=w4028, index (col) #1=0, index (row) #2=w4028, index (col) #2=1, index (row) #3=w4028, index (col) #3=2) -> (element #1=w4029:dbl, element #2=w4030:dbl, element #3=w4031:dbl)
                }
                frame 6 {
                  n531 = Index Array(array=w4035, index (row) #1=w4039, index (col) #1=0, index (row) #2=w4039, index (col) #2=1, index (row) #3=w4039, index (col) #3=2) -> (element #1=w4036:dbl, element #2=w4038:dbl, element #3=w4037:dbl)
                }
                frame 7 {
                  n532 = Index Array(array=w4043, index (row) #1=w4044, index (col) #1=0, index (row) #2=w4044, index (col) #2=1, index (row) #3=w4044, index (col) #3=2) -> (element #1=w4045:dbl, element #2=w4047:dbl, element #3=w4046:dbl)
                }
              }
            }
            frame "North west" {
              w4055 = 7
              n533 = case shown="2" w4055 {
                tunnel: [w4059 w4065 w4073 w4081 w4089 w4098 w4105 w4114] -> w4054
                tunnel: [w4061 w4067 w4075 w4082 w4091 w4100 w4107 w4116] -> w4053
                tunnel: [w4060 w4066 w4074 w4083 w4090 w4099 w4106 w4115] -> w4052
                tunnel: w4055 -> [w4063 w4068 w4076 w4084 w4092 w4097 w4108 w4113]
                tunnel: w4051 -> [w4056 w4064 w4072 w4080 w4088 w4096 w4104 w4112]
                frame 0, Default {
                  n534 = Index Array(array=w4056, index (row) #1=w4063, index (col) #1=0, index (row) #2=w4063, index (col) #2=1, index (row) #3=w4063, index (col) #3=2) -> (element #1=w4061:dbl, element #2=w4060:dbl, element #3=w4059:dbl)
                }
                frame 1 {
                  n535 = Index Array(array=w4064, index (row) #1=w4068, index (col) #1=0, index (row) #2=w4068, index (col) #2=1, index (row) #3=w4068, index (col) #3=2) -> (element #1=w4067:dbl, element #2=w4066:dbl, element #3=w4065:dbl)
                }
                frame 2 {
                  n536 = Index Array(array=w4072, index (row) #1=w4076, index (col) #1=0, index (row) #2=w4076, index (col) #2=1, index (row) #3=w4076, index (col) #3=2) -> (element #1=w4075:dbl, element #2=w4074:dbl, element #3=w4073:dbl)
                }
                frame 3 {
                  n537 = Index Array(array=w4080, index (row) #1=w4084, index (col) #1=0, index (row) #2=w4084, index (col) #2=1, index (row) #3=w4084, index (col) #3=2) -> (element #1=w4082:dbl, element #2=w4083:dbl, element #3=w4081:dbl)
                }
                frame 4 {
                  n538 = Index Array(array=w4088, index (row) #1=w4092, index (col) #1=0, index (row) #2=w4092, index (col) #2=1, index (row) #3=w4092, index (col) #3=2) -> (element #1=w4089:dbl, element #2=w4091:dbl, element #3=w4090:dbl)
                }
                frame 5 {
                  n539 = Index Array(array=w4096, index (row) #1=w4097, index (col) #1=0, index (row) #2=w4097, index (col) #2=1, index (row) #3=w4097, index (col) #3=2) -> (element #1=w4098:dbl, element #2=w4099:dbl, element #3=w4100:dbl)
                }
                frame 6 {
                  n540 = Index Array(array=w4104, index (row) #1=w4108, index (col) #1=0, index (row) #2=w4108, index (col) #2=1, index (row) #3=w4108, index (col) #3=2) -> (element #1=w4105:dbl, element #2=w4107:dbl, element #3=w4106:dbl)
                }
                frame 7 {
                  n541 = Index Array(array=w4112, index (row) #1=w4113, index (col) #1=0, index (row) #2=w4113, index (col) #2=1, index (row) #3=w4113, index (col) #3=2) -> (element #1=w4114:dbl, element #2=w4116:dbl, element #3=w4115:dbl)
                }
              }
            }
            frame "West" {
              w4124 = 6
              n542 = case shown="2" w4124 {
                tunnel: [w4128 w4134 w4142 w4150 w4158 w4167 w4174 w4183] -> w4121
                tunnel: [w4130 w4136 w4144 w4151 w4160 w4169 w4176 w4185] -> w4122
                tunnel: [w4129 w4135 w4143 w4152 w4159 w4168 w4175 w4184] -> w4120
                tunnel: w4124 -> [w4132 w4137 w4145 w4153 w4161 w4166 w4177 w4182]
                tunnel: w4123 -> [w4125 w4133 w4141 w4149 w4157 w4165 w4173 w4181]
                frame 0, Default {
                  n543 = Index Array(array=w4125, index (row) #1=w4132, index (col) #1=0, index (row) #2=w4132, index (col) #2=1, index (row) #3=w4132, index (col) #3=2) -> (element #1=w4130:dbl, element #2=w4129:dbl, element #3=w4128:dbl)
                }
                frame 1 {
                  n544 = Index Array(array=w4133, index (row) #1=w4137, index (col) #1=0, index (row) #2=w4137, index (col) #2=1, index (row) #3=w4137, index (col) #3=2) -> (element #1=w4136:dbl, element #2=w4135:dbl, element #3=w4134:dbl)
                }
                frame 2 {
                  n545 = Index Array(array=w4141, index (row) #1=w4145, index (col) #1=0, index (row) #2=w4145, index (col) #2=1, index (row) #3=w4145, index (col) #3=2) -> (element #1=w4144:dbl, element #2=w4143:dbl, element #3=w4142:dbl)
                }
                frame 3 {
                  n546 = Index Array(array=w4149, index (row) #1=w4153, index (col) #1=0, index (row) #2=w4153, index (col) #2=1, index (row) #3=w4153, index (col) #3=2) -> (element #1=w4151:dbl, element #2=w4152:dbl, element #3=w4150:dbl)
                }
                frame 4 {
                  n547 = Index Array(array=w4157, index (row) #1=w4161, index (col) #1=0, index (row) #2=w4161, index (col) #2=1, index (row) #3=w4161, index (col) #3=2) -> (element #1=w4158:dbl, element #2=w4160:dbl, element #3=w4159:dbl)
                }
                frame 5 {
                  n548 = Index Array(array=w4165, index (row) #1=w4166, index (col) #1=0, index (row) #2=w4166, index (col) #2=1, index (row) #3=w4166, index (col) #3=2) -> (element #1=w4167:dbl, element #2=w4168:dbl, element #3=w4169:dbl)
                }
                frame 6 {
                  n549 = Index Array(array=w4173, index (row) #1=w4177, index (col) #1=0, index (row) #2=w4177, index (col) #2=1, index (row) #3=w4177, index (col) #3=2) -> (element #1=w4174:dbl, element #2=w4176:dbl, element #3=w4175:dbl)
                }
                frame 7 {
                  n550 = Index Array(array=w4181, index (row) #1=w4182, index (col) #1=0, index (row) #2=w4182, index (col) #2=1, index (row) #3=w4182, index (col) #3=2) -> (element #1=w4183:dbl, element #2=w4185:dbl, element #3=w4184:dbl)
                }
              }
            }
            frame "East" {
              w4193 = 1
              n551 = case shown="2" w4193 {
                tunnel: [w4197 w4203 w4211 w4219 w4227 w4236 w4243 w4252] -> w4191
                tunnel: [w4199 w4205 w4213 w4220 w4229 w4238 w4245 w4254] -> w4190
                tunnel: [w4198 w4204 w4212 w4221 w4228 w4237 w4244 w4253] -> w4189
                tunnel: w4193 -> [w4201 w4206 w4214 w4222 w4230 w4235 w4246 w4251]
                tunnel: w4192 -> [w4194 w4202 w4210 w4218 w4226 w4234 w4242 w4250]
                frame 0, Default {
                  n552 = Index Array(array=w4194, index (row) #1=w4201, index (col) #1=0, index (row) #2=w4201, index (col) #2=1, index (row) #3=w4201, index (col) #3=2) -> (element #1=w4199:dbl, element #2=w4198:dbl, element #3=w4197:dbl)
                }
                frame 1 {
                  n553 = Index Array(array=w4202, index (row) #1=w4206, index (col) #1=0, index (row) #2=w4206, index (col) #2=1, index (row) #3=w4206, index (col) #3=2) -> (element #1=w4205:dbl, element #2=w4204:dbl, element #3=w4203:dbl)
                }
                frame 2 {
                  n554 = Index Array(array=w4210, index (row) #1=w4214, index (col) #1=0, index (row) #2=w4214, index (col) #2=1, index (row) #3=w4214, index (col) #3=2) -> (element #1=w4213:dbl, element #2=w4212:dbl, element #3=w4211:dbl)
                }
                frame 3 {
                  n555 = Index Array(array=w4218, index (row) #1=w4222, index (col) #1=0, index (row) #2=w4222, index (col) #2=1, index (row) #3=w4222, index (col) #3=2) -> (element #1=w4220:dbl, element #2=w4221:dbl, element #3=w4219:dbl)
                }
                frame 4 {
                  n556 = Index Array(array=w4226, index (row) #1=w4230, index (col) #1=0, index (row) #2=w4230, index (col) #2=1, index (row) #3=w4230, index (col) #3=2) -> (element #1=w4227:dbl, element #2=w4229:dbl, element #3=w4228:dbl)
                }
                frame 5 {
                  n557 = Index Array(array=w4234, index (row) #1=w4235, index (col) #1=0, index (row) #2=w4235, index (col) #2=1, index (row) #3=w4235, index (col) #3=2) -> (element #1=w4236:dbl, element #2=w4237:dbl, element #3=w4238:dbl)
                }
                frame 6 {
                  n558 = Index Array(array=w4242, index (row) #1=w4246, index (col) #1=0, index (row) #2=w4246, index (col) #2=1, index (row) #3=w4246, index (col) #3=2) -> (element #1=w4243:dbl, element #2=w4245:dbl, element #3=w4244:dbl)
                }
                frame 7 {
                  n559 = Index Array(array=w4250, index (row) #1=w4251, index (col) #1=0, index (row) #2=w4251, index (col) #2=1, index (row) #3=w4251, index (col) #3=2) -> (element #1=w4252:dbl, element #2=w4254:dbl, element #3=w4253:dbl)
                }
              }
            }
            frame "South" {
              w4262 = 2
              n560 = case shown="2" w4262 {
                tunnel: [w4266 w4272 w4280 w4288 w4296 w4305 w4312 w4321] -> w4261
                tunnel: [w4268 w4274 w4282 w4289 w4298 w4307 w4314 w4323] -> w4259
                tunnel: [w4267 w4273 w4281 w4290 w4297 w4306 w4313 w4322] -> w4258
                tunnel: w4262 -> [w4270 w4275 w4283 w4291 w4299 w4304 w4315 w4320]
                tunnel: w4260 -> [w4263 w4271 w4279 w4287 w4295 w4303 w4311 w4319]
                frame 0, Default {
                  n561 = Index Array(array=w4263, index (row) #1=w4270, index (col) #1=0, index (row) #2=w4270, index (col) #2=1, index (row) #3=w4270, index (col) #3=2) -> (element #1=w4268:dbl, element #2=w4267:dbl, element #3=w4266:dbl)
                }
                frame 1 {
                  n562 = Index Array(array=w4271, index (row) #1=w4275, index (col) #1=0, index (row) #2=w4275, index (col) #2=1, index (row) #3=w4275, index (col) #3=2) -> (element #1=w4274:dbl, element #2=w4273:dbl, element #3=w4272:dbl)
                }
                frame 2 {
                  n563 = Index Array(array=w4279, index (row) #1=w4283, index (col) #1=0, index (row) #2=w4283, index (col) #2=1, index (row) #3=w4283, index (col) #3=2) -> (element #1=w4282:dbl, element #2=w4281:dbl, element #3=w4280:dbl)
                }
                frame 3 {
                  n564 = Index Array(array=w4287, index (row) #1=w4291, index (col) #1=0, index (row) #2=w4291, index (col) #2=1, index (row) #3=w4291, index (col) #3=2) -> (element #1=w4289:dbl, element #2=w4290:dbl, element #3=w4288:dbl)
                }
                frame 4 {
                  n565 = Index Array(array=w4295, index (row) #1=w4299, index (col) #1=0, index (row) #2=w4299, index (col) #2=1, index (row) #3=w4299, index (col) #3=2) -> (element #1=w4296:dbl, element #2=w4298:dbl, element #3=w4297:dbl)
                }
                frame 5 {
                  n566 = Index Array(array=w4303, index (row) #1=w4304, index (col) #1=0, index (row) #2=w4304, index (col) #2=1, index (row) #3=w4304, index (col) #3=2) -> (element #1=w4305:dbl, element #2=w4306:dbl, element #3=w4307:dbl)
                }
                frame 6 {
                  n567 = Index Array(array=w4311, index (row) #1=w4315, index (col) #1=0, index (row) #2=w4315, index (col) #2=1, index (row) #3=w4315, index (col) #3=2) -> (element #1=w4312:dbl, element #2=w4314:dbl, element #3=w4313:dbl)
                }
                frame 7 {
                  n568 = Index Array(array=w4319, index (row) #1=w4320, index (col) #1=0, index (row) #2=w4320, index (col) #2=1, index (row) #3=w4320, index (col) #3=2) -> (element #1=w4321:dbl, element #2=w4323:dbl, element #3=w4322:dbl)
                }
              }
            }
            frame "South west" {
              w4331 = 4
              n569 = case shown="2" w4331 {
                tunnel: [w4335 w4341 w4349 w4357 w4365 w4374 w4381 w4390] -> w4329
                tunnel: [w4337 w4343 w4351 w4358 w4367 w4376 w4383 w4392] -> w4328
                tunnel: [w4336 w4342 w4350 w4359 w4366 w4375 w4382 w4391] -> w4327
                tunnel: w4331 -> [w4339 w4344 w4352 w4360 w4368 w4373 w4384 w4389]
                tunnel: w4330 -> [w4332 w4340 w4348 w4356 w4364 w4372 w4380 w4388]
                frame 0, Default {
                  n570 = Index Array(array=w4332, index (row) #1=w4339, index (col) #1=0, index (row) #2=w4339, index (col) #2=1, index (row) #3=w4339, index (col) #3=2) -> (element #1=w4337:dbl, element #2=w4336:dbl, element #3=w4335:dbl)
                }
                frame 1 {
                  n571 = Index Array(array=w4340, index (row) #1=w4344, index (col) #1=0, index (row) #2=w4344, index (col) #2=1, index (row) #3=w4344, index (col) #3=2) -> (element #1=w4343:dbl, element #2=w4342:dbl, element #3=w4341:dbl)
                }
                frame 2 {
                  n572 = Index Array(array=w4348, index (row) #1=w4352, index (col) #1=0, index (row) #2=w4352, index (col) #2=1, index (row) #3=w4352, index (col) #3=2) -> (element #1=w4351:dbl, element #2=w4350:dbl, element #3=w4349:dbl)
                }
                frame 3 {
                  n573 = Index Array(array=w4356, index (row) #1=w4360, index (col) #1=0, index (row) #2=w4360, index (col) #2=1, index (row) #3=w4360, index (col) #3=2) -> (element #1=w4358:dbl, element #2=w4359:dbl, element #3=w4357:dbl)
                }
                frame 4 {
                  n574 = Index Array(array=w4364, index (row) #1=w4368, index (col) #1=0, index (row) #2=w4368, index (col) #2=1, index (row) #3=w4368, index (col) #3=2) -> (element #1=w4365:dbl, element #2=w4367:dbl, element #3=w4366:dbl)
                }
                frame 5 {
                  n575 = Index Array(array=w4372, index (row) #1=w4373, index (col) #1=0, index (row) #2=w4373, index (col) #2=1, index (row) #3=w4373, index (col) #3=2) -> (element #1=w4374:dbl, element #2=w4375:dbl, element #3=w4376:dbl)
                }
                frame 6 {
                  n576 = Index Array(array=w4380, index (row) #1=w4384, index (col) #1=0, index (row) #2=w4384, index (col) #2=1, index (row) #3=w4384, index (col) #3=2) -> (element #1=w4381:dbl, element #2=w4383:dbl, element #3=w4382:dbl)
                }
                frame 7 {
                  n577 = Index Array(array=w4388, index (row) #1=w4389, index (col) #1=0, index (row) #2=w4389, index (col) #2=1, index (row) #3=w4389, index (col) #3=2) -> (element #1=w4390:dbl, element #2=w4392:dbl, element #3=w4391:dbl)
                }
              }
            }
            frame "South east" {
              w4400 = 0
              n578 = case shown="2" w4400 {
                tunnel: [w4404 w4410 w4418 w4426 w4434 w4443 w4450 w4459] -> w4399
                tunnel: [w4406 w4412 w4420 w4427 w4436 w4445 w4452 w4461] -> w4398
                tunnel: [w4405 w4411 w4419 w4428 w4435 w4444 w4451 w4460] -> w4397
                tunnel: w4400 -> [w4408 w4413 w4421 w4429 w4437 w4442 w4453 w4458]
                tunnel: w4396 -> [w4401 w4409 w4417 w4425 w4433 w4441 w4449 w4457]
                frame 0, Default {
                  n579 = Index Array(array=w4401, index (row) #1=w4408, index (col) #1=0, index (row) #2=w4408, index (col) #2=1, index (row) #3=w4408, index (col) #3=2) -> (element #1=w4406:dbl, element #2=w4405:dbl, element #3=w4404:dbl)
                }
                frame 1 {
                  n580 = Index Array(array=w4409, index (row) #1=w4413, index (col) #1=0, index (row) #2=w4413, index (col) #2=1, index (row) #3=w4413, index (col) #3=2) -> (element #1=w4412:dbl, element #2=w4411:dbl, element #3=w4410:dbl)
                }
                frame 2 {
                  n581 = Index Array(array=w4417, index (row) #1=w4421, index (col) #1=0, index (row) #2=w4421, index (col) #2=1, index (row) #3=w4421, index (col) #3=2) -> (element #1=w4420:dbl, element #2=w4419:dbl, element #3=w4418:dbl)
                }
                frame 3 {
                  n582 = Index Array(array=w4425, index (row) #1=w4429, index (col) #1=0, index (row) #2=w4429, index (col) #2=1, index (row) #3=w4429, index (col) #3=2) -> (element #1=w4427:dbl, element #2=w4428:dbl, element #3=w4426:dbl)
                }
                frame 4 {
                  n583 = Index Array(array=w4433, index (row) #1=w4437, index (col) #1=0, index (row) #2=w4437, index (col) #2=1, index (row) #3=w4437, index (col) #3=2) -> (element #1=w4434:dbl, element #2=w4436:dbl, element #3=w4435:dbl)
                }
                frame 5 {
                  n584 = Index Array(array=w4441, index (row) #1=w4442, index (col) #1=0, index (row) #2=w4442, index (col) #2=1, index (row) #3=w4442, index (col) #3=2) -> (element #1=w4443:dbl, element #2=w4444:dbl, element #3=w4445:dbl)
                }
                frame 6 {
                  n585 = Index Array(array=w4449, index (row) #1=w4453, index (col) #1=0, index (row) #2=w4453, index (col) #2=1, index (row) #3=w4453, index (col) #3=2) -> (element #1=w4450:dbl, element #2=w4452:dbl, element #3=w4451:dbl)
                }
                frame 7 {
                  n586 = Index Array(array=w4457, index (row) #1=w4458, index (col) #1=0, index (row) #2=w4458, index (col) #2=1, index (row) #3=w4458, index (col) #3=2) -> (element #1=w4459:dbl, element #2=w4461:dbl, element #3=w4460:dbl)
                }
              }
            }
          }
        }
      }
      "Time" <- w8
      "Left" <- w7
      "Right" <- w6
      "left sped/right speed/time" <- w5
    }
    frame #1 {
      n587 = flat-sequence {
        tunnel: "error in (no error)" -> [w4477]
        tunnel: "error in (no error) 2" -> [w4476]
        tunnel: [w4475] -> w4468
        tunnel: [w4474] -> w4466
        tunnel: w4468 -> [w4570]
        tunnel: [w4568] -> w4467
        tunnel: w4466 -> [w4569]
        tunnel: [w4567] -> w4465
        tunnel: w4467 -> [w4667]
        tunnel: w4465 -> [w4666]
        tunnel: [w4665] -> w4470
        tunnel: [w4664] -> w4469
        frame #0 {
          n588 = local read "Time"() -> (w4473:i32)
          n589 = node-c288(w4473) -> (w4479:T1)  [unwired: 3 in]
          n590 = timed-loop {
            tunnel: w4477 -> [w4490]
            tunnel: [w4489] -> w4474
            tunnel: w4476 -> [w4486]
            tunnel: [w4485] -> w4475
            timing: w4479 -> [_]
            timing-out: [_] -> w4478
            i -> [w4484]
            stop <- w4482 stop-if-true
            n591 = node-c288() -> ()  [unwired: 1 in, 1 out]
            n592 = Equal?(x=w4484, y=1) -> (x = y?=w4482:bool)
            n593 = local read "Left"() -> (w4481:dbl)
            n594 = local read "Right"() -> (w4480:dbl)
            n595 = xnode "PWM 2"("Duty Cycle"=w4481, "Frequency [Hz]"=500, "error in (no error)"=w4486) -> ("error out"=w4485:errorcluster)
            n596 = xnode "PWM"("Duty Cycle"=w4480, "Frequency [Hz]"=500, "error in (no error)"=w4490) -> ("error out"=w4489:errorcluster)
            n597 = node-c288() -> ()  [unwired: 1 in, 1 out]
          }
          n598 = node-c288(w4478) -> ()  [unwired: 1 out]
        }
        frame #1 {
          n599 = node-c288(1500) -> (w4573:T1)  [unwired: 3 in]
          n600 = timed-loop {
            tunnel: w4569 -> [w4584]
            tunnel: [w4583] -> w4567
            tunnel: w4570 -> [w4580]
            tunnel: [w4579] -> w4568
            timing: w4573 -> [_]
            timing-out: [_] -> w4572
            i -> [w4576]
            stop <- w4574 stop-if-true
            n601 = node-c288() -> ()  [unwired: 1 in, 1 out]
            n602 = Equal?(x=w4576, y=1) -> (x = y?=w4574:bool)
            n603 = xnode "PWM 5"("Duty Cycle"=0.65 ("Numeric 2"), "Frequency [Hz]"=500, "error in (no error)"=w4580) -> ("error out"=w4579:errorcluster)
            n604 = xnode "PWM 6"("Duty Cycle"=0.65 ("Numeric"), "Frequency [Hz]"=500, "error in (no error)"=w4584) -> ("error out"=w4583:errorcluster)
            n605 = node-c288() -> ()  [unwired: 1 in, 1 out]
          }
          n606 = node-c288(w4572) -> ()  [unwired: 1 out]
        }
        frame #2 {
          n607 = xnode "PWM 4"("Duty Cycle"=0.75, "Frequency [Hz]"=500, "error in (no error)"=w4667) -> ("error out"=w4665:errorcluster)
          n608 = xnode "PWM 3"("Duty Cycle"=0.75, "Frequency [Hz]"=500, "error in (no error)"=w4666) -> ("error out"=w4664:errorcluster)
        }
      }
      "error out 2" <- w4469
      "error out 3" <- w4470
    }
  }
